vi "SISE-Analyser110.vi"() -> ()   [LabVIEW 2024]
uses:
  <vilib>/Analysis/NI_AALPro.lvlib
panel:
  in  "Ion conc. ch1 (mM) 2":dbl
  in  "Main Tab Control":T1(tab)
  out "Event marks":string
  in  "Raw data file in":path
  out "Trace length":dbl
  out "# of traces":dbl
  out "Trace #":dbl
  in  "Scroll back":bool
  in  "Step back":bool
  in  "Step forward":bool
  in  "Scroll forward":bool
  in  "Module selection view data":enum16{"Load data", "Scroll data"}(ring)
  out "Load data":bool
  in  "Scroll speed":dbl(slide)=10.000000000000002 scale=1.0..100.0
  out "Scroll data":bool
  out "SISE 1 channel":bool
  out "Voltage 2 channel":bool
  out "Voltage 1 channel":bool
  out "SISE 2 channel":bool
  out "Scan distance, µm":dbl
  out "Scan angle, degrees":dbl
  out "Record period (single track), s):":dbl
  out "Position probe":cluster{dbl[], dbl[]}[](graph)
  in  "?":T2(tab)
  out "Vprobe SISE 1":cluster{dbl[], dbl[]}[](graph)
  out "Vprobe SISE 2":cluster{dbl[], dbl[]}[](graph)
  out "Vprobe V 1":cluster{dbl[], dbl[]}[](graph)
  out "Vprobe V 2":cluster{dbl[], dbl[]}[](graph)
  in  "?":enum32{"dV SISE 1", "dV SISE 2"}(tab)
  out "deltaV SISE 1":cluster{dbl[], "Best Linear Fit":dbl[]}[](graph)
  out "deltaV SISE 2":cluster{dbl[], "Best Linear Fit":dbl[]}[](graph)
  in  "Start fit (% of rec. period)":dbl(slide)=50.0 scale=0.0..100.0
  in  "TC 3":T3(tab)
  in  "Range limit\nS1.1 (mV)":dbl(slide)=200.0 min=0.0 max=600.0 scale=0.2..600.0
  in  "Base line\nS1.1 (mV)":dbl(slide) scale=-300.0..300.0
  in  "Range limit\nS1.2 mV":dbl(slide)=30.0 scale=0.03..300.0
  in  "Base line \nS1.2 (mV)":dbl(slide) scale=-15.0..15.0
  out "dV-SISE channel 1":cluster{dbl[], dbl[]}[](graph)
  out "V-SISE channel 1":cluster{dbl[], dbl[]}[](graph)
  out "dV-SISE channel 2":cluster{dbl[], dbl[]}[](graph)
  in  "Base line \nS2.2 (mV)":dbl(slide) scale=-15.0..15.0
  in  "Range limit\nS2.2 (mV)":dbl(slide)=30.0 scale=0.03..300.0
  out "V-SISE channel 2":cluster{dbl[], dbl[]}[](graph)
  in  "Range limit\nS1.1 (mV) 2":dbl(slide)=200.0 min=0.0 max=600.0 scale=0.2..600.0
  in  "Base line\nS1.1 (mV)":dbl(slide) scale=-300.0..300.0
  out "Voltage channel 1":cluster{dbl[], dbl[]}[](graph)
  in  "Base line\nV1 (V)":dbl(slide) scale=-300.0..300.0
  in  "Range limit\nV1 (V)":dbl(slide)=200.0 min=0.0 max=600.0 scale=0.2..600.0
  in  "Base line\nV2 (V)":dbl(slide) scale=-300.0..300.0
  in  "Range limit\nV2 (V)":dbl(slide)=200.0 min=0.0 max=600.0 scale=0.2..600.0
  out "Voltage channel 2":cluster{dbl[], dbl[]}[](graph)
  in  "Zoom from end":dbl(slide)=100.0 scale=0.0..100.0
  in  "Zoom from start":dbl(slide) scale=0.0..100.0
  in  "Calibration-channel SISE1/2":enum32{"SISE channel 1", "SISE channel 2"}(tab)
  out "Update graphs ch1":bool
  in  "Module selection (Calibration window channel 1)":T4(ring)
  out "Anal. method ch1":bool
  out "Calibration ch1":bool
  out "Slope ch1":dbl
  out "Intercept ch1":dbl
  out "?":cluster{dbl[], dbl[]}[](graph)
  out "Point #":dbl[](array[numeric])=[1.0, 2.0, 3.0, 4.0, 5.0]
  in  "Array in":dbl[][](array[numeric])
  out "Geometry ch1":bool caption="Geometry"
  out "Corrected \ndistance ch1":dbl caption="Corrected \ndistance"
  in  "Tab Control Geo 1":enum32{"flat surface", "cylinder", "sphere"}(tab)
  in  "Scan Distance  Flat (µm) 1":dbl
  in  "Scan distance cyl. (µm) 1":dbl caption="Scan distance cyl. (µm)"
  in  "Radius of object cyl. (µm) 1":dbl caption="Radius of object cyl. (µm)"
  in  "Minimum distance to object cyl. (µm) 1":dbl caption="Minimum distance to object cyl. (µm)"
  in  "Minimum distance to object sphere (µm) 1":dbl caption="Minimum distance to object sphere (µm)"
  in  "Radius of object sphere (µm) 1":dbl caption="Radius of object sphere (µm)"
  in  "Scan distance sphere (µm) 1":dbl caption="Scan distance sphere (µm)"
  out "Ion conc. SISE channel 1":cluster{dbl[], dbl[]}[](graph)
  in  "Range limit\nS1.3 (mM)":dbl(slide)=200.0 min=0.0 max=600.0 scale=1e-08..100.0
  in  "Base line\nS1.3 (mM)":dbl(slide) scale=-10.0..10.0
  out "Ion flux SISE channel 1":cluster{dbl[], dbl[]}[](graph)
  in  "Base line \nS1.4":dbl(slide) scale=-15.0..15.0
  in  "Range limit\nS1.4":dbl(slide)=1080.8651170969697 scale=0.03..3000.0
  out "?":string
  in  "Bildlaufleiste":i32(c297)
  in  "Zoom from end (Cal. modul) ch1":dbl(slide)=100.0 caption="Zoom from end" scale=0.0..100.0
  in  "Zoom from start (Cal. modul) ch1":dbl(slide) caption="Zoom from start" scale=0.0..100.0
  in  "Analysis method (Calibration window channel 1)":enum32{"Chem. potential", "Diff. gradient"}(tab)
  in  "Ion conc. ch1 (mM)":dbl
  out "Valence ch1":dbl
  out "Ion mobilty ch1":dbl
  out "Diff. coeff. ch1":dbl
  in  "Ion Species ch1":u16(ring) items=["none", "H+", "K+", "NH4+", "Na+", "Cl-", "NO3-", "Ca2+", "Mg2+"]
  out "Update graphs ch2":bool
  out "Calibration ch2":bool
  out "Slope ch2":dbl
  out "Intercept ch2":dbl
  out "?":cluster{dbl[], dbl[]}[](graph)
  out "Point # 2":dbl[](array[numeric])=[1.0, 2.0, 3.0, 4.0, 5.0]
  in  "Array in 2":dbl[][](array[numeric])
  out "Geometry 2":bool caption="Geometry"
  out "Corrected \ndistance ch2":dbl caption="Corrected\ndistance"
  in  "Tab Control Geo 2":enum32{"flat surface", "cylinder", "sphere"}(tab)
  in  "Scan Distance  Flat (µm) 2":dbl caption="Scan Distance  Flat (µm)"
  in  "Scan distance cyl. (µm) 2":dbl caption="Scan distance cyl. (µm)"
  in  "Radius of object cyl. (µm) 2":dbl caption="Radius of object cyl. (µm)"
  in  "Minimum distance to object cyl. (µm) 2":dbl caption="Minimum distance to object cyl. (µm)"
  in  "Minimum distance to object sphere (µm) 2":dbl caption="Minimum distance to object sphere (µm)"
  in  "Radius of object sphere (µm) 2":dbl caption="Radius of object sphere (µm)"
  in  "Scan distance sphere (µm) 2":dbl caption="Scan distance sphere (µm)"
  in  "Bildlaufleiste 2":i32(c297)
  out "?":string
  out "Ion conc. SISE channel 2":cluster{dbl[], dbl[]}[](graph)
  in  "Range limit\nS2.3 (mM)":dbl(slide)=200.0 min=0.0 max=600.0 scale=1e-08..100.0
  in  "Base line\nS2.3 (mM)":dbl(slide) scale=-10.0..10.0
  out "Ion flux SISE channel 2":cluster{dbl[], dbl[]}[](graph)
  in  "Base line \nS2.4":dbl(slide) scale=-15.0..15.0
  in  "Range limit\nS2.4":dbl(slide)=1021.2709042717592 scale=0.03..3000.0
  in  "Module selection (Calibration window channel 2)":T4(ring)
  in  "Zoom from end (Cal. modul) 2":dbl(slide)=100.0 caption="Zoom from end" scale=0.0..100.0
  in  "Zoom from start (Cal. modul) 2":dbl(slide) caption="Zoom from start" scale=0.0..100.0
  in  "Analysis method (Calibration window channel 2)":enum32{"Chem. potential", "Diff. gradient"}(tab)
  in  "Ion conc. ch2 (mM)":dbl
  out "Valence ch2":dbl
  out "Ion mobilty ch2":dbl
  out "Diff. coeff. ch2":dbl
  in  "Ion Species ch2":u16(ring) items=["none", "H+", "K+", "NH4+", "Na+", "Cl-", "NO3-", "Ca2+", "Mg2+"]
  out "Anal. method ch2":bool
  in  "SISE channel selection (buffer corr.)":T5(tab)
  out "Tab Control":enum32{"Chem. potential", "Diff. gradient"}(tab)
  out "Buffer Mobilty ch1":dbl
  out "Diff. coeff. buffer ch1":dbl
  in  "Module selection ch1 (buffer corr.)":T6(ring)
  out "Buffer species ch1":bool
  out "Buffer conc. ch1":bool
  in  "Select buffer ch1":T7(ring)
  out "pKs ch1":dbl
  in  "Buffer conc. ch1 (mM)":dbl
  out "?":string
  in  "Bildlaufleiste 3":i32(c297)
  out "Ion flux (buffer corr.) SISE channel 1":cluster{dbl[], dbl[]}[](graph)
  in  "Base line \nS2.4 3":dbl(slide) scale=-15.0..15.0
  in  "Range limit\nS2.4 3":dbl(slide)=30.0 scale=0.01..10000.0
  out "Update graphs (buffer corr.) ch1":bool
  in  "Zoom from end (Buffer corr. modul) ch1":dbl(slide)=100.0 caption="Zoom from end" scale=0.0..100.0
  in  "Zoom from start (Buffer corr. modul) ch1":dbl(slide) caption="Zoom from start" scale=0.0..100.0
  in  "Module selection ch2 (buffer corr.)":T6(ring)
  out "Buffer species ch2":bool
  out "Buffer conc. ch2":bool
  in  "Buffer conc. ch2 (mM)":dbl
  in  "Range limit\nS2.4 2":dbl(slide)=30.0 scale=0.01..10000.0
  in  "Base line \nS2.4 2":dbl(slide) scale=-15.0..15.0
  out "Ion flux (buffer corr.) SISE channel 2":cluster{dbl[], dbl[]}[](graph)
  out "Update graphs (buffer corr.) ch2":bool
  out "?":string
  in  "Bildlaufleiste 4":i32(c297)
  in  "Zoom from start (Buffer corr. modul) ch2":dbl(slide) caption="Zoom from start" scale=0.0..100.0
  in  "Zoom from end (Buffer corr. modul) ch2":dbl(slide)=100.0 caption="Zoom from end" scale=0.0..100.0
  in  "Select buffer ch 2":T7(ring)
  out "pKs ch2":dbl
  out "Tab Control 2":enum32{"Chem. potential", "Diff. gradient"}(tab)
  out "Buffer Mobilty ch2":dbl
  out "Diff. coeff. buffer ch2":dbl
  out "Next data file/exit program":bool
  in  "Exit program":bool
  out "Create analysis file":bool
  out "Indicate output":bool[](array[boolean])
  in  "Select output":bool[](array[boolean])=[TRUE, TRUE, TRUE, TRUE, TRUE, TRUE, TRUE, TRUE, TRUE, TRUE, TRUE, TRUE, TRUE, TRUE]
  in  "Analysis output file":path
  out "Raw data file":path
  out "Cluster 3":cluster{string[], bool[]}
  in  "Next data file":bool
  in  "Save data":bool
  out "Save analyses file":bool
  in  "Module selection Save Data":T8(ring)
  # "Event marks"
  # "Point (#)       Conc. (mM )      Vm (mV)"
  # "Event marks"
  # "Point (#)       Conc. (mM )      Vm (mV)"
  # "Event marks"
  # "Event marks"
  # "Output signals available                                                               Select output signals"
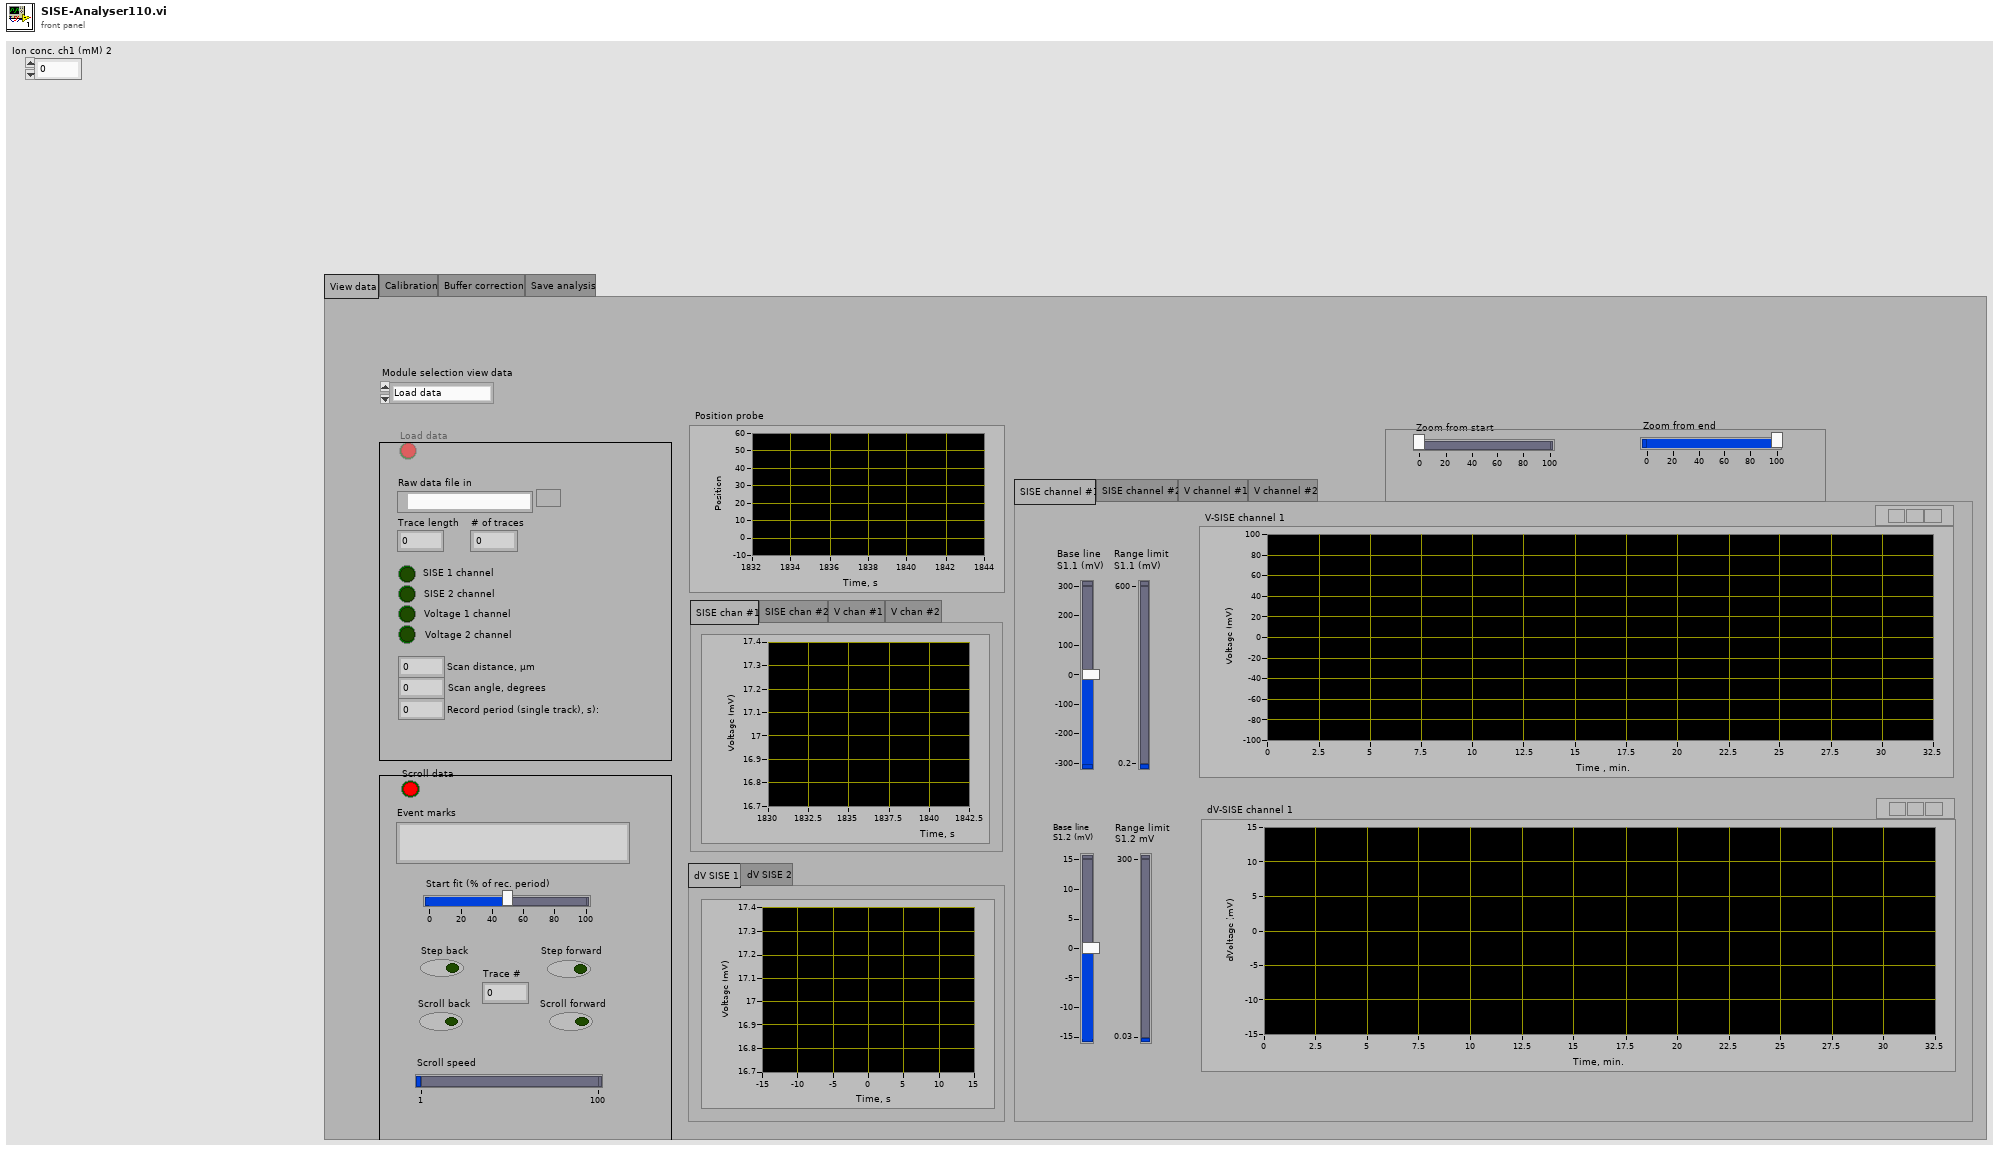
[diagram p1: front panel]
types:
  T1 = enum32{"View data", "Calibration", "Buffer correction", "Save analysis"}
  T2 = enum32{"SISE chan #1", "SISE chan #2", "V chan #1", "V chan #2"}
  T3 = enum32{"SISE channel #1", "SISE channel #2", "V channel #1", "V channel #2"}
  T4 = enum16{"Analysis method", "Calibrate", "Geometry", "Update graphs"}
  T5 = enum32{"SISE channel 1, buffer corr.", "SISE channel 2, buffer corr."}
  T6 = enum16{"Buffer species", "Buffer conc.", "Update graphs"}
  T7 = enum16{"none", "Mes", "Malate (pH 5)", "Citrate (pH 5)", "TRIS", "HEPES"}
  T8 = enum16{"Create analysis file", "Save data", "New/stop analysis"}
  T9 = enum8{"Enabled", "Disabled", "Disabled and Grayed Out"}
  T10 = enum16{"open", "replace", "create", "open or create", "replace or create", "replace or create with confirmation"}
  T11 = enum32{"Chem. potential", "Diff. gradient", "empty loop"}
  T12 = cluster{path, "Referenz (Ausgang)":refnum<file>, bool, i32, string}
  T13 = cluster{path, "Referenz (Ausgang)":refnum<file>, bool, i32, string}[]
  T14 = cluster{"Raw data file in":path, "refnum out":refnum<file>, "status":bool, "code":i32, "source":string}
  T15 = cluster{bool[], dbl[][], dbl[], cluster{string[], bool[]}, dbl[][], cluster{dbl, string}[]}
  T16 = cluster{dbl[], dbl[], "Best Linear Fit":dbl[], dbl[], dbl[]}
  T17 = cluster{"Array (Ausgang)":dbl[], "Array (Ausgang)":dbl[]}
  T18 = cluster{"Array (Ausgang)":dbl[], "Array (Ausgang)":dbl[]}[]
  T19 = cluster{"dup path":path, "refnum":refnum<file>, "status":bool, "code":i32, "source":string}
  T20 = cluster{bool[], dbl[][], dbl[], cluster{dbl, string}[]}
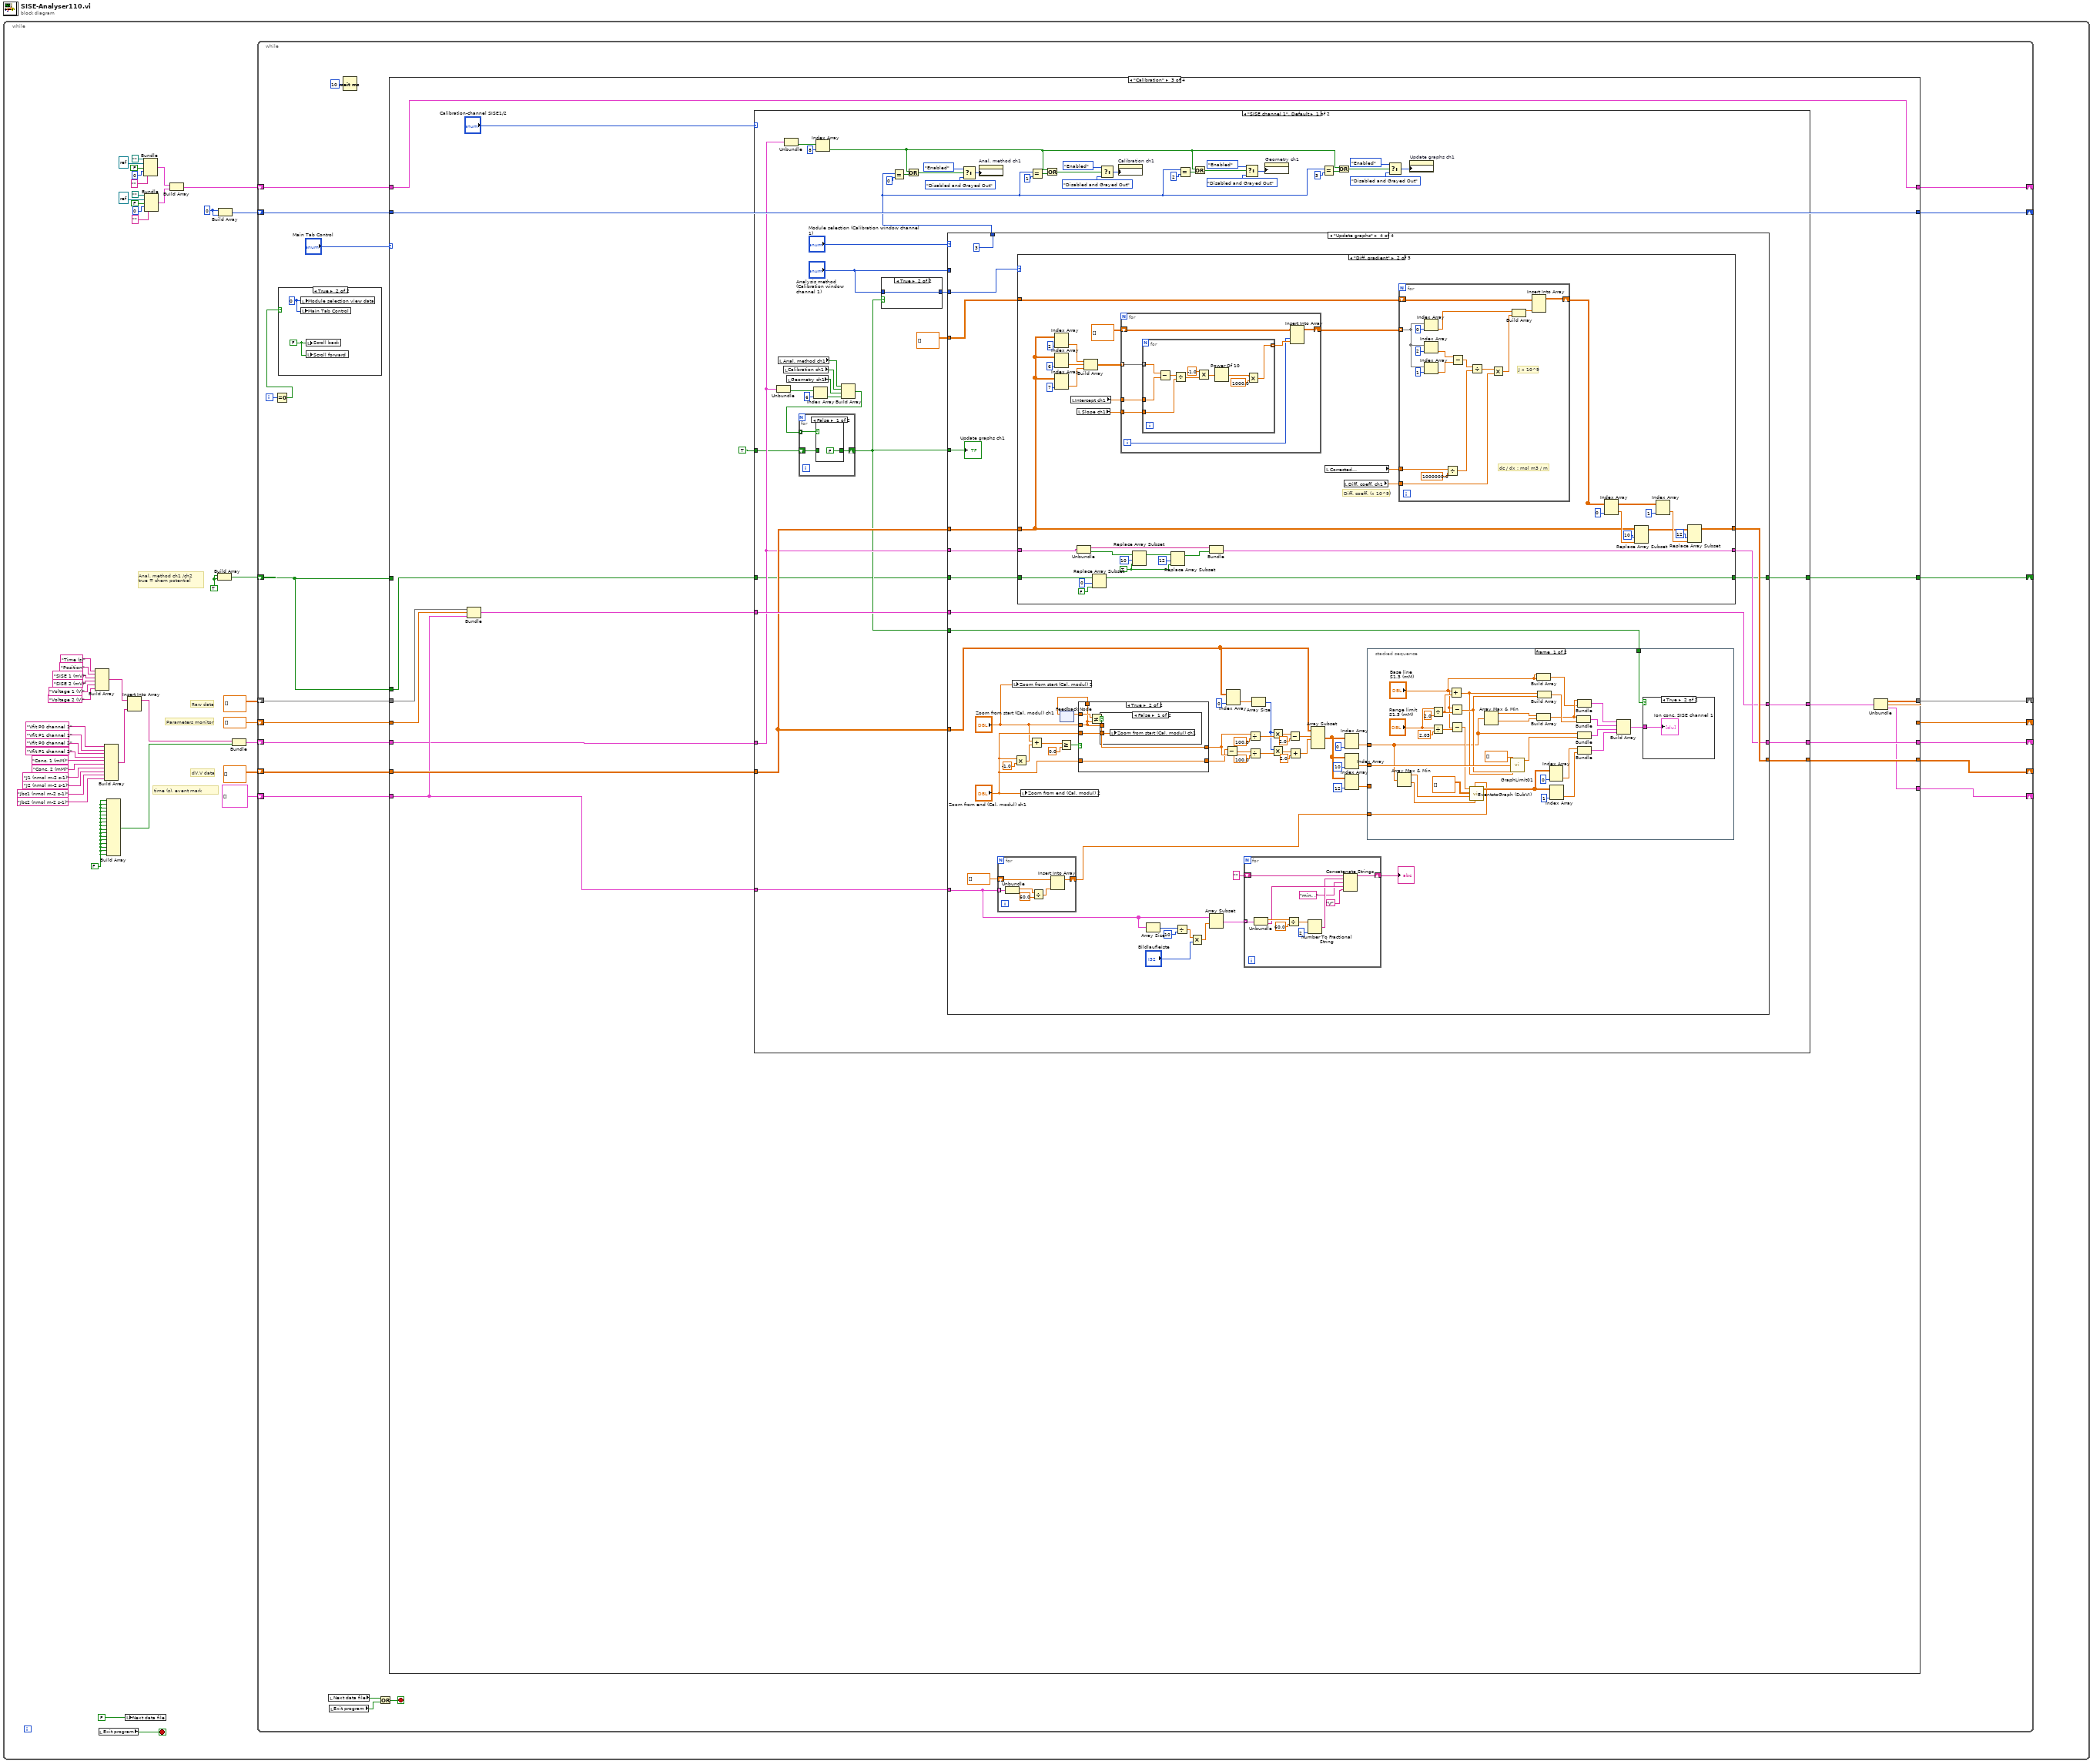
[diagram p0: block diagram]
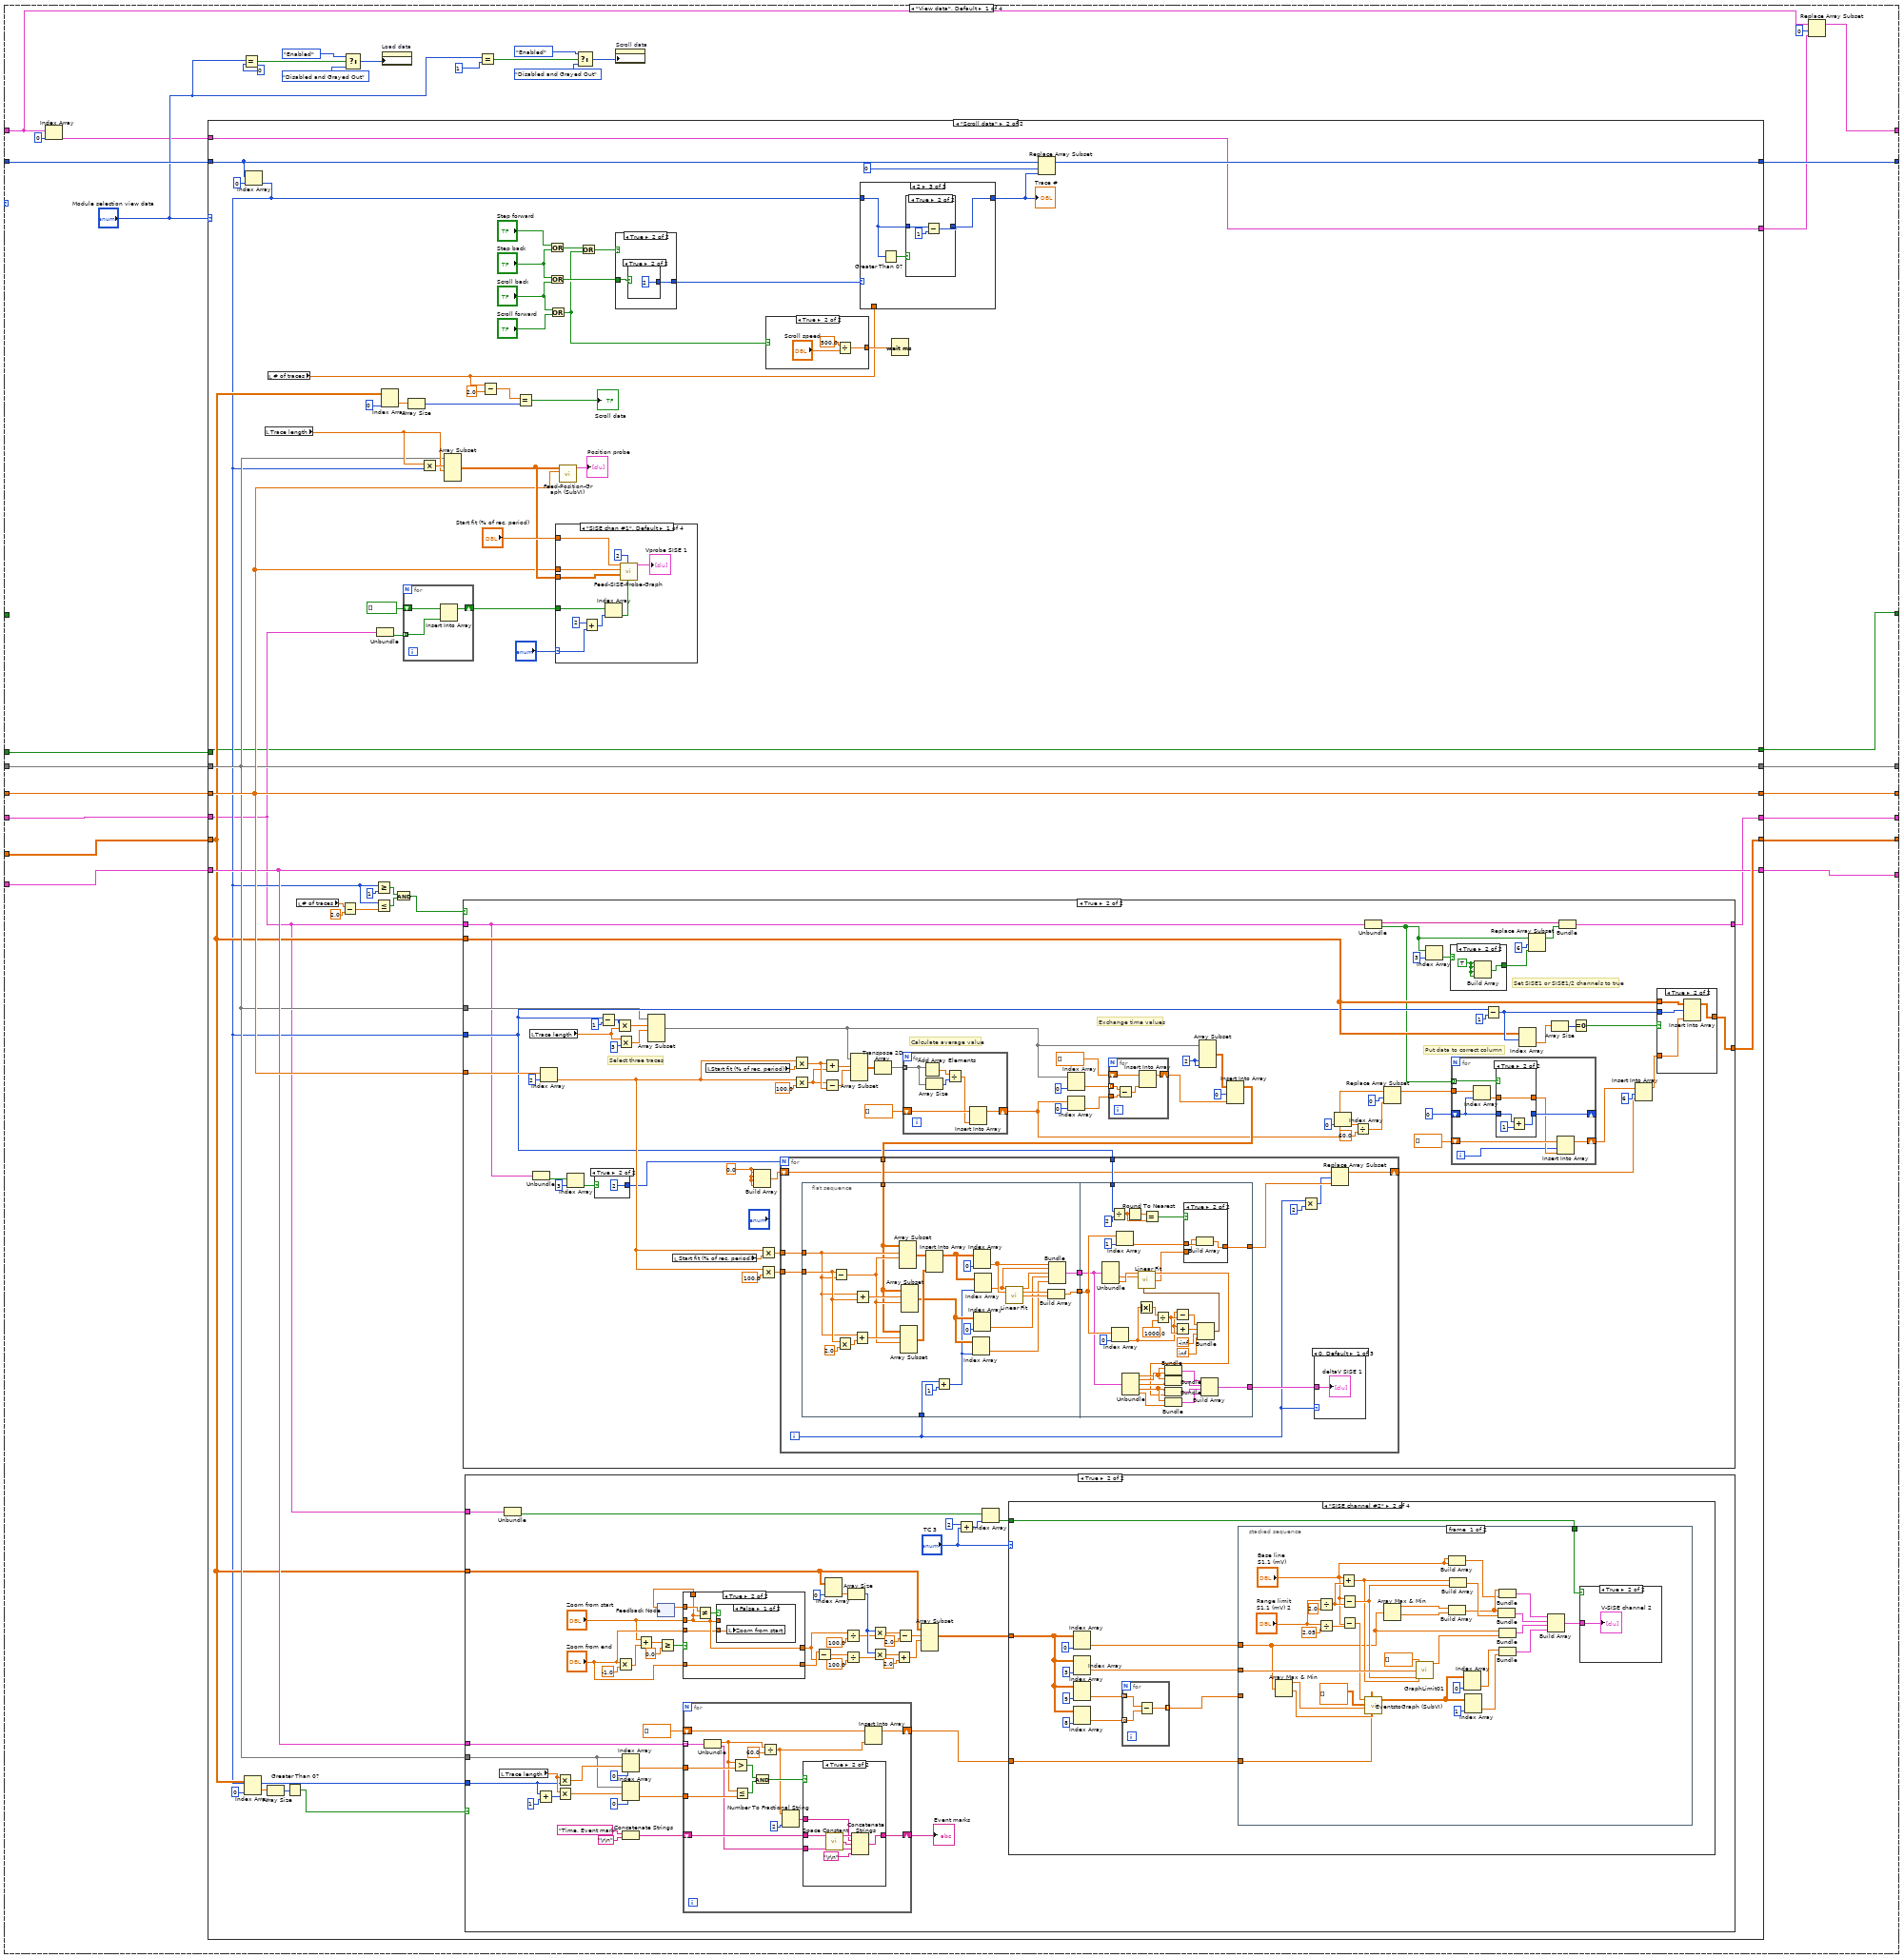
[diagram p3: hidden frame]
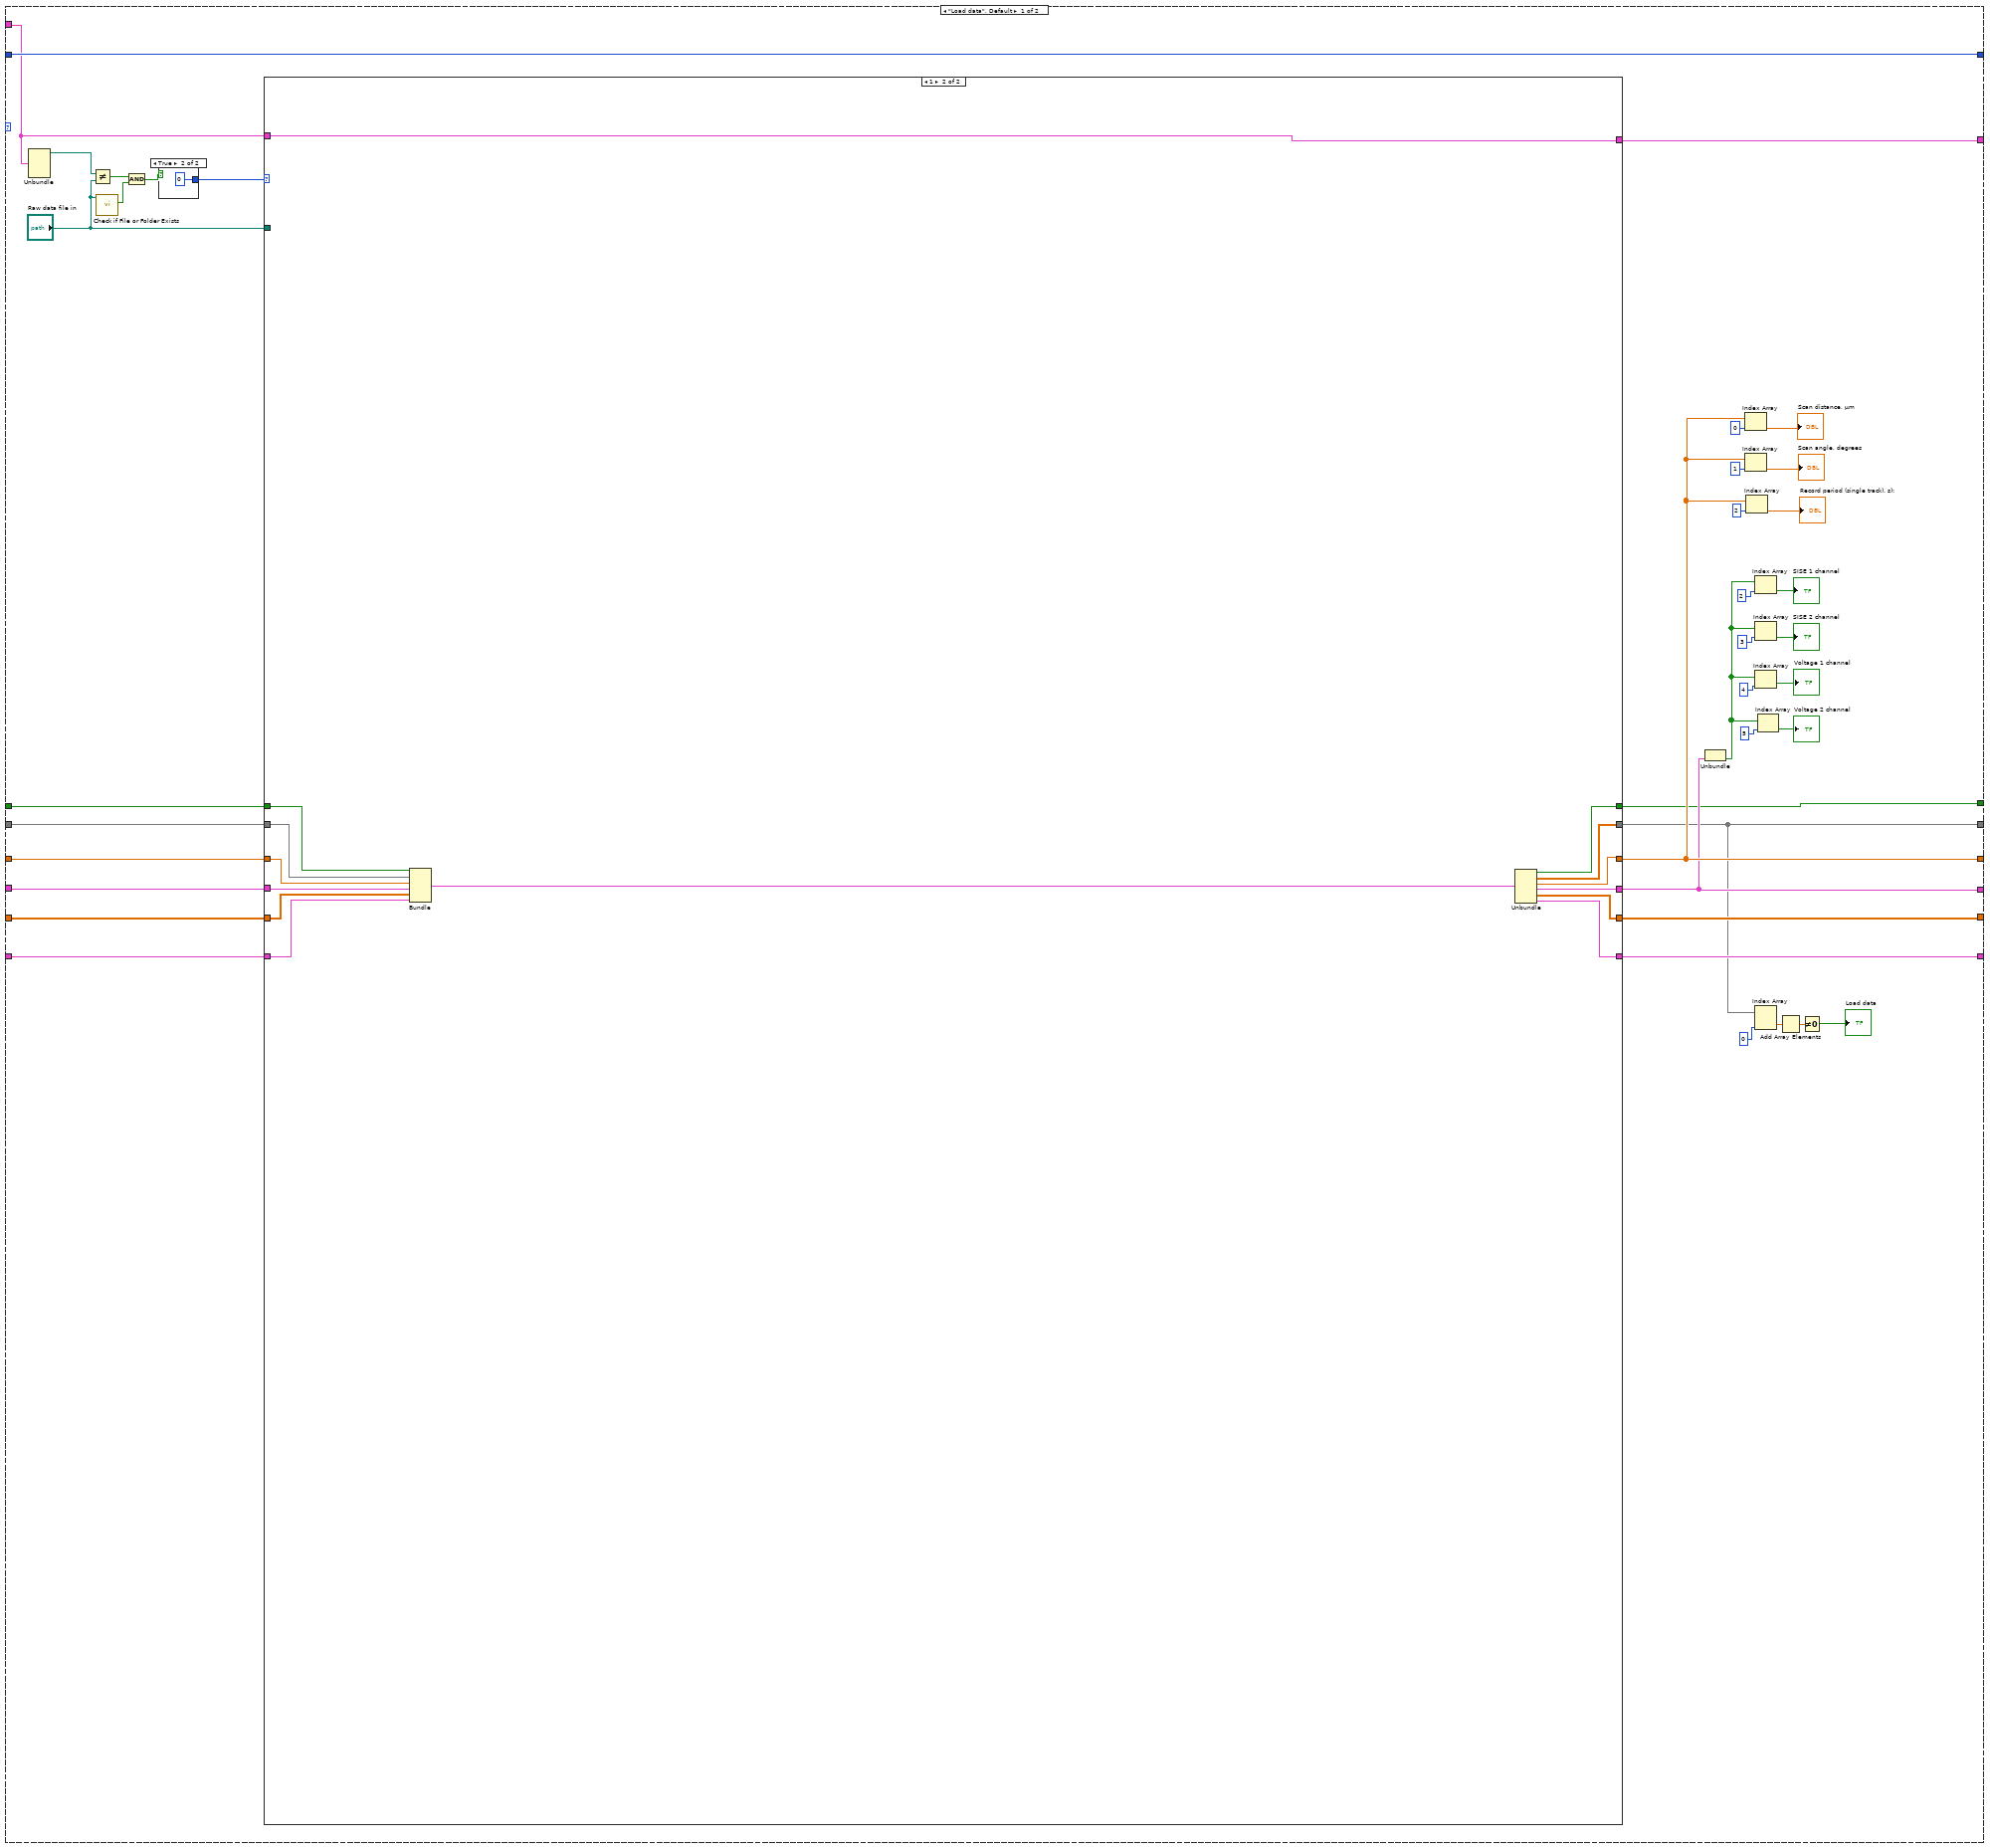
[diagram p4: hidden frame]
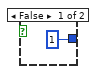
[diagram p5: hidden frame]
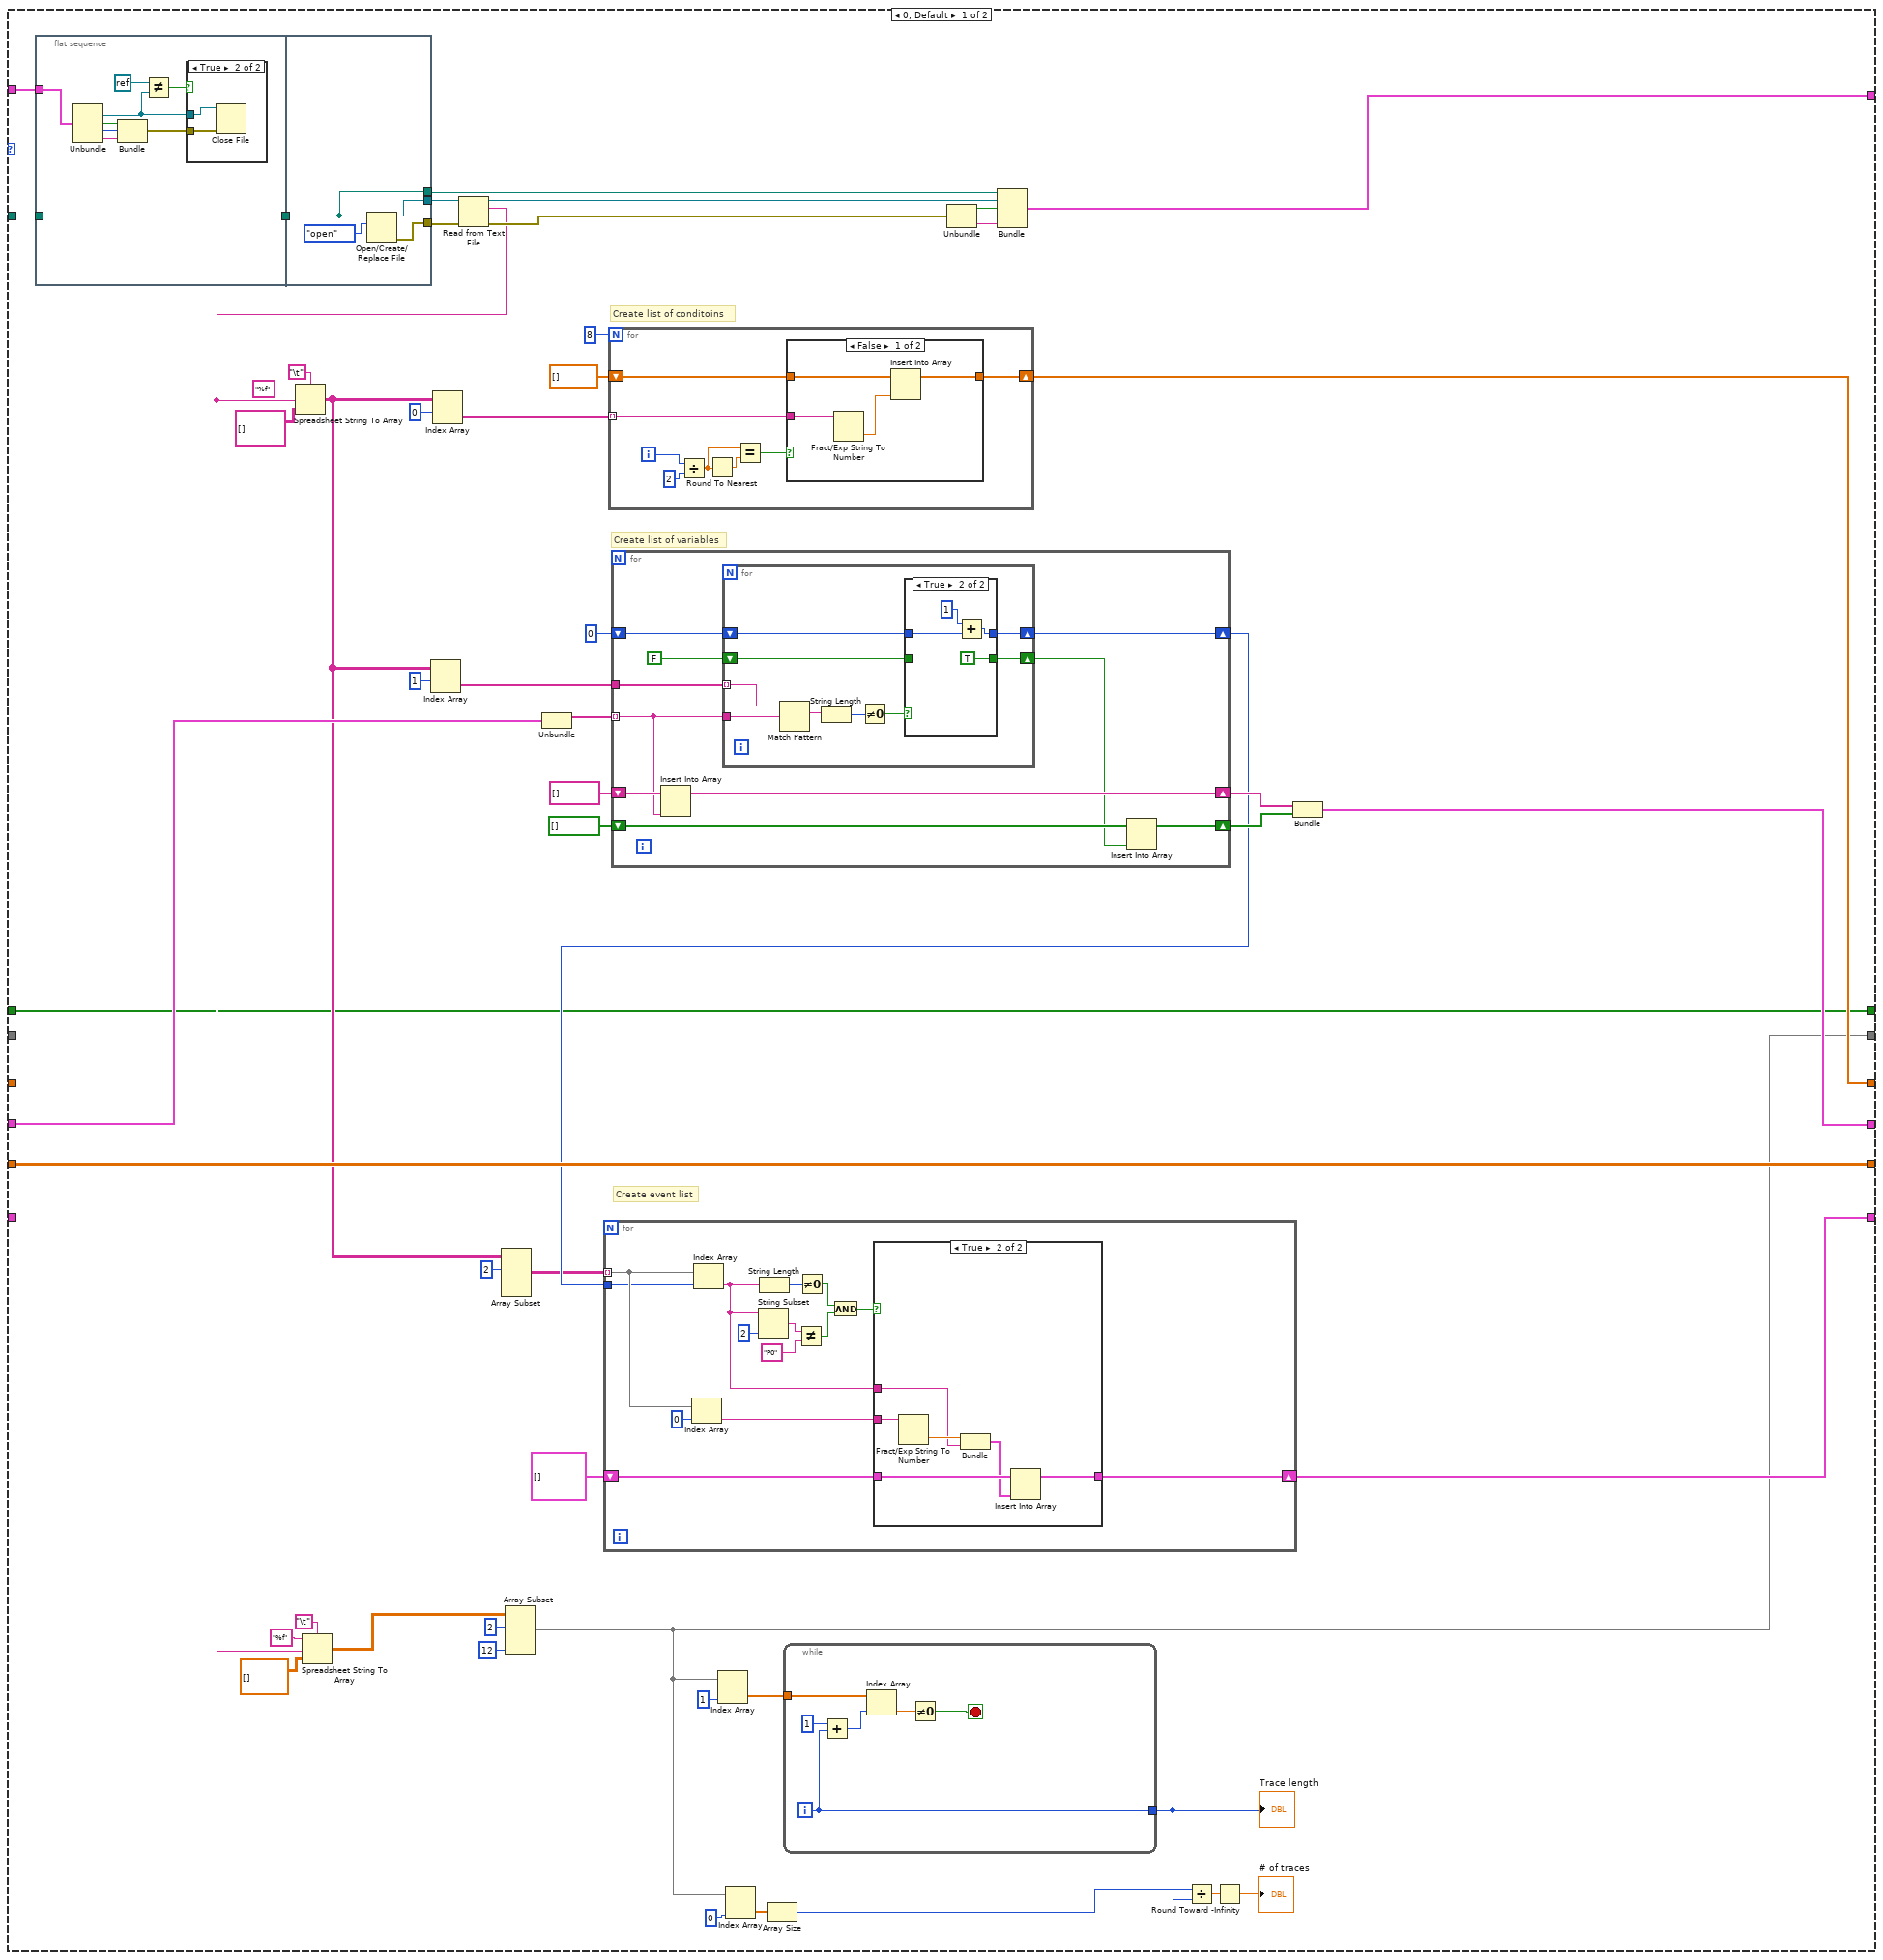
[diagram p6: hidden frame]
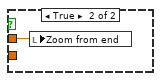
[diagram p13: hidden frame]
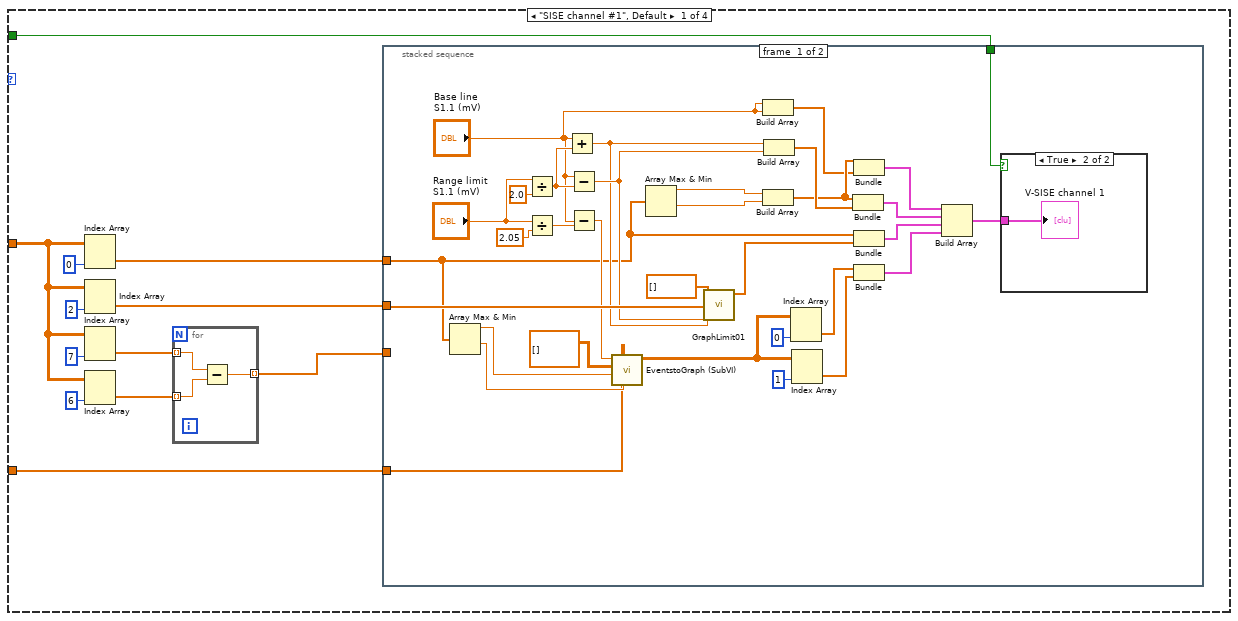
[diagram p14: hidden frame]
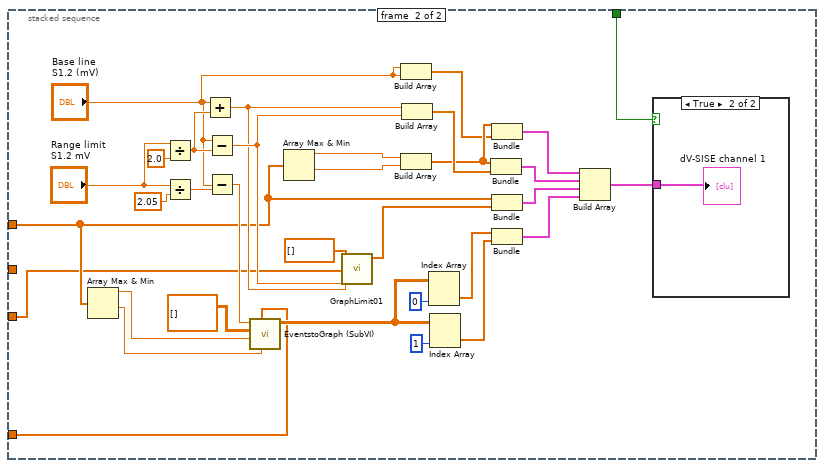
[diagram p16: hidden frame]
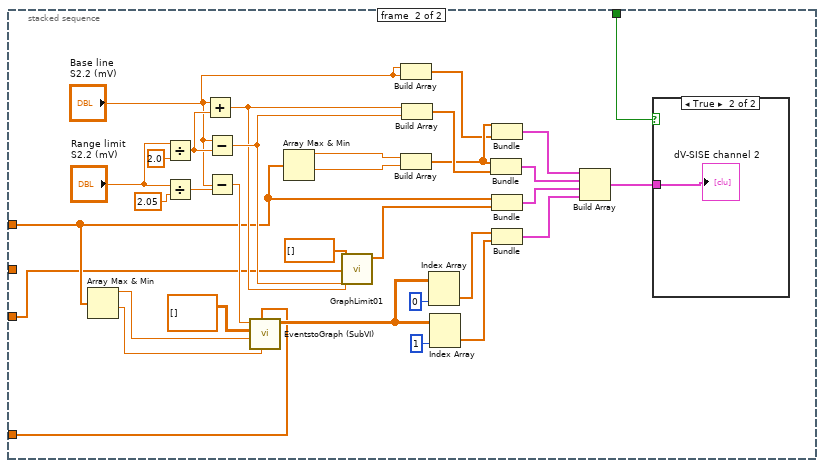
[diagram p19: hidden frame]
diagram:
  n1 = while {
    stop <- w25 stop-if-true
    w2 = TRUE
    w3 = FALSE
    w24 = 0
    # "Anal. method ch1 /ch2\ntrue = chem potential"
    # "time (s), event mark"
    # "Parameters monitor"
    # "dV,V data"
    # "Raw data"
    n2 = Build Array("Time (s)", "Position", "SISE 1 (mV)", "SISE 2 (mV)", "Voltage 1 (V)", "Voltage 2 (V)") -> (w33:string[])
    n3 = local read "Exit program"() -> (w25:bool)
    n4 = Build Array("Vfit P0 channel 1", "Vfit P1 channel 1", "Vfit P0 channel 2", "Vfit P1 channel 2", "Conc. 1 (mM)", "Conc. 2 (mM)", "J1 (nmol m-2 s-1)", "J2 (nmol m-2 s-1)", "Jbc1 (nmol m-2 s-1)", "Jbc2 (nmol m-2 s-1)") -> (w32:string[])
    n5 = Build Array(w3, w3, w3, w3, w3, w3, w3, w3, w3, w3, w3, w3, w3, w3, w3, w3) -> (w26:bool[])
    n6 = local write "Next data file"(FALSE) -> ()
    n7 = Insert Into Array(array=w33, new element=w32) -> (w27:string[])  [unwired: 1 in]
    n8 = Bundle(path "", "Referenz (Ausgang)"=refnum<file> refnum, FALSE, 0, "") -> (w12:T12)  [unwired: 1 in]
    n9 = Bundle(path "", "Referenz (Ausgang)"=refnum<file> refnum, FALSE, 0, "") -> (w11:T12)  [unwired: 1 in]
    n10 = Build Array(w12, w11) -> (w10:T13)
    n11 = Build Array(w2, w2) -> (w1:bool[])
    n12 = Build Array(w24, w24) -> (w23:i32[])
    n13 = Bundle(w27, w26) -> (w41:cluster{string[], bool[]})  [unwired: 1 in]
    n14 = while {
      shift-right: [w49] -> _
      shift-left: dbl[][] [] -> [w46]
      shift-right: [w66] -> _
      shift-left: dbl[][] [] -> [w67]
      shift-right: [w65] -> _
      shift-left: w41 -> [w50]
      shift-right: [w64] -> _
      shift-left: dbl[] [] -> [w63]
      shift-right: [w59] -> _
      shift-left: w23 -> [w54]
      shift-right: [w62] -> _
      shift-left: cluster{dbl, string}[] [] -> [w61]
      shift-right: [w51] -> _
      shift-left: w10 -> [w60]
      shift-right: [w48] -> _
      shift-left: w1 -> [w47]
      i -> [w53]
      stop <- w58 stop-if-true
      n15 = Equal To 0?(x=w53) -> (x = 0?=w52:bool)
      n16 = case shown="True" w52 {
        frame False {
        }
        frame True {
          w69 = FALSE
          w70 = 0
          n17 = local write "Main Tab Control"(w70) -> ()
          n18 = local write "Module selection view data"(w70) -> ()
          n19 = local write "Scroll back"(w69) -> ()
          n20 = local write "Scroll forward"(w69) -> ()
        }
      }
      n21 = local read "Next data file"() -> (w57:bool)
      n22 = local read "Exit program"() -> (w56:bool)
      n23 = Wait (ms)(milliseconds to wait=u32 10) -> ()  [unwired: 1 out]
      n24 = Or(x=w57, y=w56) -> (x .or. y?=w58:bool)
      n25 = case shown="\"Calibration\"" "Main Tab Control" {
        tunnel: w46 -> [w101 w959 w1197 w2103]
        tunnel: [w100 w931 w1203 w2111] -> w49
        tunnel: w67 -> [w84 w962 w1202 w2109]
        tunnel: [w89 w928 w1199 w2098] -> w66
        tunnel: w50 -> [w74 w960 w1193 w2096]
        tunnel: [w73 w930 w1194 w2110] -> w65
        tunnel: w63 -> [w88 w961 w1196 w2108]
        tunnel: [w87 w929 w1198 w2100] -> w64
        tunnel: w54 -> [w83 w951 w1191 w2105]
        tunnel: w61 -> [w75 w958 w1195 w2107]
        tunnel: [w86 w932 w1190 w2101] -> w62
        tunnel: w60 -> [w79 w937 w1192 w2104]
        tunnel: [w77 w935 w1192 w2104] -> w51
        tunnel: [w85 w951 w1191 w2105] -> w59
        tunnel: w47 -> [w72 w927 w1188 w2102]
        tunnel: [w71 w926 w1187 w2099] -> w48
        tunnel: w47 -> [_ _ _ w2095]
        frame "View data", Default {
          n26 = Index Array(array=w79, index=0 ("Index")) -> (element=w80:T12)
          n27 = case shown="\"Scroll data\"" "Module selection view data" {
            tunnel: w101 -> [w115 w302]
            tunnel: [w114 w320] -> w100
            tunnel: w84 -> [w137 w314]
            tunnel: [w113 w314] -> w89
            tunnel: w74 -> [w104 w293]
            tunnel: [w121 w301] -> w73
            tunnel: w88 -> [w132 w321]
            tunnel: [w128 w321] -> w87
            tunnel: w83 -> [w124 w297]
            tunnel: [w124 w298] -> w85
            tunnel: w75 -> [w123 w315]
            tunnel: [w122 w315] -> w86
            tunnel: w80 -> [w109 w294]
            tunnel: [w110 w294] -> w76
            tunnel: w72 -> [w103 w292]
            tunnel: [w102 w292] -> w71
            frame "Load data", Default {
              n28 = Unbundle(w109) -> (w107:path)  [unwired: 4 out]
              n29 = Not Equal?(x=w107, y="Raw data file in") -> (x != y?=w112:bool)
              n30 = call <vilib>:"Check if File or Folder Exists.vi"("path"="Raw data file in") -> ("file or folder exists?"=w111:bool)  [unwired: 8 in, 2 out]
              n31 = And(x=w112, y=w111) -> (x .and. y?=w105:bool)
              n32 = case shown="True" w105 {
                tunnel: [1 0] -> w106
                frame False {
                }
                frame True {
                }
              }
              n33 = case shown="1" w106 {
                tunnel: w137 -> [_ w289]
                tunnel: [w147 w279] -> w113
                tunnel: w104 -> [w170 w291]
                tunnel: [w169 w281] -> w121
                tunnel: w132 -> [_ w290]
                tunnel: [w178 w280] -> w128
                tunnel: w123 -> [_ w287]
                tunnel: [w166 w283] -> w122
                tunnel: w115 -> [w197 w288]
                tunnel: [w197 w282] -> w114
                tunnel: "Raw data file in" -> [w194 _]
                tunnel: [w190 w285] -> w110
                tunnel: w109 -> [w196 w285]
                tunnel: w103 -> [w144 w284]
                tunnel: [w144 w278] -> w102
                frame 0, Default {
                  # "Create list of variables"
                  # "Create list of conditoins"
                  # "Create event list"
                  n34 = flat-sequence {
                    tunnel: w196 -> [w271]
                    tunnel: [w263] -> w195
                    tunnel: w194 -> [w263]
                    tunnel: [w275] -> w187
                    tunnel: [w276] -> w188
                    tunnel: w195 -> [w274]
                    tunnel: [w274] -> w189
                    frame #0 {
                      n35 = Unbundle(w271) -> ("Referenz (Ausgang)"=w264:refnum<file>, w268:bool, w269:i32, w270:string)  [unwired: 1 out]
                      n36 = Bundle(w268, w269, w270) -> (w267:errorcluster)  [unwired: 1 in]
                      n37 = Not Equal?(x=refnum<k0> refnum, y=w264) -> (x != y?=w265:bool)
                      n38 = case shown="True" w265 {
                        tunnel: w267 -> [_ w273]
                        tunnel: w264 -> [_ w272]
                        frame False {
                        }
                        frame True {
                          n39 = Close File(refnum=w272, error in=w273) -> ()  [unwired: 2 out]
                        }
                      }
                    }
                    frame #1 {
                      n40 = Open/Create/Replace File(file path (use dialog)=w274, operation (0:open)=T10."open") -> (refnum out=w276:refnum<file>, error out=w275:errorcluster)  [unwired: 4 in, 1 out]
                    }
                  }
                  n41 = Read from Text File(file (use dialog)=w188, error in=w187) -> (refnum out=w185:refnum<file>, text=w165:string, error out=w186:errorcluster)  [unwired: 2 in, 1 out]
                  n42 = Spreadsheet String To Array(delimiter (Tab)="\t", format string="%f", spreadsheet string=w165, array type (2D Dbl)=string[][] []) -> (array=w167:string[][])
                  n43 = Spreadsheet String To Array(delimiter (Tab)="\t", format string="%f", spreadsheet string=w165, array type (2D Dbl)=dbl[][] []) -> (array=w157:dbl[][])
                  n44 = Index Array(array=w167, index (row)=1 ("Index")) -> (element=w145:string[])  [unwired: 1 in]
                  n45 = Index Array(array=w167, index (row)=0 ("Index")) -> (element=w146:string[])  [unwired: 1 in]
                  n46 = Array Subset(array=w167, index (row)=2 ("Index")) -> (w163:string[][])  [unwired: 3 in]
                  n47 = Array Subset(array=w157, index (row)=2 ("index"), length (col)=12 ("Länge")) -> (w147:dbl[][])  [unwired: 2 in]
                  n48 = Unbundle(w170) -> (w175:string[])  [unwired: 1 out]
                  n49 = for {
                    N: 8 -> [_]
                    tunnel: w146 -> [w252] mode=indexing
                    shift-right: [w250] -> w178
                    shift-left: dbl[] [] -> [w251]
                    i -> [w257]
                    n50 = Divide(x=w257, y=2) -> (x/y=w254:dbl)
                    n51 = Round To Nearest(number=w254) -> (nearest integer value=w255:dbl)
                    n52 = Equal?(x=w254, y=w255) -> (x = y?=w253:bool)
                    n53 = case shown="False" w253 {
                      tunnel: w252 -> [w259 _]
                      tunnel: w251 -> [w261 w262]
                      tunnel: [w260 w262] -> w250
                      frame False {
                        n54 = Fract/Exp String To Number(string=w259) -> (number=w258:dbl)  [unwired: 3 in, 1 out]
                        n55 = Insert Into Array(array=w261, new element=w258) -> (w260:dbl[])  [unwired: 1 in]
                      }
                      frame True {
                      }
                    }
                  }
                  n56 = for {
                    tunnel: w175 -> [w228] mode=indexing
                    tunnel: w145 -> [w234]
                    shift-right: [w227] -> w171
                    shift-left: bool[] [] -> [w226]
                    shift-right: [w231] -> w168
                    shift-left: 0 -> [w232]
                    shift-right: [w230] -> w172
                    shift-left: string[] [] -> [w229]
                    n57 = Insert Into Array(array=w229, new element=w228) -> (w230:string[])  [unwired: 1 in]
                    n58 = for {
                      tunnel: w234 -> [w243] mode=indexing
                      tunnel: w228 -> [w242]
                      shift-right: [w237] -> w225
                      shift-left: FALSE -> [w239]
                      shift-right: [w235] -> w231
                      shift-left: w232 -> [w236]
                      n59 = Match Pattern(string=w243, regular expression=w242) -> (match substring=w241:string)  [unwired: 1 in, 3 out]
                      n60 = String Length(string=w241) -> (length=w240:i32)
                      n61 = Not Equal To 0?(x=w240) -> (x != 0?=w238:bool)
                      n62 = case shown="True" w238 {
                        tunnel: w239 -> [w245 _]
                        tunnel: [w245 TRUE] -> w237
                        tunnel: w236 -> [w244 w246]
                        tunnel: [w244 w248] -> w235
                        frame False {
                        }
                        frame True {
                          n63 = Add(x=1 ("y"), y=w246) -> (x+y=w248:i32)
                        }
                      }
                    }
                    n64 = Insert Into Array(array=w226, new element=w225) -> (w227:bool[])  [unwired: 1 in]
                  }
                  n65 = for {
                    tunnel: w163 -> [w208] mode=indexing
                    tunnel: w168 -> [w204]
                    shift-right: [w205] -> w166
                    shift-left: cluster{dbl, string}[] [] -> [w206]
                    n66 = Index Array(array=w208, index=0 ("Index")) -> (element=w207:string)
                    n67 = Index Array(array=w208, index=w204) -> (element=w210:string)
                    n68 = String Subset(string=w210, length (rest)=2 ("Länge (Rest)")) -> (substring=w215:string)  [unwired: 1 in]
                    n69 = String Length(string=w210) -> (length=w217:i32)
                    n70 = Not Equal?(x=w215, y="P0") -> (x != y?=w211:bool)
                    n71 = Not Equal To 0?(x=w217) -> (x != 0?=w213:bool)
                    n72 = And(x=w213, y=w211) -> (x .and. y?=w212:bool)
                    n73 = case shown="True" w212 {
                      tunnel: w210 -> [_ w222]
                      tunnel: w207 -> [_ w224]
                      tunnel: [w218 w221] -> w205
                      tunnel: w206 -> [w218 w220]
                      frame False {
                      }
                      frame True {
                        n74 = Fract/Exp String To Number(string=w224) -> (number=w223:dbl)  [unwired: 3 in, 1 out]
                        n75 = Bundle(w223, w222) -> (w219:cluster{dbl, string})  [unwired: 1 in]
                        n76 = Insert Into Array(array=w220, new element=w219) -> (w221:cluster{dbl, string}[])  [unwired: 1 in]
                      }
                    }
                  }
                  n77 = Index Array(array=w147, index (col)=1 ("disabled index (col)")) -> (element=w154:dbl[])  [unwired: 1 in]
                  n78 = Index Array(array=w147, index (col)=0 ("disabled index (col)")) -> (element=w152:dbl[])  [unwired: 1 in]
                  n79 = Array Size(array=w152) -> (size(s)=w151:i32)
                  n80 = while {
                    tunnel: w154 -> [w203]
                    tunnel: [w198] -> w149
                    i -> [w198]
                    stop <- w199 stop-if-true
                    n81 = Add(x=1, y=w198) -> (x+y=w202:i32)
                    n82 = Index Array(array=w203, index=w202) -> (element=w200:dbl)
                    n83 = Not Equal To 0?(x=w200) -> (x != 0?=w199:bool)
                  }
                  "Trace length" <- w149
                  n84 = Unbundle(w186) -> ("status"=w191:bool, "code"=w192:i32, "source"=w193:string)
                  n85 = Bundle("Raw data file in"=w189, "refnum out"=w185, "status"=w191, "code"=w192, "source"=w193) -> (w190:T14)  [unwired: 1 in]
                  n86 = Divide(x=w151, y=w149) -> (x/y=w150:dbl)
                  n87 = Round Toward -Infinity(1:w150) -> (0:→"# of traces":dbl)
                  n88 = Bundle(w172, w171) -> (w169:cluster{string[], bool[]})  [unwired: 1 in]
                }
                frame 1 {
                  n89 = Bundle(w284, w289, w290, w291, w288, w287) -> (w286:T15)  [unwired: 1 in]
                  n90 = Unbundle(w286) -> (w278:bool[], w279:dbl[][], w280:dbl[], w281:cluster{string[], bool[]}, w282:dbl[][], w283:cluster{dbl, string}[])
                }
              }
              n91 = Unbundle(w121) -> (w120:bool[])  [unwired: 1 out]
              n92 = Index Array(array=w128, index=0) -> (element=→"Scan distance, µm":dbl)
              n93 = Index Array(array=w128, index=1) -> (element=→"Scan angle, degrees":dbl)
              n94 = Index Array(array=w128, index=2) -> (element=→"Record period (single track), s):":dbl)
              n95 = Index Array(array=w120, index=2) -> (element=→"SISE 1 channel":bool)
              n96 = Index Array(array=w113, index (col)=0 ("disabled index (col)")) -> (element=w140:dbl[])  [unwired: 1 in]
              n97 = Index Array(array=w120, index=3) -> (element=→"SISE 2 channel":bool)
              n98 = Index Array(array=w120, index=4) -> (element=→"Voltage 1 channel":bool)
              n99 = Index Array(array=w120, index=5) -> (element=→"Voltage 2 channel":bool)
              n100 = Add Array Elements(numeric array=w140) -> (sum=w139:dbl)
              n101 = Not Equal To 0?(x=w139) -> (x != 0?=→"Load data":bool)
            }
            frame "Scroll data" {
              n102 = Index Array(array=w302, index (col)=0 ("Deaktivierter Index (Spalte)")) -> (element=w312:dbl[])  [unwired: 1 in]
              n103 = Index Array(array=w297, index=0 ("Index")) -> (element=w299:i32)
              n104 = local read "Trace length"() -> (w329:dbl)
              n105 = Array Size(array=w312) -> (size(s)=w311:i32)
              n106 = local read "# of traces"() -> (w319:dbl)
              n107 = Greater Than 0?(x=w311) -> (x > 0?=w310:bool)
              n108 = local read "# of traces"() -> (w303:dbl)
              n109 = Subtract(x=w303, y=2.0) -> (x-y=w307:dbl)
              n110 = Greater Or Equal?(x=w299, y=1) -> (x >= y?=w306:bool)
              n111 = Less Or Equal?(x=w299, y=w307) -> (x <= y?=w305:bool)
              n112 = Unbundle(w293) -> (w309:bool[])  [unwired: 1 out]
              n113 = Index Array(array=w302, index (col)=0 ("Deaktivierter Index (Spalte)")) -> (element=w334:dbl[])  [unwired: 1 in]
              n114 = And(x=w306, y=w305) -> (x .and. y?=w304:bool)
              n115 = for {
                shift-right: [w864] -> w323
                shift-left: bool[] [] -> [w863]
                tunnel: w309 -> [w862] mode=indexing
                n116 = Insert Into Array(array=w863, new element=w862) -> (w864:bool[])  [unwired: 1 in]
              }
              n117 = Array Size(array=w334) -> (size(s)=w317:i32)
              n118 = Multiply(x=w329, y=w299) -> (x*y=w330:dbl)
              n119 = Array Subset(array=w314, index (row)=w330, length (row)=w329) -> (w325:dbl[][])  [unwired: 2 in]
              n120 = case shown="True" w304 {
                tunnel: w314 -> [_ w689]
                tunnel: w299 -> [_ w690]
                tunnel: w321 -> [_ w728]
                tunnel: w302 -> [w669 w692]
                tunnel: [w669 w702] -> w320
                tunnel: w293 -> [w668 w682]
                tunnel: [w668 w678] -> w301
                frame False {
                }
                frame True {
                  w670 = 0.0 ("Element")
                  w714 = 2 ("Index")
                  # "Put data to correct column"
                  # "Set SISE1 or SISE1/2 channels to true"
                  # "Exchange time values"
                  # "Calculate average value"
                  # "Select three traces"
                  n121 = local read "Trace length"() -> (w699:dbl)
                  n122 = Unbundle(w682) -> (w688:bool[])  [unwired: 1 out]
                  n123 = Index Array(array=w728, index=2 ("Index")) -> (element=w715:dbl)
                  n124 = Index Array(array=w688, index=3 ("Index")) -> (element=w687:bool)
                  n125 = case shown="True" w687 {
                    tunnel: [1 2] -> w697
                    frame False {
                    }
                    frame True {
                    }
                  }
                  n126 = Subtract(x=w690, y=1) -> (x-y=w738:i32)
                  n127 = Multiply(x=w738, y=w699) -> (x*y=w737:dbl)
                  n128 = Multiply(x=w699, y=3) -> (x*y=w735:dbl)
                  n129 = Array Subset(array=w689, index (row)=w737, length (row)=w735) -> (w694:dbl[][])  [unwired: 2 in]
                  n130 = local read "Start fit (% of rec. period)"() -> (w719:dbl)
                  n131 = local read "Start fit (% of rec. period)"() -> (w726:dbl)
                  n132 = Build Array(w670, w670, w670, w670) -> (w691:dbl[])
                  n133 = Multiply(x=w715, y=w719) -> (x*y=w717:dbl)
                  n134 = Multiply(x=w715, y=100.0) -> (x*y=w716:dbl)
                  n135 = Multiply(x=w715, y=w726) -> (x*y=w733:dbl)
                  n136 = Multiply(x=w715, y=100.0) -> (x*y=w732:dbl)
                  n137 = Add(x=w733, y=w732) -> (x+y=w734:dbl)
                  n138 = Subtract(x=w732, y=w733) -> (x-y=w730:dbl)
                  n139 = Array Subset(array=w694, index (row)=w734, length (row)=w730) -> (w729:dbl[][])  [unwired: 2 in]
                  n140 = Transpose 2D Array(2D array=w729) -> (transposed array=w676:dbl[][])
                  n141 = for {
                    tunnel: w676 -> [w859] mode=indexing
                    shift-right: [w858] -> w686
                    shift-left: dbl[] [] -> [w857]
                    n142 = Add Array Elements(numeric array=w859) -> (sum=w860:dbl)
                    n143 = Array Size(array=w859) -> (size(s)=w861:i32)
                    n144 = Divide(x=w860, y=w861) -> (x/y=w856:dbl)
                    n145 = Insert Into Array(array=w857, new element=w856) -> (w858:dbl[])  [unwired: 1 in]
                  }
                  n146 = Index Array(array=w694, index (col)=0 ("Deaktivierter Index (Spalte)")) -> (element=w722:dbl[])  [unwired: 1 in]
                  n147 = Index Array(array=w686, index=0 ("Index (Spalte)")) -> (element=w720:dbl)
                  n148 = for {
                    tunnel: w720 -> [w852]
                    shift-right: [w855] -> w711
                    shift-left: dbl[] [] -> [w854]
                    tunnel: w722 -> [w851] mode=indexing
                    n149 = Subtract(x=w851, y=w852) -> (x-y=w853:dbl)
                    n150 = Insert Into Array(array=w854, new element=w853) -> (w855:dbl[])  [unwired: 1 in]
                  }
                  n151 = Array Subset(array=w694, index (col)=w714, length (col)=w714) -> (w713:dbl[][])  [unwired: 2 in]
                  n152 = Insert Into Array(array=w713, index (col)=0 ("Index"), new element=w711) -> (w710:dbl[][])  [unwired: 1 in]
                  n153 = for {
                    N: w697 -> [_]
                    tunnel: w710 -> [w780]
                    tunnel: w716 -> [w779]
                    tunnel: w717 -> [w778]
                    tunnel: w690 -> [w776]
                    shift-right: [w775] -> w693
                    shift-left: w691 -> [w774]
                    i -> [w772]
                    n154 = flat-sequence {
                      tunnel: w780 -> [w791]
                      tunnel: w778 -> [w792]
                      tunnel: w779 -> [w799]
                      tunnel: [w796] -> w782
                      tunnel: [w793] -> w781
                      tunnel: w772 -> [w786]
                      tunnel: w782 -> [w825]
                      tunnel: w781 -> [w829]
                      tunnel: w776 -> [w826]
                      tunnel: [w814] -> w773
                      tunnel: [w813] -> w777
                      frame #0 {
                        n155 = Subtract(x=w799, y=w792) -> (x-y=w805:dbl)
                        n156 = Multiply(x=w799, y=2.0) -> (x*y=w802:dbl)
                        n157 = Add(x=w792, y=w802) -> (x+y=w810:dbl)
                        n158 = Add(x=w792, y=w799) -> (x+y=w809:dbl)
                        n159 = Array Subset(array=w791, index (row)=w792, length (row)=w805) -> (w807:dbl[][])  [unwired: 2 in]
                        n160 = Array Subset(array=w791, index (row)=w810, length (row)=w805) -> (w808:dbl[][])  [unwired: 2 in]
                        n161 = Array Subset(array=w791, index (row)=w809, length (row)=w805) -> (w800:dbl[][])  [unwired: 2 in]
                        n162 = Insert Into Array(array=w807, new element=w808) -> (w803:dbl[][])  [unwired: 2 in]
                        n163 = Add(x=w786, y=1) -> (x+y=w787:i32)
                        n164 = Index Array(array=w800, index (col)=w787) -> (element=w790:dbl[])  [unwired: 1 in]
                        n165 = Index Array(array=w803, index (col)=0 ("disabled index (col)")) -> (element=w798:dbl[])  [unwired: 1 in]
                        n166 = Index Array(array=w800, index (col)=0 ("disabled index (col)")) -> (element=w789:dbl[])  [unwired: 1 in]
                        n167 = Index Array(array=w803, index (col)=w787) -> (element=w797:dbl[])  [unwired: 1 in]
                        n168 = call <vilib>:"Linear Fit.vi"("Y"=w797, "X"=w798) -> ("Best Linear Fit"=w788:dbl[], "slope"=w795:dbl, "intercept"=w794:dbl)  [unwired: 9 in, 2 out]
                        n169 = Build Array(w795, w794) -> (w793:dbl[])
                        n170 = Bundle(w798, w797, "Best Linear Fit"=w788, w789, w790) -> (w796:T16)  [unwired: 1 in]
                      }
                      frame #1 {
                        n171 = Unbundle(w825) -> (w833:dbl[], w834:dbl[])  [unwired: 3 out]
                        n172 = Divide(x=w826, y=2 ("x")) -> (x/y=w827:dbl)
                        n173 = Index Array(array=w829, index=0 ("Index")) -> (element=w835:dbl)
                        n174 = Index Array(array=w829, index=1 ("Index")) -> (element=w812:dbl)
                        n175 = Unbundle(w825) -> (w822:dbl[], w824:dbl[], "Best Linear Fit"=w821:dbl[], w820:dbl[], w818:dbl[])
                        n176 = Round To Nearest(number=w827) -> (nearest integer value=w828:dbl)
                        n177 = Absolute Value(x=w835) -> (abs(x)=w840:dbl)
                        n178 = Equal?(x=w828, y=w827) -> (x = y?=w831:bool)
                        n179 = Divide(x=w840, y=1000.0) -> (x/y=w842:dbl)
                        n180 = Bundle(w822, w824) -> (w823:cluster{dbl[], dbl[]})  [unwired: 1 in]
                        n181 = Bundle(w822, "Best Linear Fit"=w821) -> (w817:cluster{dbl[], "Best Linear Fit":dbl[]})  [unwired: 1 in]
                        n182 = Bundle(w820, w818) -> (w815:cluster{dbl[], dbl[]})  [unwired: 1 in]
                        n183 = Subtract(x=w835, y=w842) -> (x-y=w839:dbl)
                        n184 = Add(x=w835, y=w842) -> (x+y=w838:dbl)
                        n185 = Bundle(w839, w838, -inf, inf) -> (w837:cluster{dbl, dbl, dbl, dbl})  [unwired: 1 in]
                        n186 = call <vilib>:"Linear Fit.vi"("Y"=w834, "X"=w833, "parameter bounds"=w837) -> ("Best Linear Fit"=w819:dbl[], "intercept"=w811:dbl)  [unwired: 8 in, 3 out]
                        n187 = Bundle(w820, "Best Linear Fit"=w819) -> (w816:cluster{dbl[], "Best Linear Fit":dbl[]})  [unwired: 1 in]
                        n188 = case shown="True" w831 {
                          tunnel: w812 -> [w847 w850]
                          tunnel: [w845 w848] -> w814
                          tunnel: w811 -> [w846 w849]
                          frame False {
                            n189 = Build Array(w847, w846) -> (w845:dbl[])
                          }
                          frame True {
                            n190 = Build Array(w849, w850) -> (w848:dbl[])
                          }
                        }
                        n191 = Build Array(w823, w817, w816, w815) -> (w813:cluster{dbl[], "Best Linear Fit":dbl[]}[])
                      }
                    }
                    n192 = Multiply(x=w772, y=2) -> (x*y=w770:i32)
                    n193 = case shown="0, Default" w772 {
                      tunnel: w777 -> [w783 w784 _]
                      frame 0, Default {
                        "deltaV SISE 1" <- w783
                      }
                      frame 1 {
                        "deltaV SISE 2" <- w784
                      }
                      frame 2 {
                      }
                    }
                    n194 = Replace Array Subset(array=w774, new element=w773, index=w770) -> (w775:dbl[])
                  }
                  n195 = Index Array(array=w686, index=0 ("Index")) -> (element=w706:dbl)
                  n196 = Divide(x=w706, y=60.0) -> (x/y=w695:dbl)
                  n197 = Unbundle(w682) -> (w679:string[], w675:bool[])
                  n198 = Replace Array Subset(array=w686, new element=w695, index=0 ("Index")) -> (w674:dbl[])
                  n199 = Index Array(array=w675, index=3 ("Index")) -> (element=w683:bool)
                  n200 = case shown="True" w683 {
                    tunnel: [w757 w759] -> w680
                    frame False {
                      w756 = FALSE
                      w755 = TRUE
                      n201 = Build Array(w755, w755, w756, w756) -> (w757:bool[])
                    }
                    frame True {
                      w758 = TRUE
                      n202 = Build Array(w758, w758, w758, w758) -> (w759:bool[])
                    }
                  }
                  n203 = for {
                    tunnel: w675 -> [w748] mode=indexing
                    tunnel: w674 -> [w747]
                    shift-right: [w746] -> _
                    shift-left: 0 -> [w745]
                    shift-right: [w743] -> w671
                    shift-left: dbl[] [] -> [w742]
                    i -> [w740]
                    n204 = Index Array(array=w747, index=w745) -> (element=w744:dbl)
                    n205 = case shown="True" w748 {
                      tunnel: w745 -> [w750 w754]
                      tunnel: [w750 w752] -> w746
                      tunnel: w744 -> [_ w751]
                      tunnel: [0.0 w751] -> w741
                      frame False {
                      }
                      frame True {
                        n206 = Add(x=w754, y=1) -> (x+y=w752:i32)
                      }
                    }
                    n207 = Insert Into Array(array=w742, index=w740, new element=w741) -> (w743:dbl[])
                  }
                  n208 = Subtract(x=w690, y=1) -> (x-y=w700:i32)
                  n209 = Index Array(array=w692, index (row)=w700) -> (element=w705:dbl[])  [unwired: 1 in]
                  n210 = Replace Array Subset(array=w675, new element=w680, index=6 ("Index")) -> (w677:bool[])
                  n211 = Array Size(array=w705) -> (size(s)=w704:i32)
                  n212 = Bundle(w679, w677) -> (w678:cluster{string[], bool[]})  [unwired: 1 in]
                  n213 = Equal To 0?(x=w704) -> (x = 0?=w703:bool)
                  n214 = Insert Into Array(array=w671, index=6 ("Index"), new element=w693) -> (w685:dbl[])
                  n215 = case shown="True" w703 {
                    tunnel: w692 -> [w765 w769]
                    tunnel: [w762 w768] -> w702
                    tunnel: w685 -> [w764 w766]
                    tunnel: w700 -> [w763 w767]
                    frame False {
                      n216 = Replace Array Subset(array=w765, new element=w764, index (row)=w763) -> (w762:dbl[][])  [unwired: 1 in]
                    }
                    frame True {
                      n217 = Insert Into Array(array=w769, index (row)=w767, new element=w766) -> (w768:dbl[][])  [unwired: 1 in]
                    }
                  }
                }
              }
              n218 = case shown="True" w310 {
                tunnel: w293 -> [_ w348]
                tunnel: w302 -> [_ w351]
                tunnel: w315 -> [_ w354]
                tunnel: w314 -> [_ w350]
                tunnel: w299 -> [_ w349]
                frame False {
                }
                frame True {
                  n219 = local read "Trace length"() -> (w394:dbl)
                  n220 = Unbundle(w348) -> (w347:bool[])  [unwired: 1 out]
                  n221 = Add(x=w349, y=1) -> (x+y=w391:i32)
                  n222 = Multiply(x=w394, y=w349) -> (x*y=w392:dbl)
                  n223 = Multiply(x=w394, y=w391) -> (x*y=w393:dbl)
                  n224 = Multiply(x="Zoom from end", y=-1.0) -> (x*y=w372:dbl)
                  n225 = Concatenate Strings("Time, Event mark", "\r\n") -> (w389:string)
                  n226 = Index Array(array=w350, index (row)=w392, index (col)=0 ("Deaktivierter Index (Spalte)")) -> (element=w387:dbl)
                  n227 = Index Array(array=w350, index (row)=w393, index (col)=0 ("Deaktivierter Index (Spalte)")) -> (element=w388:dbl)
                  n228 = Add(x="Zoom from start", y=w372) -> (x+y=w365:dbl)
                  n229 = feedback #1() -> (w368:dbl)  [unwired: 1 in]
                  n230 = Greater Or Equal?(x=w365, y=0.0) -> (x >= y?=w366:bool)
                  n231 = case shown="True" w366 {
                    tunnel: "Zoom from start" -> [w397 w400]
                    tunnel: [w396 w400] -> w352
                    tunnel: w368 -> [w396 w402]
                    tunnel: "Zoom from end" -> [_ w399]
                    tunnel: [w397 w400] -> w373
                    tunnel: [w395 w398] -> w374
                    tunnel: "Zoom from end" -> [w395 w398]
                    frame False {
                    }
                    frame True {
                      n232 = Not Equal?(x=w402, y=w400) -> (x != y?=w401:bool)
                      n233 = case shown="False" w401 {
                        tunnel: w400 -> [_ w404]
                        tunnel: w399 -> [w403 _]
                        frame False {
                          n234 = local write "Zoom from start"(w403) -> ()
                        }
                        frame True {
                          n235 = local write "Zoom from end"(w404) -> ()
                        }
                      }
                    }
                  }
                  n236 = feedback-in #1(w352) -> ()
                  n237 = for {
                    tunnel: w354 -> [w658] mode=indexing
                    shift-right: [w660] -> w353
                    shift-left: dbl[] [] -> [w659]
                    tunnel: w387 -> [w657]
                    tunnel: w388 -> [w656]
                    shift-right: [w650] -> w390
                    shift-left: w389 -> [w653]
                    n238 = Unbundle(w658) -> (w645:dbl, w652:string)
                    n239 = Greater?(x=w645, y=w657) -> (0:w654:bool)
                    n240 = Less Or Equal?(x=w645, y=w656) -> (x <= y?=w655:bool)
                    n241 = And(x=w654, y=w655) -> (x .and. y?=w651:bool)
                    n242 = Divide(x=w645, y=60.0) -> (x/y=w646:dbl)
                    n243 = Number To Fractional String(number=w646, precision (6)=i16 2 ("Genauigkeit (6)")) -> (F-format string=w648:string)  [unwired: 2 in]
                    n244 = case shown="True" w651 {
                      tunnel: w653 -> [w661 w664]
                      tunnel: w652 -> [_ w667]
                      tunnel: [w661 w665] -> w650
                      tunnel: w648 -> [_ w662]
                      frame False {
                      }
                      frame True {
                        n245 = call <vilib>:"Space Constant.vi"() -> ("String"=w663:string)
                        n246 = Concatenate Strings(w664, w662, w663, w667, "\r\n") -> (w665:string)
                      }
                    }
                    n247 = Insert Into Array(array=w659, new element=w646) -> (w660:dbl[])  [unwired: 1 in]
                  }
                  "Event marks" <- w390
                  n248 = Subtract(x=w374, y=w373) -> (x-y=w369:dbl)
                  n249 = Index Array(array=w351, index (col)=0 ("Deaktivierter Index (Spalte)")) -> (element=w364:dbl[])  [unwired: 1 in]
                  n250 = Divide(x=w373, y=100.0) -> (x/y=w371:dbl)
                  n251 = Divide(x=w369, y=100.0) -> (x/y=w370:dbl)
                  n252 = Array Size(array=w364) -> (size(s)=w376:i32)
                  n253 = Multiply(x=w376, y=w371) -> (x*y=w379:dbl)
                  n254 = Multiply(x=w376, y=w370) -> (x*y=w377:dbl)
                  n255 = Add(x=w377, y=2.0) -> (x+y=w378:dbl)
                  n256 = Subtract(x=w379, y=2.0) -> (x-y=w380:dbl)
                  n257 = Array Subset(array=w351, index (row)=w380, length (row)=w378) -> (w355:dbl[][])  [unwired: 2 in]
                  n258 = Add(x=2, y="TC 3") -> (x+y=w346:u32)
                  n259 = Index Array(array=w347, index=w346) -> (element=w356:bool)
                  n260 = case shown="\"SISE channel #2\"" "TC 3" {
                    tunnel: w355 -> [w407 w490 w604 w611]
                    tunnel: w353 -> [w406 w489 w572 w614]
                    tunnel: w356 -> [w405 w488 w571 w608]
                    frame "SISE channel #1", Default {
                      n261 = Index Array(array=w407, index (col)=0 ("disabled index (col)")) -> (element=w414:dbl[])  [unwired: 1 in]
                      n262 = Index Array(array=w407, index (col)=2 ("disabled index (col)")) -> (element=w413:dbl[])  [unwired: 1 in]
                      n263 = Index Array(array=w407, index (col)=7 ("disabled index (col)")) -> (element=w410:dbl[])  [unwired: 1 in]
                      n264 = Index Array(array=w407, index (col)=6 ("disabled index (col)")) -> (element=w409:dbl[])  [unwired: 1 in]
                      n265 = for {
                        tunnel: w410 -> [w419] mode=indexing
                        tunnel: w409 -> [w418] mode=indexing
                        tunnel: [w417] -> w408 mode=indexing
                        n266 = Subtract(x=w419, y=w418) -> (x-y=w417:dbl)
                      }
                      n267 = stacked-sequence {
                        tunnel: w414 -> [w421 w460]
                        tunnel: w413 -> [w440 _]
                        tunnel: w406 -> [w422 w454]
                        tunnel: w408 -> [_ w459]
                        tunnel: w405 -> [w420 w455]
                        frame #0 {
                          n268 = Array Max & Min(array=w421) -> (max value=w432:dbl, min value=w431:dbl)  [unwired: 2 out]
                          n269 = Divide(x="Range limit\nS1.1 (mV)", y=2.0) -> (x/y=w450:dbl)
                          n270 = Divide(x="Range limit\nS1.1 (mV)", y=2.05) -> (x/y=w451:dbl)
                          n271 = Add(x="Base line\nS1.1 (mV)", y=w450) -> (x+y=w423:dbl)
                          n272 = Subtract(x="Base line\nS1.1 (mV)", y=w450) -> (x-y=w424:dbl)
                          n273 = Subtract(x="Base line\nS1.1 (mV)", y=w451) -> (x-y=w430:dbl)
                          n274 = call "EventstoGraph (SubVI).vi"("Numerisch 2"=w431, "Array 3"=w422, "Numerisch"=w432, "Array (Eingang)"=dbl[][] [], "Numerisch 3"=w430) -> ("Array (Ausgang)"=w434:dbl[][])  [unwired: 6 in]
                          n275 = Array Max & Min(array=w421) -> (max value=w446:dbl, min value=w447:dbl)  [unwired: 2 out]
                          n276 = call "GraphLimit01.vi"("Numeric 2"=w424, "Numeric"=w423, "Array in"=w440, "Array 3"=dbl[] []) -> ("Array out"=w439:dbl[])  [unwired: 7 in]
                          n277 = Build Array("Base line\nS1.1 (mV)", "Base line\nS1.1 (mV)") -> (w443:dbl[])
                          n278 = Build Array(w446, w447) -> (w444:dbl[])
                          n279 = Build Array(w423, w424) -> (w445:dbl[])
                          n280 = Index Array(array=w434, index (col)=0 ("Index (Zeile)")) -> (element=w435:dbl[])  [unwired: 1 in]
                          n281 = Index Array(array=w434, index (col)=1 ("Index (Zeile)")) -> (element=w433:dbl[])  [unwired: 1 in]
                          n282 = Bundle(w444, w445) -> (w427:cluster{dbl[], dbl[]})  [unwired: 1 in]
                          n283 = Bundle(w444, w443) -> (w428:cluster{dbl[], dbl[]})  [unwired: 1 in]
                          n284 = Bundle(w421, "Array out"=w439) -> (w426:cluster{dbl[], "Array out":dbl[]})  [unwired: 1 in]
                          n285 = Bundle("Array (Ausgang)"=w435, "Array (Ausgang)"=w433) -> (w425:T17)  [unwired: 1 in]
                          n286 = Build Array(w428, w427, w426, w425) -> (w429:T18)
                          n287 = case shown="True" w420 {
                            tunnel: w429 -> [_ w453]
                            frame False {
                            }
                            frame True {
                              "V-SISE channel 1" <- w453
                            }
                          }
                        }
                        frame #1 {
                          n288 = Array Max & Min(array=w460) -> (max value=w469:dbl, min value=w468:dbl)  [unwired: 2 out]
                          n289 = Divide(x="Range limit\nS1.2 mV", y=2.0) -> (x/y=w485:dbl)
                          n290 = Divide(x="Range limit\nS1.2 mV", y=2.05) -> (x/y=w486:dbl)
                          n291 = Add(x="Base line \nS1.2 (mV)", y=w485) -> (x+y=w461:dbl)
                          n292 = Subtract(x="Base line \nS1.2 (mV)", y=w485) -> (x-y=w462:dbl)
                          n293 = Subtract(x="Base line \nS1.2 (mV)", y=w486) -> (x-y=w467:dbl)
                          n294 = call "EventstoGraph (SubVI).vi"("Numerisch 2"=w468, "Array 3"=w454, "Numerisch"=w469, "Array (Eingang)"=dbl[][] [], "Numerisch 3"=w467) -> ("Array (Ausgang)"=w471:dbl[][])  [unwired: 6 in]
                          n295 = Array Max & Min(array=w460) -> (max value=w481:dbl, min value=w482:dbl)  [unwired: 2 out]
                          n296 = call "GraphLimit01.vi"("Numeric 2"=w462, "Numeric"=w461, "Array in"=w459, "Array 3"=dbl[] []) -> ("Array out"=w476:dbl[])  [unwired: 7 in]
                          n297 = Build Array("Base line \nS1.2 (mV)", "Base line \nS1.2 (mV)") -> (w478:dbl[])
                          n298 = Build Array(w481, w482) -> (w479:dbl[])
                          n299 = Build Array(w461, w462) -> (w480:dbl[])
                          n300 = Index Array(array=w471, index (col)=0 ("Index (Zeile)")) -> (element=w472:dbl[])  [unwired: 1 in]
                          n301 = Index Array(array=w471, index (col)=1 ("Index (Zeile)")) -> (element=w470:dbl[])  [unwired: 1 in]
                          n302 = Bundle(w479, w480) -> (w465:cluster{dbl[], dbl[]})  [unwired: 1 in]
                          n303 = Bundle(w479, w478) -> (w466:cluster{dbl[], dbl[]})  [unwired: 1 in]
                          n304 = Bundle(w460, "Array out"=w476) -> (w464:cluster{dbl[], "Array out":dbl[]})  [unwired: 1 in]
                          n305 = Bundle("Array (Ausgang)"=w472, "Array (Ausgang)"=w470) -> (w463:T17)  [unwired: 1 in]
                          n306 = Build Array(w466, w465, w464, w463) -> (w456:T18)
                          n307 = case shown="True" w455 {
                            tunnel: w456 -> [_ w487]
                            frame False {
                            }
                            frame True {
                              "dV-SISE channel 1" <- w487
                            }
                          }
                        }
                      }
                    }
                    frame "SISE channel #2" {
                      n308 = Index Array(array=w490, index (col)=0 ("disabled index (col)")) -> (element=w497:dbl[])  [unwired: 1 in]
                      n309 = Index Array(array=w490, index (col)=3 ("disabled index (col)")) -> (element=w496:dbl[])  [unwired: 1 in]
                      n310 = Index Array(array=w490, index (col)=9 ("disabled index (col)")) -> (element=w493:dbl[])  [unwired: 1 in]
                      n311 = Index Array(array=w490, index (col)=8 ("disabled index (col)")) -> (element=w492:dbl[])  [unwired: 1 in]
                      n312 = for {
                        tunnel: w493 -> [w502] mode=indexing
                        tunnel: w492 -> [w501] mode=indexing
                        tunnel: [w500] -> w491 mode=indexing
                        n313 = Subtract(x=w502, y=w501) -> (x-y=w500:dbl)
                      }
                      n314 = stacked-sequence {
                        tunnel: w497 -> [w506 w543]
                        tunnel: w496 -> [w525 _]
                        tunnel: w489 -> [w507 w539]
                        tunnel: w491 -> [_ w542]
                        tunnel: w488 -> [w505 w540]
                        frame #0 {
                          n315 = Array Max & Min(array=w506) -> (max value=w517:dbl, min value=w516:dbl)  [unwired: 2 out]
                          n316 = Divide(x="Range limit\nS1.1 (mV) 2", y=2.0) -> (x/y=w534:dbl)
                          n317 = Divide(x="Range limit\nS1.1 (mV) 2", y=2.05) -> (x/y=w535:dbl)
                          n318 = Add(x="Base line\nS1.1 (mV)", y=w534) -> (x+y=w508:dbl)
                          n319 = Subtract(x="Base line\nS1.1 (mV)", y=w534) -> (x-y=w509:dbl)
                          n320 = Subtract(x="Base line\nS1.1 (mV)", y=w535) -> (x-y=w515:dbl)
                          n321 = call "EventstoGraph (SubVI).vi"("Numerisch 2"=w516, "Array 3"=w507, "Numerisch"=w517, "Array (Eingang)"=dbl[][] [], "Numerisch 3"=w515) -> ("Array (Ausgang)"=w519:dbl[][])  [unwired: 6 in]
                          n322 = Array Max & Min(array=w506) -> (max value=w530:dbl, min value=w531:dbl)  [unwired: 2 out]
                          n323 = call "GraphLimit01.vi"("Numeric 2"=w509, "Numeric"=w508, "Array in"=w525, "Array 3"=dbl[] []) -> ("Array out"=w524:dbl[])  [unwired: 7 in]
                          n324 = Build Array("Base line\nS1.1 (mV)", "Base line\nS1.1 (mV)") -> (w527:dbl[])
                          n325 = Build Array(w530, w531) -> (w528:dbl[])
                          n326 = Build Array(w508, w509) -> (w529:dbl[])
                          n327 = Index Array(array=w519, index (col)=0 ("Index (Zeile)")) -> (element=w520:dbl[])  [unwired: 1 in]
                          n328 = Index Array(array=w519, index (col)=1 ("Index (Zeile)")) -> (element=w518:dbl[])  [unwired: 1 in]
                          n329 = Bundle(w528, w529) -> (w512:cluster{dbl[], dbl[]})  [unwired: 1 in]
                          n330 = Bundle(w528, w527) -> (w513:cluster{dbl[], dbl[]})  [unwired: 1 in]
                          n331 = Bundle(w506, "Array out"=w524) -> (w511:cluster{dbl[], "Array out":dbl[]})  [unwired: 1 in]
                          n332 = Bundle("Array (Ausgang)"=w520, "Array (Ausgang)"=w518) -> (w510:T17)  [unwired: 1 in]
                          n333 = Build Array(w513, w512, w511, w510) -> (w514:T18)
                          n334 = case shown="True" w505 {
                            tunnel: w514 -> [_ w536]
                            frame False {
                            }
                            frame True {
                              "V-SISE channel 2" <- w536
                            }
                          }
                        }
                        frame #1 {
                          n335 = Array Max & Min(array=w543) -> (max value=w552:dbl, min value=w551:dbl)  [unwired: 2 out]
                          n336 = Divide(x="Range limit\nS2.2 (mV)", y=2.0) -> (x/y=w568:dbl)
                          n337 = Divide(x="Range limit\nS2.2 (mV)", y=2.05) -> (x/y=w569:dbl)
                          n338 = Add(x="Base line \nS2.2 (mV)", y=w568) -> (x+y=w544:dbl)
                          n339 = Subtract(x="Base line \nS2.2 (mV)", y=w568) -> (x-y=w545:dbl)
                          n340 = Subtract(x="Base line \nS2.2 (mV)", y=w569) -> (x-y=w550:dbl)
                          n341 = call "EventstoGraph (SubVI).vi"("Numerisch 2"=w551, "Array 3"=w539, "Numerisch"=w552, "Array (Eingang)"=dbl[][] [], "Numerisch 3"=w550) -> ("Array (Ausgang)"=w554:dbl[][])  [unwired: 6 in]
                          n342 = Array Max & Min(array=w543) -> (max value=w564:dbl, min value=w565:dbl)  [unwired: 2 out]
                          n343 = call "GraphLimit01.vi"("Numeric 2"=w545, "Numeric"=w544, "Array in"=w542, "Array 3"=dbl[] []) -> ("Array out"=w559:dbl[])  [unwired: 7 in]
                          n344 = Build Array("Base line \nS2.2 (mV)", "Base line \nS2.2 (mV)") -> (w561:dbl[])
                          n345 = Build Array(w564, w565) -> (w562:dbl[])
                          n346 = Build Array(w544, w545) -> (w563:dbl[])
                          n347 = Index Array(array=w554, index (col)=0 ("Index (Zeile)")) -> (element=w555:dbl[])  [unwired: 1 in]
                          n348 = Index Array(array=w554, index (col)=1 ("Index (Zeile)")) -> (element=w553:dbl[])  [unwired: 1 in]
                          n349 = Bundle(w562, w563) -> (w548:cluster{dbl[], dbl[]})  [unwired: 1 in]
                          n350 = Bundle(w562, w561) -> (w549:cluster{dbl[], dbl[]})  [unwired: 1 in]
                          n351 = Bundle(w543, "Array out"=w559) -> (w547:cluster{dbl[], "Array out":dbl[]})  [unwired: 1 in]
                          n352 = Bundle("Array (Ausgang)"=w555, "Array (Ausgang)"=w553) -> (w546:T17)  [unwired: 1 in]
                          n353 = Build Array(w549, w548, w547, w546) -> (w541:T18)
                          n354 = case shown="True" w540 {
                            tunnel: w541 -> [_ w570]
                            frame False {
                            }
                            frame True {
                              "dV-SISE channel 2" <- w570
                            }
                          }
                        }
                      }
                    }
                    frame "V channel #1" {
                      n355 = Index Array(array=w604, index (col)=0 ("disabled index (col)")) -> (element=w573:dbl[])  [unwired: 1 in]
                      n356 = Index Array(array=w604, index (col)=4 ("disabled index (col)")) -> (element=w574:dbl[])  [unwired: 1 in]
                      n357 = Array Max & Min(array=w573) -> (max value=w584:dbl, min value=w583:dbl)  [unwired: 2 out]
                      n358 = Divide(x="Range limit\nV1 (V)", y=2.0) -> (x/y=w601:dbl)
                      n359 = Divide(x="Range limit\nV1 (V)", y=2.05) -> (x/y=w602:dbl)
                      n360 = Add(x="Base line\nV1 (V)", y=w601) -> (x+y=w575:dbl)
                      n361 = Subtract(x="Base line\nV1 (V)", y=w601) -> (x-y=w576:dbl)
                      n362 = Subtract(x="Base line\nV1 (V)", y=w602) -> (x-y=w582:dbl)
                      n363 = call "EventstoGraph (SubVI).vi"("Numerisch 2"=w583, "Array 3"=w572, "Numerisch"=w584, "Array (Eingang)"=dbl[][] [], "Numerisch 3"=w582) -> ("Array (Ausgang)"=w586:dbl[][])  [unwired: 6 in]
                      n364 = Array Max & Min(array=w573) -> (max value=w597:dbl, min value=w598:dbl)  [unwired: 2 out]
                      n365 = call "GraphLimit01.vi"("Numeric 2"=w576, "Numeric"=w575, "Array in"=w574, "Array 3"=dbl[] []) -> ("Array out"=w591:dbl[])  [unwired: 7 in]
                      n366 = Build Array("Base line\nV1 (V)", "Base line\nV1 (V)") -> (w594:dbl[])
                      n367 = Build Array(w597, w598) -> (w595:dbl[])
                      n368 = Build Array(w575, w576) -> (w596:dbl[])
                      n369 = Index Array(array=w586, index (col)=0 ("Index (Zeile)")) -> (element=w587:dbl[])  [unwired: 1 in]
                      n370 = Index Array(array=w586, index (col)=1 ("Index (Zeile)")) -> (element=w585:dbl[])  [unwired: 1 in]
                      n371 = Bundle(w595, w596) -> (w579:cluster{dbl[], dbl[]})  [unwired: 1 in]
                      n372 = Bundle(w595, w594) -> (w580:cluster{dbl[], dbl[]})  [unwired: 1 in]
                      n373 = Bundle(w573, "Array out"=w591) -> (w578:cluster{dbl[], "Array out":dbl[]})  [unwired: 1 in]
                      n374 = Bundle("Array (Ausgang)"=w587, "Array (Ausgang)"=w585) -> (w577:T17)  [unwired: 1 in]
                      n375 = Build Array(w580, w579, w578, w577) -> (w581:T18)
                      n376 = case shown="True" w571 {
                        tunnel: w581 -> [_ w607]
                        frame False {
                        }
                        frame True {
                          "Voltage channel 1" <- w607
                        }
                      }
                    }
                    frame "V channel #2" {
                      n377 = Index Array(array=w611, index (col)=0 ("disabled index (col)")) -> (element=w609:dbl[])  [unwired: 1 in]
                      n378 = Index Array(array=w611, index (col)=5 ("disabled index (col)")) -> (element=w610:dbl[])  [unwired: 1 in]
                      n379 = Array Max & Min(array=w609) -> (max value=w624:dbl, min value=w623:dbl)  [unwired: 2 out]
                      n380 = Divide(x="Range limit\nV2 (V)", y=2.0) -> (x/y=w641:dbl)
                      n381 = Divide(x="Range limit\nV2 (V)", y=2.05) -> (x/y=w642:dbl)
                      n382 = Add(x="Base line\nV2 (V)", y=w641) -> (x+y=w615:dbl)
                      n383 = Subtract(x="Base line\nV2 (V)", y=w641) -> (x-y=w616:dbl)
                      n384 = Subtract(x="Base line\nV2 (V)", y=w642) -> (x-y=w622:dbl)
                      n385 = call "EventstoGraph (SubVI).vi"("Numerisch 2"=w623, "Array 3"=w614, "Numerisch"=w624, "Array (Eingang)"=dbl[][] [], "Numerisch 3"=w622) -> ("Array (Ausgang)"=w626:dbl[][])  [unwired: 6 in]
                      n386 = Array Max & Min(array=w609) -> (max value=w637:dbl, min value=w638:dbl)  [unwired: 2 out]
                      n387 = call "GraphLimit01.vi"("Numeric 2"=w616, "Numeric"=w615, "Array in"=w610, "Array 3"=dbl[] []) -> ("Array out"=w631:dbl[])  [unwired: 7 in]
                      n388 = Build Array("Base line\nV2 (V)", "Base line\nV2 (V)") -> (w634:dbl[])
                      n389 = Build Array(w637, w638) -> (w635:dbl[])
                      n390 = Build Array(w615, w616) -> (w636:dbl[])
                      n391 = Index Array(array=w626, index (col)=0 ("Index (Zeile)")) -> (element=w627:dbl[])  [unwired: 1 in]
                      n392 = Index Array(array=w626, index (col)=1 ("Index (Zeile)")) -> (element=w625:dbl[])  [unwired: 1 in]
                      n393 = Bundle(w635, w636) -> (w619:cluster{dbl[], dbl[]})  [unwired: 1 in]
                      n394 = Bundle(w635, w634) -> (w620:cluster{dbl[], dbl[]})  [unwired: 1 in]
                      n395 = Bundle(w609, "Array out"=w631) -> (w618:cluster{dbl[], "Array out":dbl[]})  [unwired: 1 in]
                      n396 = Bundle("Array (Ausgang)"=w627, "Array (Ausgang)"=w625) -> (w617:T17)  [unwired: 1 in]
                      n397 = Build Array(w620, w619, w618, w617) -> (w621:T18)
                      n398 = case shown="True" w608 {
                        tunnel: w621 -> [_ w644]
                        frame False {
                        }
                        frame True {
                          "Voltage channel 2" <- w644
                        }
                      }
                    }
                  }
                }
              }
              n399 = Subtract(x=w319, y=2.0) -> (x-y=w316:dbl)
              n400 = Equal?(x=w316, y=w317) -> (x = y?=→"Scroll data":bool)
              n401 = Or(x="Step forward", y="Step back") -> (x .or. y?=w339:bool)
              n402 = Or(x="Step back", y="Scroll back") -> (x .or. y?=w337:bool)
              n403 = Or(x="Scroll back", y="Scroll forward") -> (x .or. y?=w333:bool)
              n404 = case shown="\"SISE chan #1\", Default" "?" {
                selector: "?" -> [w866 w878 w886 w894]
                tunnel: w321 -> [w873 w880 w890 w897]
                tunnel: w325 -> [w874 w881 w889 w898]
                tunnel: w323 -> [w870 w877 w884 w893]
                tunnel: "Start fit (% of rec. period)" -> [w872 w879 w888 w896]
                frame "SISE chan #1", Default {
                  n405 = Add(x=2, y=w866) -> (x+y=w867:u32)
                  n406 = Index Array(array=w870, index=w867) -> (element=w869:bool)
                  n407 = call "Feed-SISE-Probe-Graph.vi"("Boolesch"=w869, "Numerisch"=2, "Array 2"=w874, "Array"=w873, "Start fit (% of rec. period)"=w872) -> ("Array 3"=→"Vprobe SISE 1":cluster{dbl[], dbl[]}[])  [unwired: 6 in]
                }
                frame "SISE chan #2" {
                  n408 = Index Array(array=w877, index=w878) -> (element=w876:bool)
                  n409 = call "Feed-SISE-Probe-Graph.vi"("Boolesch"=w876, "Numerisch"=3, "Array 2"=w881, "Array"=w880, "Start fit (% of rec. period)"=w879) -> ("Array 3"=→"Vprobe SISE 2":cluster{dbl[], dbl[]}[])  [unwired: 6 in]
                }
                frame "V chan #1" {
                  n410 = Index Array(array=w884, index=w886) -> (element=w885:bool)
                  n411 = call "Feed-V-Probe-Graph.vi"("Boolesch"=w885, "Numerisch"=4, "Array 2"=w889, "Array"=w890, "Start fit (% of rec. period)"=w888) -> ("Array 3"=→"Vprobe V 1":cluster{dbl[], dbl[]}[])  [unwired: 6 in]
                }
                frame "V chan #2" {
                  n412 = Index Array(array=w893, index=w894) -> (element=w892:bool)
                  n413 = call "Feed-V-Probe-Graph.vi"("Boolesch"=w892, "Numerisch"=5, "Array 2"=w898, "Array"=w897, "Start fit (% of rec. period)"=w896) -> ("Array 3"=→"Vprobe V 2":cluster{dbl[], dbl[]}[])  [unwired: 6 in]
                }
              }
              n414 = call "Feed-Position-Graph (SubVI).vi"("Array 2"=w321, "Array"=w325) -> ("Array 3"=→"Position probe":cluster{dbl[], dbl[]}[])  [unwired: 9 in]
              n415 = Or(x=w339, y=w333) -> (x .or. y?=w338:bool)
              n416 = case shown="True" w338 {
                tunnel: [0 w923] -> w336
                tunnel: w337 -> [_ w922]
                frame False {
                }
                frame True {
                  n417 = case shown="True" w922 {
                    tunnel: [1 2] -> w923
                    frame False {
                    }
                    frame True {
                    }
                  }
                }
              }
              n418 = case shown="True" w333 {
                tunnel: [200 w900] -> w332
                frame False {
                }
                frame True {
                  n419 = Divide(x=500.0, y="Scroll speed") -> (x/y=w900:dbl)
                }
              }
              n420 = case shown="2" w336 {
                tunnel: w299 -> [w903 w909 w916]
                tunnel: w319 -> [_ w904 _]
                tunnel: [w903 w908 w915] -> w296
                frame 0, Default {
                }
                frame 1 {
                  n421 = Subtract(x=w904, y=1) -> (x-y=w906:dbl)
                  n422 = Less?(x=w909, y=w906) -> (x < y?=w907:bool)
                  n423 = case shown="False" w907 {
                    tunnel: w909 -> [w910 w913]
                    tunnel: [w910 w911] -> w908
                    frame False {
                    }
                    frame True {
                      n424 = Add(x=w913, y=1) -> (x+y=w911:i32)
                    }
                  }
                }
                frame 2 {
                  n425 = Greater Than 0?(x=w916) -> (x > 0?=w914:bool)
                  n426 = case shown="True" w914 {
                    tunnel: w916 -> [w917 w920]
                    tunnel: [w917 w918] -> w915
                    frame False {
                    }
                    frame True {
                      n427 = Subtract(x=w920, y=1) -> (x-y=w918:i32)
                    }
                  }
                }
              }
              "Trace #" <- w296
              n428 = Wait (ms)(milliseconds to wait=w332) -> ()  [unwired: 1 out]
              n429 = Replace Array Subset(array=w297, new element=w296, index=0 ("Index")) -> (w298:i32[])
            }
          }
          n430 = Equal?(x="Module selection view data", y=u16 0) -> (x = y?=w98:bool)
          n431 = Select(t=T9."Enabled" ("Disabled"), s=w98, f=T9."Disabled and Grayed Out") -> (s? t:f=w95:T9)
          n432 = property on="Load data" class="Bool (strict)"("DisabledEnum"=w95) -> ()  [unwired: 2 in, 2 out]
          n433 = Equal?(x="Module selection view data", y=u16 1) -> (x = y?=w93:bool)
          n434 = Select(t=T9."Enabled" ("Disabled"), s=w93, f=T9."Disabled and Grayed Out") -> (s? t:f=w90:T9)
          n435 = property on="Scroll data" class="Bool (strict)"("DisabledEnum"=w90) -> ()  [unwired: 2 in, 2 out]
          n436 = Replace Array Subset(array=w79, new element=w76, index=0 ("Index")) -> (w77:T13)
        }
        frame "Save analysis" {
          n437 = Index Array(array=w937, index=1 ("Index")) -> (element=w938:T12)
          n438 = case shown="\"Save data\"" "Module selection Save Data" {
            tunnel: w938 -> [w984 w1016 w1028]
            tunnel: [w979 w1016 w1028] -> w936
            tunnel: w962 -> [w974 w1019 w1036]
            tunnel: w961 -> [w975 w1020 w1035]
            tunnel: w960 -> [w976 w1021 w1034]
            tunnel: w959 -> [w977 w1018 w1033]
            tunnel: w958 -> [w978 w1017 w1032]
            tunnel: [w973 w1014 w1031] -> w933
            tunnel: [0 2 1] -> w941
            tunnel: w927 -> [w963 w1013 w1027]
            frame "Create analysis file", Default {
              n439 = local read "Raw data file in"() -> (→"Raw data file":path)
              n440 = call <vilib>:"Check if File or Folder Exists.vi"("path"="Analysis output file") -> ("file or folder exists?"=w964:bool, "dup path"=w968:path)  [unwired: 8 in, 1 out]
              n441 = Unbundle(w984) -> (w982:path, "Referenz (Ausgang)"=w970:refnum<file>, w980:bool, w981:i32, w972:string)
              n442 = Bundle(w963, w974, w975, w976, w977, w978) -> (w973:T15)  [unwired: 1 in]
              n443 = Not(x=w964) -> (.not. x?=w965:bool)
              n444 = Bundle(w980, w981, w972) -> (w971:errorcluster)  [unwired: 1 in]
              n445 = Not Equal?(x=w968, y=w982) -> (x != y?=w967:bool)
              n446 = And(x=w965, y=w967) -> (x .and. y?=w966:bool)
              n447 = feedback #2(FALSE) -> (w988:bool)
              n448 = case shown="True" w966 {
                tunnel: w968 -> [_ w999]
                tunnel: [w997 w1002] -> w987
                tunnel: w988 -> [w997 _]
                tunnel: [w990 w1004] -> w979
                tunnel: [w997 w1002] -> w989
                tunnel: w982 -> [w995 _]
                tunnel: w971 -> [w996 w1000]
                tunnel: w970 -> [w991 _]
                frame False {
                  n449 = Unbundle(w996) -> (w992:bool, w993:i32, w994:string)
                  n450 = Bundle(w995, "Referenz (Ausgang)"=w991, w992, w993, w994) -> (w990:T12)  [unwired: 1 in]
                }
                frame True {
                  n451 = Open/Create/Replace File(file path (use dialog)=w999, error in=w1000, operation (0:open)=T10."create") -> (refnum out=w1010:refnum<file>, error out=w1009:errorcluster)  [unwired: 3 in, 1 out]
                  n452 = Set File Position(offset (in bytes) (0)=i64 0, refnum=w1010, from (0:start)=enum16{"start", "end", "current"}."end", error in=w1009) -> (refnum out=w998:refnum<file>, error out=w1003:errorcluster)
                  n453 = Unbundle By Name(w1003) -> ("status"=w1001:bool)
                  n454 = Not(x=w1001) -> (.not. x?=w1002:bool)
                  n455 = Unbundle(w1003) -> ("status"=w1007:bool, "code"=w1006:i32, "source"=w1005:string)
                  n456 = Bundle("dup path"=w999, "refnum"=w998, "status"=w1007, "code"=w1006, "source"=w1005) -> (w1004:T19)  [unwired: 1 in]
                }
              }
              "Create analysis file" <- w987
              n457 = feedback-in #2(w989) -> ()
            }
            frame "New/stop analysis" {
              n458 = Bundle(w1013, w1019, w1020, w1021, w1018, w1017) -> (w1014:T15)  [unwired: 1 in]
              n459 = local read "Save analyses file"() -> (w1015:bool)
              "Next data file/exit program" <- w1015
              n460 = case shown="True" w1015 {
                frame False {
                }
                frame True {
                  n461 = Or(x="Exit program", y="Next data file") -> (x .or. y?=w1025:bool)
                  n462 = case shown="True" w1025 {
                    frame False {
                    }
                    frame True {
                      n463 = local write "Main Tab Control"(0) -> ()
                    }
                  }
                }
              }
            }
            frame "Save data" {
              n464 = Unbundle(w1034) -> (w1040:string[], w1042:bool[])
              n465 = for {
                tunnel: "Select output" -> [w1056] mode=indexing
                tunnel: w1042 -> [w1057] mode=indexing
                shift-right: [w1053] -> w1039
                shift-left: bool[] [] -> [w1054]
                n466 = And(x=w1057, y=w1056) -> (x .and. y?=w1055:bool)
                n467 = case shown="True" w1055 {
                  tunnel: w1054 -> [w1059 w1062]
                  tunnel: [w1058 w1063] -> w1053
                  frame False {
                    n468 = Insert Into Array(array=w1059, new element=FALSE) -> (w1058:bool[])  [unwired: 1 in]
                  }
                  frame True {
                    n469 = Insert Into Array(array=w1062, new element=TRUE) -> (w1063:bool[])  [unwired: 1 in]
                  }
                }
              }
              "Indicate output" <- w1039
              n470 = Bundle(w1027, w1036, w1035, w1034, w1033, w1032) -> (w1031:T15)  [unwired: 1 in]
              n471 = local read "Create analysis file"() -> (w1029:bool)
              n472 = And(x=w1029, y="Save data") -> (x .and. y?=w1038:bool)
              n473 = case shown="True" w1038 {
                tunnel: w1040 -> [_ w1076]
                tunnel: w1039 -> [_ w1069]
                tunnel: w1033 -> [_ w1073]
                tunnel: w1028 -> [_ w1081]
                tunnel: w1027 -> [_ w1064]
                frame False {
                }
                frame True {
                  n474 = Index Array(array=w1073, index (col)=0 ("Index (Zeile)")) -> (element=w1082:dbl[])  [unwired: 1 in]
                  n475 = for {
                    tunnel: w1069 -> [w1086] mode=indexing
                    shift-right: [w1083] -> w1068
                    shift-left: 0 -> [w1084]
                    i -> [w1085]
                    n476 = case shown="True" w1086 {
                      tunnel: w1085 -> [_ w1088]
                      tunnel: w1084 -> [w1087 _]
                      tunnel: [w1087 w1088] -> w1083
                      frame False {
                      }
                      frame True {
                      }
                    }
                  }
                  n477 = Unbundle(w1081) -> ("Referenz (Ausgang)"=w1077:refnum<file>, w1078:bool, w1079:i32, w1080:string)  [unwired: 1 out]
                  n478 = Array Size(array=w1082) -> (size(s)=w1075:i32)
                  n479 = Bundle(w1078, w1079, w1080) -> (w1067:errorcluster)  [unwired: 1 in]
                  n480 = Add(x=w1075, y=2) -> (x+y=w1071:i32)
                  n481 = for {
                    N: w1071 -> [_]
                    tunnel: w1076 -> [w1099]
                    tunnel: w1077 -> [w1102]
                    tunnel: w1069 -> [w1100]
                    tunnel: w1073 -> [w1098]
                    tunnel: w1068 -> [w1094]
                    tunnel: w1067 -> [w1092]
                    tunnel: [w1091] -> w1066
                    tunnel: [w1090] -> w1065
                    tunnel: w1064 -> [w1089]
                    i -> [w1093]
                    n482 = Greater Or Equal?(x=w1093, y=2) -> (x >= y?=w1097:bool)
                    n483 = case shown="True" w1097 {
                      tunnel: [w1103 2] -> w1095
                      tunnel: w1093 -> [w1103 _]
                      frame False {
                      }
                      frame True {
                      }
                    }
                    n484 = case shown="0, Default" w1095 {
                      tunnel: [w1108 w1143 w1164] -> w1101
                      tunnel: w1100 -> [w1112 w1142 w1166]
                      tunnel: w1099 -> [_ w1145 _]
                      tunnel: w1098 -> [_ _ w1169]
                      tunnel: w1094 -> [_ w1141 w1162]
                      tunnel: w1093 -> [_ _ w1161]
                      tunnel: w1089 -> [w1109 _ _]
                      frame 0, Default {
                        n485 = Index Array(array=w1112, index=13) -> (element=w1110:bool)
                        n486 = case shown="False" w1110 {
                          tunnel: w1109 -> [w1117 w1131]
                          tunnel: [w1116 w1125] -> w1106
                          frame False {
                            n487 = Index Array(array=w1117, index=0) -> (element=w1120:bool)
                            n488 = case shown="True" w1120 {
                              tunnel: ["Diff. gradient" "Chem. potential"] -> w1119
                              frame False {
                              }
                              frame True {
                              }
                            }
                            n489 = Concatenate Strings("Anal. method channel 1: ", w1119, "\r\n") -> (w1116:string)
                          }
                          frame True {
                            n490 = Index Array(array=w1131, index=0) -> (element=w1134:bool)
                            n491 = Index Array(array=w1131, index=1) -> (element=w1132:bool)
                            n492 = case shown="True" w1134 {
                              tunnel: ["Diff. gradient" "Chem. potential"] -> w1130
                              frame False {
                              }
                              frame True {
                              }
                            }
                            n493 = case shown="True" w1132 {
                              tunnel: ["Diff. gradient" "Chem. potential"] -> w1127
                              frame False {
                              }
                              frame True {
                              }
                            }
                            n494 = Concatenate Strings("Anal. method channel 1: ", w1130, "\t", "Anal. method channel 2: ", w1127, "\r\n") -> (w1125:string)
                          }
                        }
                        n495 = local read "Raw data file in"() -> (w1113:path)
                        n496 = Path To String(path=w1113) -> (string=w1115:string)
                        n497 = Concatenate Strings("Datafile in: ", w1115, "\t") -> (w1107:string)
                        n498 = Concatenate Strings(w1107, w1106) -> (w1108:string)
                      }
                      frame 1 {
                        n499 = for {
                          tunnel: w1141 -> [w1150]
                          tunnel: w1142 -> [w1153] mode=indexing
                          tunnel: w1145 -> [w1152] mode=indexing
                          shift-right: [w1148] -> w1143
                          shift-left: "" -> [w1147]
                          i -> [w1151]
                          n500 = Equal?(x=w1150, y=w1151) -> (x = y?=w1149:bool)
                          n501 = case shown="False" w1153 {
                            tunnel: w1152 -> [_ w1158]
                            tunnel: w1149 -> [_ w1157]
                            tunnel: ["" w1155] -> w1146
                            frame False {
                            }
                            frame True {
                              n502 = case shown="True" w1157 {
                                tunnel: ["\t" "\r\n"] -> w1156
                                frame False {
                                }
                                frame True {
                                }
                              }
                              n503 = Concatenate Strings(w1158, w1156) -> (w1155:string)
                            }
                          }
                          n504 = Concatenate Strings(w1147, w1146) -> (w1148:string)
                        }
                      }
                      frame 2 {
                        n505 = Subtract(x=w1161, y=2 ("x")) -> (x-y=w1167:i32)
                        n506 = Index Array(array=w1169, index (row)=w1167) -> (element=w1165:dbl[])  [unwired: 1 in]
                        n507 = for {
                          tunnel: w1166 -> [w1177] mode=indexing
                          tunnel: w1165 -> [w1176] mode=indexing
                          shift-right: [w1172] -> w1164
                          shift-left: "" -> [w1171]
                          tunnel: w1162 -> [w1174]
                          i -> [w1173]
                          n508 = Equal?(x=w1174, y=w1173) -> (x = y?=w1175:bool)
                          n509 = case shown="False" w1177 {
                            tunnel: w1176 -> [_ w1183]
                            tunnel: ["" w1184] -> w1170
                            tunnel: w1175 -> [_ w1180]
                            frame False {
                            }
                            frame True {
                              n510 = Number To Exponential String(number=w1183, precision (6)=i16 6 ("Genauigkeit (6)")) -> (E-format string=w1181:string)  [unwired: 2 in]
                              n511 = case shown="False" w1180 {
                                tunnel: ["\t" "\r\n"] -> w1179
                                frame False {
                                }
                                frame True {
                                }
                              }
                              n512 = Concatenate Strings(w1181, w1179) -> (w1184:string)
                            }
                          }
                          n513 = Concatenate Strings(w1171, w1170) -> (w1172:string)
                        }
                      }
                    }
                    n514 = Write to Text File(file (use dialog)=w1102, text=w1101, error in=w1092) -> (refnum out=w1091:refnum<file>, error out=w1090:errorcluster)  [unwired: 1 in, 1 out]
                  }
                  n515 = Close File(refnum=w1066, error in=w1065) -> ()  [unwired: 2 out]
                }
              }
              n516 = case shown="True" w1029 {
                tunnel: w1028 -> [_ w1049]
                frame False {
                }
                frame True {
                  n517 = Unbundle(w1049) -> (w1044:path, w1046:bool, w1047:i32, w1048:string)  [unwired: 1 out]
                  n518 = Bundle(w1046, w1047, w1048) -> (w1045:errorcluster)  [unwired: 1 in]
                  n519 = Read from Text File(file (use dialog)=w1044, error in=w1045) -> (text=w1052:string)  [unwired: 2 in, 3 out]
                  n520 = String Length(string=w1052) -> (length=w1051:i32)
                  n521 = Not Equal To 0?(x=w1051) -> (x != 0?=→"Save analyses file":bool)
                }
              }
              "Cluster 3" <- w1034
            }
          }
          n522 = Equal?(x=w941, y=u16 0) -> (x = y?=w955:bool)
          n523 = Select(t=T9."Enabled" ("Disabled"), s=w955, f=T9."Disabled and Grayed Out") -> (s? t:f=w952:T9)
          n524 = property on="Create analysis file" class="Bool (strict)"("DisabledEnum"=w952) -> ()  [unwired: 2 in, 2 out]
          n525 = Equal?(x=w941, y=u16 1) -> (x = y?=w949:bool)
          n526 = Select(t=T9."Enabled" ("Disabled"), s=w949, f=T9."Disabled and Grayed Out") -> (s? t:f=w946:T9)
          n527 = property on="Save analyses file" class="Bool (strict)"("DisabledEnum"=w946) -> ()  [unwired: 2 in, 2 out]
          n528 = Equal?(x=w941, y=u16 2) -> (x = y?=w944:bool)
          n529 = Select(t=T9."Enabled" ("Disabled"), s=w944, f=T9."Disabled and Grayed Out") -> (s? t:f=w940:T9)
          n530 = property on="Next data file/exit program" class="Bool (strict)"("DisabledEnum"=w940) -> ()  [unwired: 2 in, 2 out]
          n531 = Replace Array Subset(array=w937, new element=w936, index=1 ("Index")) -> (w935:T13)
          n532 = Unbundle(w933) -> (w926:bool[], w928:dbl[][], w929:dbl[], w930:cluster{string[], bool[]}, w931:dbl[][], w932:cluster{dbl, string}[])
        }
        frame "Calibration" {
          n533 = Bundle(w1202, w1196, w1195) -> (w1201:cluster{dbl[][], dbl[], cluster{dbl, string}[]})  [unwired: 1 in]
          n534 = case shown="\"SISE channel 1\", Default" "Calibration-channel SISE1/2" {
            tunnel: w1197 -> [w1219 w1677]
            tunnel: [w1234 w1678] -> w1203
            tunnel: w1201 -> [w1236 w1682]
            tunnel: [w1233 w1681] -> w1200
            tunnel: w1195 -> [w1235 w1680]
            tunnel: [w1220 w1665] -> w1194
            tunnel: w1193 -> [w1218 w1656]
            tunnel: TRUE -> [w1210 w1660]
            tunnel: w1188 -> [w1205 w1651]
            tunnel: [w1206 w1650] -> w1187
            frame "SISE channel 1", Default {
              n535 = Unbundle(w1218) -> (w1216:bool[])  [unwired: 1 out]
              n536 = local read "Anal. method ch1"() -> (w1212:bool)
              n537 = local read "Calibration ch1"() -> (w1213:bool)
              n538 = Unbundle(w1218) -> (w1231:bool[])  [unwired: 1 out]
              n539 = local read "Geometry ch1"() -> (w1214:bool)
              n540 = Index Array(array=w1216, index=6) -> (element=w1215:bool)
              n541 = Index Array(array=w1231, index=8 ("Index")) -> (element=w1221:bool)
              n542 = Build Array(w1212, w1213, w1214, w1215) -> (w1211:bool[])
              n543 = for {
                tunnel: w1211 -> [w1259] mode=indexing
                shift-right: [w1257] -> w1207
                shift-left: w1210 -> [w1258]
                n544 = case shown="False" w1259 {
                  tunnel: w1258 -> [_ w1261]
                  tunnel: [FALSE w1261] -> w1257
                  frame False {
                  }
                  frame True {
                  }
                }
              }
              n545 = case shown="True" w1207 {
                tunnel: [T11."empty loop" ("Analysis method (Calibration window channel 1)") w1256] -> w1209
                tunnel: "Analysis method (Calibration window channel 1)" -> [_ w1256]
                frame False {
                }
                frame True {
                }
              }
              n546 = case shown="\"Update graphs\"" "Module selection (Calibration window channel 1)" {
                tunnel: dbl[][] [] -> [_ _ _ w1407]
                tunnel: w1207 -> [_ _ _ w1387]
                tunnel: [0 1 2 3] -> w1239
                tunnel: w1219 -> [_ _ _ w1388]
                tunnel: [w1270 w1315 w1325 w1386] -> w1234
                tunnel: [w1271 w1316 w1326 w1383] -> w1233
                tunnel: w1236 -> [w1271 w1316 w1326 w1383]
                tunnel: w1235 -> [_ _ _ w1389]
                tunnel: w1219 -> [w1270 w1315 w1325 w1367]
                tunnel: w1218 -> [w1269 w1314 w1324 w1385]
                tunnel: [w1269 w1314 w1324 w1384] -> w1220
                tunnel: "Analysis method (Calibration window channel 1)" -> [w1268 _ _ _]
                tunnel: w1209 -> [_ _ _ w1355]
                tunnel: w1207 -> [_ _ _ w1354]
                tunnel: [w1262 w1310 w1322 w1352] -> w1206
                tunnel: w1205 -> [w1262 w1310 w1322 w1353]
                frame "Analysis method", Default {
                  n547 = case shown="\"Diff. gradient\"" w1268 {
                    tunnel: "Ion Species ch1" -> [w1275 w1280]
                    tunnel: [w1274 w1281] -> w1266
                    frame "Chem. potential", Default {
                      n548 = Not Equal?(x=w1275, y=u16 0) -> (x != y?=w1277:bool)
                      n549 = Not Equal?(x="Ion conc. ch1 (mM)", y=u16 0) -> (x != y?=w1279:bool)
                      n550 = And(x=w1277, y=w1279) -> (x .and. y?=w1274:bool)
                    }
                    frame "Diff. gradient" {
                      n551 = Not Equal?(x=w1280, y=u16 0) -> (x != y?=w1281:bool)
                    }
                  }
                  "Anal. method ch1" <- w1266
                  n552 = case shown="8" "Ion Species ch1" {
                    tunnel: [0.0 36.4 7.6 7.6 5.2 7.9 7.4 3.1 2.7] -> w1263
                    tunnel: [0.0 1.0 1.0 1.0 1.0 1.0 1.0 2.0 2.0] -> w1264
                    tunnel: [0.0 9.3 2.0 2.0 1.3 2.0 1.9 0.8 0.7] -> w1265
                    frame 0, Default {
                    }
                    frame 1 {
                      # "H+"
                    }
                    frame 2 {
                      # "K+"
                    }
                    frame 3 {
                      # "NH4+"
                    }
                    frame 4 {
                      # "Na+"
                    }
                    frame 5 {
                      # "Cl-"
                    }
                    frame 6 {
                      # "NO3-"
                    }
                    frame 7 {
                      # "Ca2+"
                    }
                    frame 8 {
                      # "Mg2+"
                    }
                  }
                  "Ion mobilty ch1" <- w1263
                  "Valence ch1" <- w1264
                  "Diff. coeff. ch1" <- w1265
                }
                frame "Calibrate" {
                  n553 = call "Calibration-Fit-(SubVI).vi"("Array in"="Array in") -> ("intercept"=→"Intercept ch1":dbl, "slope"=w1313:dbl, "Array out"=→"?":cluster{dbl[], "Best Linear Fit":dbl[]}[], "Array 3"=→"Point #":dbl[])  [unwired: 7 in]
                  "Slope ch1" <- w1313
                  n554 = Not A Number/Path/Refnum?(number/path/refnum=w1313) -> (NaN/Path/Refnum?=w1312:bool)
                  n555 = Not(x=w1312) -> (.not. x?=→"Calibration ch1":bool)
                }
                frame "Geometry" {
                  n556 = local write "Tab Control Geo 2"("Tab Control Geo 1") -> ()
                  n557 = case shown="\"sphere\"" "Tab Control Geo 1" {
                    tunnel: ["Scan Distance  Flat (µm) 1" w1335 w1350] -> w1329
                    frame "flat surface", Default {
                      n558 = local write "Scan Distance  Flat (µm) 2"("Scan Distance  Flat (µm) 1") -> ()
                    }
                    frame "cylinder" {
                      n559 = local write "Scan distance cyl. (µm) 2"("Scan distance cyl. (µm) 1") -> ()
                      n560 = local write "Radius of object cyl. (µm) 2"("Radius of object cyl. (µm) 1") -> ()
                      n561 = local write "Minimum distance to object cyl. (µm) 2"("Minimum distance to object cyl. (µm) 1") -> ()
                      n562 = Add(x="Minimum distance to object cyl. (µm) 1", y="Radius of object cyl. (µm) 1") -> (x+y=w1338:dbl)
                      n563 = Add(x=w1338, y="Scan distance cyl. (µm) 1") -> (x+y=w1339:dbl)
                      n564 = Divide(x=w1339, y=w1338) -> (x/y=w1337:dbl)
                      n565 = Natural Logarithm(1:w1337) -> (0:w1336:dbl)
                      n566 = Multiply(x=w1336, y="Radius of object cyl. (µm) 1") -> (x*y=w1335:dbl)
                    }
                    frame "sphere" {
                      n567 = local write "Scan distance sphere (µm) 2"("Scan distance sphere (µm) 1") -> ()
                      n568 = local write "Radius of object sphere (µm) 2"("Radius of object sphere (µm) 1") -> ()
                      n569 = local write "Minimum distance to object sphere (µm) 2"("Minimum distance to object sphere (µm) 1") -> ()
                      n570 = Add(x="Minimum distance to object sphere (µm) 1", y="Radius of object sphere (µm) 1") -> (x+y=w1345:dbl)
                      n571 = Add(x=w1345, y="Scan distance sphere (µm) 1") -> (x+y=w1346:dbl)
                      n572 = Divide(x=1.0, y=w1345) -> (x/y=w1348:dbl)
                      n573 = Square(x="Radius of object sphere (µm) 1") -> (x^2=w1349:dbl)
                      n574 = Divide(x=1.0, y=w1346) -> (x/y=w1344:dbl)
                      n575 = Subtract(x=w1348, y=w1344) -> (x-y=w1343:dbl)
                      n576 = Multiply(x=w1343, y=w1349) -> (x*y=w1350:dbl)
                    }
                  }
                  "Corrected \ndistance ch1" <- w1329
                  n577 = Not Equal?(x=w1329, y=0.0) -> (x != y?=→"Geometry ch1":bool)
                }
                frame "Update graphs" {
                  n578 = for {
                    tunnel: w1389 -> [w1500] mode=indexing
                    shift-right: [w1502] -> w1404
                    shift-left: dbl[] [] -> [w1501]
                    n579 = Unbundle(w1500) -> (w1497:dbl)  [unwired: 1 out]
                    n580 = Divide(x=w1497, y=60.0) -> (x/y=w1498:dbl)
                    n581 = Insert Into Array(array=w1501, new element=w1498) -> (w1502:dbl[])  [unwired: 1 in]
                  }
                  n582 = local write "Zoom from start (Cal. modul) 2"("Zoom from start (Cal. modul) ch1") -> ()
                  n583 = Multiply(x="Zoom from end (Cal. modul) ch1", y=-1.0) -> (x*y=w1363:dbl)
                  n584 = case shown="\"Diff. gradient\"" w1355 {
                    tunnel: w1407 -> [w1539 w1612 _]
                    tunnel: w1388 -> [w1510 w1599 w1648]
                    tunnel: [w1527 w1604 w1648] -> w1386
                    tunnel: w1385 -> [w1517 w1581 w1649]
                    tunnel: [w1515 w1580 w1649] -> w1384
                    tunnel: w1353 -> [w1506 w1577 w1647]
                    tunnel: [w1503 w1576 w1647] -> w1352
                    frame "Chem. potential", Default {
                      w1516 = TRUE
                      w1534 = 1000000000.0  # Scaling, nmol m-2 s-1
                      w1536 = -58.0  # Nernst slope
                      n585 = Index Array(array=w1510, index (col)=2 ("Deaktivierter Index (Spalte)")) -> (element=w1509:dbl[])  [unwired: 1 in]
                      n586 = Index Array(array=w1510, index (col)=7 ("Deaktivierter Index (Spalte)")) -> (element=w1508:dbl[])  [unwired: 1 in]
                      n587 = Index Array(array=w1510, index (col)=6 ("Deaktivierter Index (Spalte)")) -> (element=w1507:dbl[])  [unwired: 1 in]
                      n588 = for {
                        tunnel: w1508 -> [w1544] mode=indexing
                        tunnel: [w1543] -> w1514 mode=indexing
                        tunnel: w1507 -> [w1542] mode=indexing
                        n589 = Subtract(x=w1544, y=w1542) -> (x-y=w1543:dbl)
                      }
                      n590 = Replace Array Subset(array=w1506, new element=TRUE ("new element/subarray"), index=0) -> (w1503:bool[])
                      n591 = local read "Corrected \ndistance ch1"() -> (w1535:dbl)
                      n592 = local read "Ion conc. ch1 (mM)"() -> (w1533:dbl)
                      n593 = local read "Ion mobilty ch1"() -> (w1538:dbl)
                      n594 = Unbundle(w1517) -> (w1518:string[], w1523:bool[])
                      n595 = local read "Intercept ch1"() -> (w1541:dbl)
                      n596 = local read "Valence ch1"() -> (w1537:dbl)
                      n597 = local read "Slope ch1"() -> (w1540:dbl)
                      n598 = for {
                        tunnel: w1509 -> [w1549] mode=indexing
                        tunnel: w1541 -> [w1566]
                        tunnel: w1540 -> [w1546]
                        shift-right: [w1570] -> w1526
                        shift-left: w1539 -> [w1571]
                        tunnel: w1538 -> [w1565]
                        tunnel: w1537 -> [w1555]
                        tunnel: w1536 -> [w1562]
                        tunnel: w1535 -> [w1559]
                        tunnel: w1534 -> [w1552]
                        tunnel: w1533 -> [w1550]
                        tunnel: w1514 -> [w1548] mode=indexing
                        # "dV / dx : mV / mm"
                        n599 = Divide(x=w1562, y=w1555) -> (x/y=w1561:dbl)
                        n600 = Divide(x=w1559, y=1000.0) -> (x/y=w1557:dbl)
                        n601 = Multiply(x=w1565, y=1e-08) -> (x*y=w1551:dbl)
                        n602 = Subtract(x=w1549, y=w1566) -> (x-y=w1574:dbl)
                        n603 = Divide(x=w1574, y=w1546) -> (x/y=w1573:dbl)
                        n604 = Divide(x=w1548, y=w1557) -> (x/y=w1554:dbl)
                        n605 = Multiply(x=w1550, y=w1551) -> (x*y=w1545:dbl)
                        n606 = Divide(x=w1561, y=w1546) -> (x/y=w1560:dbl)
                        n607 = Multiply(x=-1.0, y=w1573) -> (x*y=w1572:dbl)
                        n608 = Multiply(x=w1545, y=w1560) -> (x*y=w1556:dbl)
                        n609 = Power Of 10(x=w1572) -> (10^x=w1567:dbl)
                        n610 = Multiply(x=w1556, y=w1554) -> (x*y=w1553:dbl)
                        n611 = Multiply(x=w1553, y=w1552) -> (x*y=w1547:dbl)
                        n612 = Multiply(x=w1567, y=1000.0) -> (x*y=w1563:dbl)
                        n613 = Build Array(w1563, w1547) -> (w1569:dbl[])
                        n614 = Insert Into Array(array=w1571, new element=w1569) -> (w1570:dbl[][])  [unwired: 2 in]
                      }
                      n615 = Replace Array Subset(array=w1523, new element=w1516, index=10 ("Index")) -> (w1520:bool[])
                      n616 = Replace Array Subset(array=w1520, new element=w1516, index=12 ("Index")) -> (w1519:bool[])
                      n617 = Bundle(w1518, w1519) -> (w1515:cluster{string[], bool[]})  [unwired: 1 in]
                      n618 = Index Array(array=w1526, index (col)=0 ("Deaktivierter Index (Spalte)")) -> (element=w1532:dbl[])  [unwired: 1 in]
                      n619 = Replace Array Subset(array=w1510, new element=w1532, index (col)=10 ("Deaktivierter Index (Spalte)")) -> (w1528:dbl[][])  [unwired: 1 in]
                      n620 = Index Array(array=w1526, index (col)=1 ("Deaktivierter Index (Spalte)")) -> (element=w1531:dbl[])  [unwired: 1 in]
                      n621 = Replace Array Subset(array=w1528, new element=w1531, index (col)=12 ("Deaktivierter Index (Spalte)")) -> (w1527:dbl[][])  [unwired: 1 in]
                    }
                    frame "Diff. gradient" {
                      w1584 = TRUE
                      # "Diff. coeff. (x 10^9)"
                      n622 = Index Array(array=w1599, index (col)=2 ("Deaktivierter Index (Spalte)")) -> (element=w1598:dbl[])  [unwired: 1 in]
                      n623 = Index Array(array=w1599, index (col)=6 ("Deaktivierter Index (Spalte)")) -> (element=w1597:dbl[])  [unwired: 1 in]
                      n624 = Index Array(array=w1599, index (col)=7 ("Deaktivierter Index (Spalte)")) -> (element=w1596:dbl[])  [unwired: 1 in]
                      n625 = local read "Intercept ch1"() -> (w1594:dbl)
                      n626 = Unbundle(w1581) -> (w1582:string[], w1588:bool[])
                      n627 = local read "Slope ch1"() -> (w1593:dbl)
                      n628 = Build Array(w1598, w1597, w1596) -> (w1595:dbl[][])
                      n629 = Replace Array Subset(array=w1577, new element=FALSE ("new element/subarray"), index=0) -> (w1576:bool[])
                      n630 = for {
                        tunnel: w1595 -> [w1619] mode=indexing
                        tunnel: w1594 -> [w1618]
                        tunnel: w1593 -> [w1617]
                        shift-right: [w1615] -> w1589
                        shift-left: dbl[][] [] -> [w1616]
                        i -> [w1613]
                        n631 = for {
                          tunnel: w1619 -> [w1623] mode=indexing
                          tunnel: [w1621] -> w1614 mode=indexing
                          tunnel: w1618 -> [w1624]
                          tunnel: w1617 -> [w1622]
                          n632 = Subtract(x=w1623, y=w1624) -> (x-y=w1627:dbl)
                          n633 = Divide(x=w1627, y=w1622) -> (x/y=w1628:dbl)
                          n634 = Multiply(x=-1.0, y=w1628) -> (x*y=w1629:dbl)
                          n635 = Power Of 10(x=w1629) -> (10^x=w1620:dbl)
                          n636 = Multiply(x=w1620, y=1000.0) -> (x*y=w1621:dbl)
                        }
                        n637 = Insert Into Array(array=w1616, index (col)=w1613, new element=w1614) -> (w1615:dbl[][])  [unwired: 1 in]
                      }
                      n638 = Replace Array Subset(array=w1588, new element=w1584, index=10 ("Index")) -> (w1585:bool[])
                      n639 = Replace Array Subset(array=w1585, new element=w1584, index=12 ("Index")) -> (w1583:bool[])
                      n640 = Bundle(w1582, w1583) -> (w1580:cluster{string[], bool[]})  [unwired: 1 in]
                      n641 = local read "Corrected \ndistance ch1"() -> (w1591:dbl)
                      n642 = local read "Diff. coeff. ch1"() -> (w1592:dbl)
                      n643 = for {
                        shift-right: [w1646] -> w1603
                        shift-left: w1612 -> [w1645]
                        tunnel: w1592 -> [w1634]
                        tunnel: w1591 -> [w1638]
                        tunnel: w1589 -> [w1630] mode=indexing
                        # "J x 10^9"
                        # "dc / dx : mol m3 / m"
                        n644 = Index Array(array=w1630, index=0 ("Deaktivierter Index (Spalte)")) -> (element=w1632:dbl)
                        n645 = Index Array(array=w1630, index=2 ("Deaktivierter Index (Spalte)")) -> (element=w1641:dbl)
                        n646 = Index Array(array=w1630, index=1 ("Deaktivierter Index (Spalte)")) -> (element=w1640:dbl)
                        n647 = Divide(x=w1638, y=1000000.0) -> (x/y=w1636:dbl)
                        n648 = Subtract(x=w1641, y=w1640) -> (x-y=w1639:dbl)
                        n649 = Divide(x=w1639, y=w1636) -> (x/y=w1635:dbl)
                        n650 = Multiply(x=w1635, y=w1634) -> (x*y=w1631:dbl)
                        n651 = Build Array(w1632, w1631) -> (w1633:dbl[])
                        n652 = Insert Into Array(array=w1645, new element=w1633) -> (w1646:dbl[][])  [unwired: 2 in]
                      }
                      n653 = Index Array(array=w1603, index (col)=0 ("Deaktivierter Index (Spalte)")) -> (element=w1611:dbl[])  [unwired: 1 in]
                      n654 = Replace Array Subset(array=w1599, new element=w1611, index (col)=10 ("Deaktivierter Index (Spalte)")) -> (w1607:dbl[][])  [unwired: 1 in]
                      n655 = Index Array(array=w1603, index (col)=1 ("Deaktivierter Index (Spalte)")) -> (element=w1610:dbl[])  [unwired: 1 in]
                      n656 = Replace Array Subset(array=w1607, new element=w1610, index (col)=12 ("Deaktivierter Index (Spalte)")) -> (w1604:dbl[][])  [unwired: 1 in]
                    }
                    frame "empty loop" {
                    }
                  }
                  n657 = local write "Zoom from end (Cal. modul) 2"("Zoom from end (Cal. modul) ch1") -> ()
                  n658 = Add(x="Zoom from start (Cal. modul) ch1", y=w1363) -> (x+y=w1366:dbl)
                  n659 = Greater Or Equal?(x=w1366, y=0.0) -> (x >= y?=w1365:bool)
                  n660 = feedback #3() -> (w1364:dbl)  [unwired: 1 in]
                  n661 = case shown="True" w1365 {
                    tunnel: "Zoom from start (Cal. modul) ch1" -> [w1410 w1413]
                    tunnel: [w1409 w1413] -> w1358
                    tunnel: w1364 -> [w1409 w1415]
                    tunnel: "Zoom from end (Cal. modul) ch1" -> [_ w1412]
                    tunnel: [w1410 w1413] -> w1360
                    tunnel: [w1408 w1411] -> w1359
                    tunnel: "Zoom from end (Cal. modul) ch1" -> [w1408 w1411]
                    frame False {
                    }
                    frame True {
                      n662 = Not Equal?(x=w1415, y=w1413) -> (x != y?=w1414:bool)
                      n663 = case shown="False" w1414 {
                        tunnel: w1413 -> [_ w1417]
                        tunnel: w1412 -> [w1416 _]
                        frame False {
                          n664 = local write "Zoom from start (Cal. modul) ch1"(w1416) -> ()
                        }
                        frame True {
                          n665 = local write "Zoom from end (Cal. modul) ch1"(w1417) -> ()
                        }
                      }
                    }
                  }
                  n666 = feedback-in #3(w1358) -> ()
                  n667 = Array Size(array=w1389) -> (size(s)=w1393:i32)
                  n668 = Divide(x=w1393, y=10) -> (x/y=w1394:dbl)
                  n669 = Multiply(x=w1394, y="Bildlaufleiste") -> (x*y=w1396:dbl)
                  n670 = Array Subset(array=w1389, index=w1396) -> (w1397:cluster{dbl, string}[])  [unwired: 1 in]
                  n671 = Subtract(x=w1359, y=w1360) -> (x-y=w1381:dbl)
                  n672 = Index Array(array=w1367, index (col)=0 ("Deaktivierter Index (Spalte)")) -> (element=w1382:dbl[])  [unwired: 1 in]
                  n673 = for {
                    shift-right: [w1427] -> w1392
                    shift-left: "" -> [w1428]
                    tunnel: w1397 -> [w1426] mode=indexing
                    n674 = Unbundle(w1426) -> (w1424:dbl, w1421:string)
                    n675 = Divide(x=w1424, y=60.0) -> (x/y=w1422:dbl)
                    n676 = Number To Fractional String(number=w1422, precision (6)=i16 2 ("Genauigkeit (6)")) -> (F-format string=w1420:string)  [unwired: 2 in]
                    n677 = Concatenate Strings(w1428, w1420, "min. ,", w1421, "\r") -> (w1427:string)
                  }
                  "?" <- w1392
                  n678 = Divide(x=w1360, y=100.0) -> (x/y=w1379:dbl)
                  n679 = Divide(x=w1381, y=100.0) -> (x/y=w1380:dbl)
                  n680 = Array Size(array=w1382) -> (size(s)=w1378:i32)
                  n681 = Multiply(x=w1378, y=w1379) -> (x*y=w1375:dbl)
                  n682 = Multiply(x=w1378, y=w1380) -> (x*y=w1377:dbl)
                  n683 = Subtract(x=w1375, y=2.0) -> (x-y=w1374:dbl)
                  n684 = Add(x=w1377, y=2.0) -> (x+y=w1376:dbl)
                  n685 = Array Subset(array=w1367, index (row)=w1374, length (row)=w1376) -> (w1368:dbl[][])  [unwired: 2 in]
                  n686 = Index Array(array=w1368, index (col)=0 ("disabled index (col)")) -> (element=w1401:dbl[])  [unwired: 1 in]
                  n687 = Index Array(array=w1368, index (col)=10 ("disabled index (col)")) -> (element=w1400:dbl[])  [unwired: 1 in]
                  n688 = Index Array(array=w1368, index (col)=12 ("disabled index (col)")) -> (element=w1398:dbl[])  [unwired: 1 in]
                  n689 = stacked-sequence {
                    tunnel: w1401 -> [w1430 w1469]
                    tunnel: w1400 -> [w1449 _]
                    tunnel: w1404 -> [w1431 w1463]
                    tunnel: w1398 -> [_ w1468]
                    tunnel: w1387 -> [w1429 w1464]
                    frame #0 {
                      n690 = Array Max & Min(array=w1430) -> (max value=w1441:dbl, min value=w1440:dbl)  [unwired: 2 out]
                      n691 = Divide(x="Range limit\nS1.3 (mM)", y=2.0) -> (x/y=w1459:dbl)
                      n692 = Divide(x="Range limit\nS1.3 (mM)", y=2.05) -> (x/y=w1460:dbl)
                      n693 = Add(x="Base line\nS1.3 (mM)", y=w1459) -> (x+y=w1432:dbl)
                      n694 = Subtract(x="Base line\nS1.3 (mM)", y=w1459) -> (x-y=w1433:dbl)
                      n695 = Subtract(x="Base line\nS1.3 (mM)", y=w1460) -> (x-y=w1439:dbl)
                      n696 = call "EventstoGraph (SubVI).vi"("Numerisch 2"=w1440, "Array 3"=w1431, "Numerisch"=w1441, "Array (Eingang)"=dbl[][] [], "Numerisch 3"=w1439) -> ("Array (Ausgang)"=w1443:dbl[][])  [unwired: 6 in]
                      n697 = Array Max & Min(array=w1430) -> (max value=w1455:dbl, min value=w1456:dbl)  [unwired: 2 out]
                      n698 = call "GraphLimit01.vi"("Numeric 2"=w1433, "Numeric"=w1432, "Array in"=w1449, "Array 3"=dbl[] []) -> ("Array out"=w1448:dbl[])  [unwired: 7 in]
                      n699 = Build Array("Base line\nS1.3 (mM)", "Base line\nS1.3 (mM)") -> (w1452:dbl[])
                      n700 = Build Array(w1455, w1456) -> (w1453:dbl[])
                      n701 = Build Array(w1432, w1433) -> (w1454:dbl[])
                      n702 = Index Array(array=w1443, index (col)=0 ("Index (Zeile)")) -> (element=w1444:dbl[])  [unwired: 1 in]
                      n703 = Index Array(array=w1443, index (col)=1 ("Index (Zeile)")) -> (element=w1442:dbl[])  [unwired: 1 in]
                      n704 = Bundle(w1453, w1454) -> (w1436:cluster{dbl[], dbl[]})  [unwired: 1 in]
                      n705 = Bundle(w1453, w1452) -> (w1437:cluster{dbl[], dbl[]})  [unwired: 1 in]
                      n706 = Bundle(w1430, "Array out"=w1448) -> (w1435:cluster{dbl[], "Array out":dbl[]})  [unwired: 1 in]
                      n707 = Bundle("Array (Ausgang)"=w1444, "Array (Ausgang)"=w1442) -> (w1434:T17)  [unwired: 1 in]
                      n708 = Build Array(w1437, w1436, w1435, w1434) -> (w1438:T18)
                      n709 = case shown="True" w1429 {
                        tunnel: w1438 -> [_ w1462]
                        frame False {
                        }
                        frame True {
                          "Ion conc. SISE channel 1" <- w1462
                        }
                      }
                    }
                    frame #1 {
                      n710 = Array Max & Min(array=w1469) -> (max value=w1478:dbl, min value=w1477:dbl)  [unwired: 2 out]
                      n711 = Divide(x="Range limit\nS1.4", y=2.0) -> (x/y=w1494:dbl)
                      n712 = Divide(x="Range limit\nS1.4", y=2.05) -> (x/y=w1495:dbl)
                      n713 = Add(x="Base line \nS1.4", y=w1494) -> (x+y=w1470:dbl)
                      n714 = Subtract(x="Base line \nS1.4", y=w1494) -> (x-y=w1471:dbl)
                      n715 = Subtract(x="Base line \nS1.4", y=w1495) -> (x-y=w1476:dbl)
                      n716 = call "EventstoGraph (SubVI).vi"("Numerisch 2"=w1477, "Array 3"=w1463, "Numerisch"=w1478, "Array (Eingang)"=dbl[][] [], "Numerisch 3"=w1476) -> ("Array (Ausgang)"=w1480:dbl[][])  [unwired: 6 in]
                      n717 = Array Max & Min(array=w1469) -> (max value=w1490:dbl, min value=w1491:dbl)  [unwired: 2 out]
                      n718 = call "GraphLimit01.vi"("Numeric 2"=w1471, "Numeric"=w1470, "Array in"=w1468, "Array 3"=dbl[] []) -> ("Array out"=w1485:dbl[])  [unwired: 7 in]
                      n719 = Build Array("Base line \nS1.4", "Base line \nS1.4") -> (w1487:dbl[])
                      n720 = Build Array(w1490, w1491) -> (w1488:dbl[])
                      n721 = Build Array(w1470, w1471) -> (w1489:dbl[])
                      n722 = Index Array(array=w1480, index (col)=0 ("Index (Zeile)")) -> (element=w1481:dbl[])  [unwired: 1 in]
                      n723 = Index Array(array=w1480, index (col)=1 ("Index (Zeile)")) -> (element=w1479:dbl[])  [unwired: 1 in]
                      n724 = Bundle(w1488, w1489) -> (w1474:cluster{dbl[], dbl[]})  [unwired: 1 in]
                      n725 = Bundle(w1488, w1487) -> (w1475:cluster{dbl[], dbl[]})  [unwired: 1 in]
                      n726 = Bundle(w1469, "Array out"=w1485) -> (w1473:cluster{dbl[], "Array out":dbl[]})  [unwired: 1 in]
                      n727 = Bundle("Array (Ausgang)"=w1481, "Array (Ausgang)"=w1479) -> (w1472:T17)  [unwired: 1 in]
                      n728 = Build Array(w1475, w1474, w1473, w1472) -> (w1465:T18)
                      n729 = case shown="True" w1464 {
                        tunnel: w1465 -> [_ w1496]
                        frame False {
                        }
                        frame True {
                          "Ion flux SISE channel 1" <- w1496
                        }
                      }
                    }
                  }
                  "Update graphs ch1" <- w1354
                }
              }
              n730 = Equal?(x=w1239, y=u16 0) -> (x = y?=w1229:bool)
              n731 = Or(x=w1221, y=w1229) -> (x .or. y?=w1228:bool)
              n732 = Select(t=T9."Enabled" ("Disabled"), s=w1228, f=T9."Disabled and Grayed Out") -> (s? t:f=w1254:T9)
              n733 = property on="Anal. method ch1" class="Bool (strict)"("DisabledEnum"=w1254) -> ()  [unwired: 2 in, 2 out]
              n734 = Equal?(x=w1239, y=u16 1) -> (x = y?=w1226:bool)
              n735 = Or(x=w1221, y=w1226) -> (x .or. y?=w1227:bool)
              n736 = Select(t=T9."Enabled" ("Disabled"), s=w1227, f=T9."Disabled and Grayed Out") -> (s? t:f=w1250:T9)
              n737 = property on="Calibration ch1" class="Bool (strict)"("DisabledEnum"=w1250) -> ()  [unwired: 2 in, 2 out]
              n738 = Equal?(x=w1239, y=u16 2) -> (x = y?=w1224:bool)
              n739 = Or(x=w1221, y=w1224) -> (x .or. y?=w1225:bool)
              n740 = Select(t=T9."Enabled" ("Disabled"), s=w1225, f=T9."Disabled and Grayed Out") -> (s? t:f=w1244:T9)
              n741 = property on="Geometry ch1" class="Bool (strict)"("DisabledEnum"=w1244) -> ()  [unwired: 2 in, 2 out]
              n742 = Equal?(x=w1239, y=u16 3) -> (x = y?=w1222:bool)
              n743 = Or(x=w1221, y=w1222) -> (x .or. y?=w1223:bool)
              n744 = Select(t=T9."Enabled" ("Disabled"), s=w1223, f=T9."Disabled and Grayed Out") -> (s? t:f=w1238:T9)
              n745 = property on="Update graphs ch1" class="Bool (strict)"("DisabledEnum"=w1238) -> ()  [unwired: 2 in, 2 out]
            }
            frame "SISE channel 2" {
              n746 = local read "Anal. method ch2"() -> (w1661:bool)
              n747 = Unbundle(w1656) -> (w1676:bool[])  [unwired: 1 out]
              n748 = Unbundle(w1656) -> (w1655:bool[])  [unwired: 1 out]
              n749 = local read "Calibration ch2"() -> (w1662:bool)
              n750 = local read "Geometry 2"() -> (w1663:bool)
              n751 = Index Array(array=w1655, index=8) -> (element=w1654:bool)
              n752 = Index Array(array=w1676, index=7 ("Index")) -> (element=w1666:bool)
              n753 = Build Array(w1661, w1662, w1663, w1654) -> (w1659:bool[])
              n754 = for {
                tunnel: w1659 -> [w1704] mode=indexing
                shift-right: [w1702] -> w1652
                shift-left: w1660 -> [w1703]
                n755 = case shown="True" w1704 {
                  tunnel: w1703 -> [_ w1706]
                  tunnel: [FALSE w1706] -> w1702
                  frame False {
                  }
                  frame True {
                  }
                }
              }
              n756 = case shown="False" w1652 {
                tunnel: "Analysis method (Calibration window channel 2)" -> [_ w1701]
                tunnel: [T11."empty loop" ("Analysis method (Calibration window channel 2)") w1701] -> w1658
                frame False {
                }
                frame True {
                }
              }
              n757 = case shown="\"Update graphs\"" "Module selection (Calibration window channel 2)" {
                tunnel: dbl[][] [] -> [_ _ _ w1801]
                tunnel: w1652 -> [_ _ _ w1835]
                tunnel: [0 1 2 3] -> w1684
                tunnel: w1677 -> [_ _ _ w1805]
                tunnel: [w1716 w1761 w1771 w1851] -> w1681
                tunnel: w1682 -> [w1716 w1761 w1771 w1851]
                tunnel: w1680 -> [_ _ _ w1834]
                tunnel: [w1715 w1760 w1770 w1802] -> w1678
                tunnel: w1677 -> [w1715 w1760 w1770 w1809]
                tunnel: w1656 -> [w1714 w1759 w1769 w1804]
                tunnel: [w1714 w1759 w1769 w1803] -> w1665
                tunnel: w1658 -> [_ _ _ w1800]
                tunnel: "Analysis method (Calibration window channel 2)" -> [w1708 _ _ _]
                tunnel: w1652 -> [_ _ _ w1799]
                tunnel: w1651 -> [w1707 w1755 w1767 w1798]
                tunnel: [w1707 w1755 w1767 w1797] -> w1650
                frame "Analysis method", Default {
                  n758 = case shown="\"Diff. gradient\"" w1708 {
                    tunnel: "Ion Species ch2" -> [w1720 w1725]
                    tunnel: [w1719 w1726] -> w1709
                    frame "Chem. potential", Default {
                      n759 = Not Equal?(x=w1720, y=u16 0) -> (x != y?=w1722:bool)
                      n760 = Not Equal?(x="Ion conc. ch2 (mM)", y=u16 0) -> (x != y?=w1724:bool)
                      n761 = And(x=w1722, y=w1724) -> (x .and. y?=w1719:bool)
                    }
                    frame "Diff. gradient" {
                      n762 = Not Equal?(x=w1725, y=u16 0) -> (x != y?=w1726:bool)
                    }
                  }
                  "Anal. method ch2" <- w1709
                  n763 = case shown="7" "Ion Species ch2" {
                    tunnel: [0.0 36.4 7.6 7.6 5.2 7.9 7.4 3.1 2.7] -> w1710
                    tunnel: [0.0 1.0 1.0 1.0 1.0 1.0 1.0 2.0 2.0] -> w1711
                    tunnel: [0.0 9.3 2.0 2.0 1.3 2.0 1.9 0.4 0.4] -> w1712
                    frame 0, Default {
                    }
                    frame 1 {
                      # "H+"
                    }
                    frame 2 {
                      # "K+"
                    }
                    frame 3 {
                      # "NH4+"
                    }
                    frame 4 {
                      # "Na+"
                    }
                    frame 5 {
                      # "Cl-"
                    }
                    frame 6 {
                      # "NO3-"
                    }
                    frame 7 {
                      # "Ca2+"
                    }
                    frame 8 {
                      # "Mg2+"
                    }
                  }
                  "Diff. coeff. ch2" <- w1712
                  "Ion mobilty ch2" <- w1710
                  "Valence ch2" <- w1711
                }
                frame "Calibrate" {
                  n764 = call "Calibration-Fit-(SubVI).vi"("Array in"="Array in 2") -> ("intercept"=→"Intercept ch2":dbl, "slope"=w1758:dbl, "Array out"=→"?":cluster{dbl[], "Best Linear Fit":dbl[]}[], "Array 3"=→"Point # 2":dbl[])  [unwired: 7 in]
                  "Slope ch2" <- w1758
                  n765 = Not A Number/Path/Refnum?(number/path/refnum=w1758) -> (NaN/Path/Refnum?=w1757:bool)
                  n766 = Not(x=w1757) -> (.not. x?=→"Calibration ch2":bool)
                }
                frame "Geometry" {
                  n767 = local write "Tab Control Geo 1"("Tab Control Geo 2") -> ()
                  n768 = case shown="\"flat surface\", Default" "Tab Control Geo 2" {
                    tunnel: ["Scan Distance  Flat (µm) 2" w1780 w1795] -> w1774
                    frame "flat surface", Default {
                      n769 = local write "Scan Distance  Flat (µm) 1"("Scan Distance  Flat (µm) 2") -> ()
                    }
                    frame "cylinder" {
                      n770 = Add(x="Minimum distance to object cyl. (µm) 2", y="Radius of object cyl. (µm) 2") -> (x+y=w1783:dbl)
                      n771 = local write "Scan distance cyl. (µm) 1"("Scan distance cyl. (µm) 2") -> ()
                      n772 = local write "Radius of object cyl. (µm) 1"("Radius of object cyl. (µm) 2") -> ()
                      n773 = local write "Minimum distance to object cyl. (µm) 1"("Minimum distance to object cyl. (µm) 2") -> ()
                      n774 = Add(x=w1783, y="Scan distance cyl. (µm) 2") -> (x+y=w1784:dbl)
                      n775 = Divide(x=w1784, y=w1783) -> (x/y=w1782:dbl)
                      n776 = Natural Logarithm(1:w1782) -> (0:w1781:dbl)
                      n777 = Multiply(x=w1781, y="Radius of object cyl. (µm) 2") -> (x*y=w1780:dbl)
                    }
                    frame "sphere" {
                      n778 = local write "Scan distance sphere (µm) 1"("Scan distance sphere (µm) 2") -> ()
                      n779 = local write "Radius of object sphere (µm) 1"("Radius of object sphere (µm) 2") -> ()
                      n780 = local write "Minimum distance to object sphere (µm) 1"("Minimum distance to object sphere (µm) 2") -> ()
                      n781 = Add(x="Minimum distance to object sphere (µm) 2", y="Radius of object sphere (µm) 2") -> (x+y=w1790:dbl)
                      n782 = Add(x=w1790, y="Scan distance sphere (µm) 2") -> (x+y=w1791:dbl)
                      n783 = Divide(x=1.0, y=w1790) -> (x/y=w1793:dbl)
                      n784 = Square(x="Radius of object sphere (µm) 2") -> (x^2=w1794:dbl)
                      n785 = Divide(x=1.0, y=w1791) -> (x/y=w1789:dbl)
                      n786 = Subtract(x=w1793, y=w1789) -> (x-y=w1788:dbl)
                      n787 = Multiply(x=w1788, y=w1794) -> (x*y=w1795:dbl)
                    }
                  }
                  "Corrected \ndistance ch2" <- w1774
                  n788 = Not Equal?(x=w1774, y=0.0) -> (x != y?=→"Geometry 2":bool)
                }
                frame "Update graphs" {
                  n789 = for {
                    tunnel: w1834 -> [w2092] mode=indexing
                    shift-right: [w2094] -> w1833
                    shift-left: dbl[] [] -> [w2093]
                    n790 = Unbundle(w2092) -> (w2089:dbl)  [unwired: 1 out]
                    n791 = Divide(x=w2089, y=60.0) -> (x/y=w2090:dbl)
                    n792 = Insert Into Array(array=w2093, new element=w2090) -> (w2094:dbl[])  [unwired: 1 in]
                  }
                  n793 = case shown="\"Chem. potential\", Default" w1800 {
                    tunnel: w1801 -> [w1889 w1962 _]
                    tunnel: w1805 -> [w1861 w1949 w1999]
                    tunnel: [w1877 w1954 w1999] -> w1802
                    tunnel: [w1866 w1931 w1998] -> w1803
                    tunnel: w1804 -> [w1857 w1930 w1998]
                    tunnel: w1798 -> [w1856 w1927 w1997]
                    tunnel: [w1853 w1926 w1997] -> w1797
                    frame "Chem. potential", Default {
                      w1867 = TRUE
                      w1884 = 1000000000.0  # Scaling, nmol m-2 s-1
                      w1886 = -58.0  # Nernst slope
                      n794 = Index Array(array=w1861, index (col)=3 ("Deaktivierter Index (Spalte)")) -> (element=w1860:dbl[])  [unwired: 1 in]
                      n795 = Index Array(array=w1861, index (col)=9 ("Deaktivierter Index (Spalte)")) -> (element=w1859:dbl[])  [unwired: 1 in]
                      n796 = Index Array(array=w1861, index (col)=8 ("Deaktivierter Index (Spalte)")) -> (element=w1858:dbl[])  [unwired: 1 in]
                      n797 = for {
                        tunnel: w1859 -> [w1894] mode=indexing
                        tunnel: [w1893] -> w1865 mode=indexing
                        tunnel: w1858 -> [w1892] mode=indexing
                        n798 = Subtract(x=w1894, y=w1892) -> (x-y=w1893:dbl)
                      }
                      n799 = Replace Array Subset(array=w1856, new element=TRUE ("new element/subarray"), index=1) -> (w1853:bool[])
                      n800 = local read "Corrected \ndistance ch2"() -> (w1885:dbl)
                      n801 = local read "Ion conc. ch2 (mM)"() -> (w1883:dbl)
                      n802 = local read "Ion mobilty ch2"() -> (w1888:dbl)
                      n803 = Unbundle(w1857) -> (w1868:string[], w1873:bool[])
                      n804 = local read "Intercept ch2"() -> (w1891:dbl)
                      n805 = local read "Valence ch2"() -> (w1887:dbl)
                      n806 = local read "Slope ch2"() -> (w1890:dbl)
                      n807 = for {
                        tunnel: w1860 -> [w1899] mode=indexing
                        tunnel: w1891 -> [w1916]
                        tunnel: w1890 -> [w1896]
                        shift-right: [w1920] -> w1876
                        shift-left: w1889 -> [w1921]
                        tunnel: w1888 -> [w1915]
                        tunnel: w1887 -> [w1905]
                        tunnel: w1886 -> [w1912]
                        tunnel: w1885 -> [w1909]
                        tunnel: w1884 -> [w1902]
                        tunnel: w1883 -> [w1900]
                        tunnel: w1865 -> [w1898] mode=indexing
                        # "dV / dx : mV / mm"
                        n808 = Divide(x=w1912, y=w1905) -> (x/y=w1911:dbl)
                        n809 = Divide(x=w1909, y=1000.0) -> (x/y=w1907:dbl)
                        n810 = Multiply(x=w1915, y=1e-08) -> (x*y=w1901:dbl)
                        n811 = Subtract(x=w1899, y=w1916) -> (x-y=w1924:dbl)
                        n812 = Divide(x=w1924, y=w1896) -> (x/y=w1923:dbl)
                        n813 = Divide(x=w1898, y=w1907) -> (x/y=w1904:dbl)
                        n814 = Multiply(x=w1900, y=w1901) -> (x*y=w1895:dbl)
                        n815 = Divide(x=w1911, y=w1896) -> (x/y=w1910:dbl)
                        n816 = Multiply(x=-1.0, y=w1923) -> (x*y=w1922:dbl)
                        n817 = Multiply(x=w1895, y=w1910) -> (x*y=w1906:dbl)
                        n818 = Power Of 10(x=w1922) -> (10^x=w1917:dbl)
                        n819 = Multiply(x=w1906, y=w1904) -> (x*y=w1903:dbl)
                        n820 = Multiply(x=w1903, y=w1902) -> (x*y=w1897:dbl)
                        n821 = Multiply(x=w1917, y=1000.0) -> (x*y=w1913:dbl)
                        n822 = Build Array(w1913, w1897) -> (w1919:dbl[])
                        n823 = Insert Into Array(array=w1921, new element=w1919) -> (w1920:dbl[][])  [unwired: 2 in]
                      }
                      n824 = Replace Array Subset(array=w1873, new element=w1867, index=11 ("Index")) -> (w1870:bool[])
                      n825 = Replace Array Subset(array=w1870, new element=w1867, index=13 ("Index")) -> (w1869:bool[])
                      n826 = Bundle(w1868, w1869) -> (w1866:cluster{string[], bool[]})  [unwired: 1 in]
                      n827 = Index Array(array=w1876, index (col)=0 ("Deaktivierter Index (Spalte)")) -> (element=w1882:dbl[])  [unwired: 1 in]
                      n828 = Replace Array Subset(array=w1861, new element=w1882, index (col)=11 ("Deaktivierter Index (Spalte)")) -> (w1878:dbl[][])  [unwired: 1 in]
                      n829 = Index Array(array=w1876, index (col)=1 ("Deaktivierter Index (Spalte)")) -> (element=w1881:dbl[])  [unwired: 1 in]
                      n830 = Replace Array Subset(array=w1878, new element=w1881, index (col)=13 ("Deaktivierter Index (Spalte)")) -> (w1877:dbl[][])  [unwired: 1 in]
                    }
                    frame "Diff. gradient" {
                      w1934 = TRUE
                      # "Diff. coell. (x 10^9)"
                      n831 = Index Array(array=w1949, index (col)=3 ("Deaktivierter Index (Spalte)")) -> (element=w1948:dbl[])  [unwired: 1 in]
                      n832 = Index Array(array=w1949, index (col)=8 ("Deaktivierter Index (Spalte)")) -> (element=w1947:dbl[])  [unwired: 1 in]
                      n833 = Index Array(array=w1949, index (col)=9 ("Deaktivierter Index (Spalte)")) -> (element=w1946:dbl[])  [unwired: 1 in]
                      n834 = local read "Intercept ch2"() -> (w1944:dbl)
                      n835 = Replace Array Subset(array=w1927, new element=FALSE ("new element/subarray"), index=1) -> (w1926:bool[])
                      n836 = Unbundle(w1930) -> (w1932:string[], w1938:bool[])
                      n837 = local read "Slope ch2"() -> (w1943:dbl)
                      n838 = Build Array(w1948, w1947, w1946) -> (w1945:dbl[][])
                      n839 = for {
                        tunnel: w1945 -> [w1969] mode=indexing
                        tunnel: w1944 -> [w1968]
                        tunnel: w1943 -> [w1967]
                        shift-right: [w1965] -> w1939
                        shift-left: dbl[][] [] -> [w1966]
                        i -> [w1963]
                        n840 = for {
                          tunnel: w1969 -> [w1972] mode=indexing
                          tunnel: [w1970] -> w1964 mode=indexing
                          tunnel: w1968 -> [w1973]
                          tunnel: w1967 -> [w1971]
                          n841 = Subtract(x=w1972, y=w1973) -> (x-y=w1976:dbl)
                          n842 = Divide(x=w1976, y=w1971) -> (x/y=w1977:dbl)
                          n843 = Multiply(x=-1.0, y=w1977) -> (x*y=w1978:dbl)
                          n844 = Power Of 10(x=w1978) -> (10^x=w1979:dbl)
                          n845 = Multiply(x=w1979, y=1000.0) -> (x*y=w1970:dbl)
                        }
                        n846 = Insert Into Array(array=w1966, index (col)=w1963, new element=w1964) -> (w1965:dbl[][])  [unwired: 1 in]
                      }
                      n847 = Replace Array Subset(array=w1938, new element=w1934, index=11 ("Index")) -> (w1935:bool[])
                      n848 = Replace Array Subset(array=w1935, new element=w1934, index=13 ("Index")) -> (w1933:bool[])
                      n849 = Bundle(w1932, w1933) -> (w1931:cluster{string[], bool[]})  [unwired: 1 in]
                      n850 = local read "Corrected \ndistance ch2"() -> (w1941:dbl)
                      n851 = local read "Diff. coeff. ch2"() -> (w1942:dbl)
                      n852 = for {
                        shift-right: [w1996] -> w1953
                        shift-left: w1962 -> [w1995]
                        tunnel: w1942 -> [w1984]
                        tunnel: w1941 -> [w1988]
                        tunnel: w1939 -> [w1980] mode=indexing
                        # "J x 10^9"
                        # "dc / dx : mol m3 / m"
                        n853 = Index Array(array=w1980, index=0 ("Deaktivierter Index (Spalte)")) -> (element=w1982:dbl)
                        n854 = Index Array(array=w1980, index=2 ("Deaktivierter Index (Spalte)")) -> (element=w1991:dbl)
                        n855 = Index Array(array=w1980, index=1 ("Deaktivierter Index (Spalte)")) -> (element=w1990:dbl)
                        n856 = Divide(x=w1988, y=1000000.0) -> (x/y=w1986:dbl)
                        n857 = Subtract(x=w1991, y=w1990) -> (x-y=w1989:dbl)
                        n858 = Divide(x=w1989, y=w1986) -> (x/y=w1985:dbl)
                        n859 = Multiply(x=w1985, y=w1984) -> (x*y=w1981:dbl)
                        n860 = Build Array(w1982, w1981) -> (w1983:dbl[])
                        n861 = Insert Into Array(array=w1995, new element=w1983) -> (w1996:dbl[][])  [unwired: 2 in]
                      }
                      n862 = Index Array(array=w1953, index (col)=0 ("Deaktivierter Index (Spalte)")) -> (element=w1961:dbl[])  [unwired: 1 in]
                      n863 = Replace Array Subset(array=w1949, new element=w1961, index (col)=11 ("Deaktivierter Index (Spalte)")) -> (w1957:dbl[][])  [unwired: 1 in]
                      n864 = Index Array(array=w1953, index (col)=1 ("Deaktivierter Index (Spalte)")) -> (element=w1960:dbl[])  [unwired: 1 in]
                      n865 = Replace Array Subset(array=w1957, new element=w1960, index (col)=13 ("Deaktivierter Index (Spalte)")) -> (w1954:dbl[][])  [unwired: 1 in]
                    }
                    frame "empty loop" {
                    }
                  }
                  n866 = local write "Zoom from start (Cal. modul) ch1"("Zoom from start (Cal. modul) 2") -> ()
                  n867 = Multiply(x="Zoom from end (Cal. modul) 2", y=-1.0) -> (x*y=w1815:dbl)
                  n868 = local write "Zoom from end (Cal. modul) ch1"("Zoom from end (Cal. modul) 2") -> ()
                  n869 = Add(x="Zoom from start (Cal. modul) 2", y=w1815) -> (x+y=w1818:dbl)
                  n870 = feedback #4() -> (w1816:dbl)  [unwired: 1 in]
                  n871 = Greater Or Equal?(x=w1818, y=0.0) -> (x >= y?=w1817:bool)
                  n872 = case shown="True" w1817 {
                    tunnel: "Zoom from start (Cal. modul) 2" -> [w2002 w2005]
                    tunnel: [w2001 w2005] -> w1810
                    tunnel: w1816 -> [w2001 w2007]
                    tunnel: "Zoom from end (Cal. modul) 2" -> [_ w2004]
                    tunnel: [w2002 w2005] -> w1812
                    tunnel: [w2000 w2003] -> w1811
                    tunnel: "Zoom from end (Cal. modul) 2" -> [w2000 w2003]
                    frame False {
                    }
                    frame True {
                      n873 = Not Equal?(x=w2007, y=w2005) -> (x != y?=w2006:bool)
                      n874 = case shown="True" w2006 {
                        tunnel: w2005 -> [_ w2009]
                        tunnel: w2004 -> [w2008 _]
                        frame False {
                          n875 = local write "Zoom from start (Cal. modul) 2"(w2008) -> ()
                        }
                        frame True {
                          n876 = local write "Zoom from end (Cal. modul) 2"(w2009) -> ()
                        }
                      }
                    }
                  }
                  n877 = feedback-in #4(w1810) -> ()
                  n878 = Array Size(array=w1834) -> (size(s)=w1839:i32)
                  n879 = Divide(x=w1839, y=10) -> (x/y=w1840:dbl)
                  n880 = Multiply(x=w1840, y="Bildlaufleiste 2") -> (x*y=w1842:dbl)
                  n881 = Array Subset(array=w1834, index=w1842) -> (w1843:cluster{dbl, string}[])  [unwired: 1 in]
                  n882 = Subtract(x=w1811, y=w1812) -> (x-y=w1831:dbl)
                  n883 = Index Array(array=w1809, index (col)=0 ("Deaktivierter Index (Spalte)")) -> (element=w1832:dbl[])  [unwired: 1 in]
                  n884 = for {
                    shift-right: [w2019] -> w1838
                    shift-left: "" -> [w2020]
                    tunnel: w1843 -> [w2018] mode=indexing
                    n885 = Unbundle(w2018) -> (w2016:dbl, w2013:string)
                    n886 = Divide(x=w2016, y=60.0) -> (x/y=w2014:dbl)
                    n887 = Number To Fractional String(number=w2014, precision (6)=i16 2 ("Genauigkeit (6)")) -> (F-format string=w2012:string)  [unwired: 2 in]
                    n888 = Concatenate Strings(w2020, w2012, "min. ,", w2013, "\r") -> (w2019:string)
                  }
                  "?" <- w1838
                  n889 = Divide(x=w1812, y=100.0) -> (x/y=w1829:dbl)
                  n890 = Divide(x=w1831, y=100.0) -> (x/y=w1830:dbl)
                  n891 = Array Size(array=w1832) -> (size(s)=w1828:i32)
                  n892 = Multiply(x=w1828, y=w1829) -> (x*y=w1825:dbl)
                  n893 = Multiply(x=w1828, y=w1830) -> (x*y=w1827:dbl)
                  n894 = Subtract(x=w1825, y=2.0) -> (x-y=w1824:dbl)
                  n895 = Add(x=w1827, y=2.0) -> (x+y=w1826:dbl)
                  n896 = Array Subset(array=w1809, index (row)=w1824, length (row)=w1826) -> (w1808:dbl[][])  [unwired: 2 in]
                  n897 = Index Array(array=w1808, index (col)=0 ("disabled index (col)")) -> (element=w1847:dbl[])  [unwired: 1 in]
                  n898 = Index Array(array=w1808, index (col)=11 ("disabled index (col)")) -> (element=w1846:dbl[])  [unwired: 1 in]
                  n899 = Index Array(array=w1808, index (col)=13 ("disabled index (col)")) -> (element=w1844:dbl[])  [unwired: 1 in]
                  n900 = stacked-sequence {
                    tunnel: w1847 -> [w2022 w2061]
                    tunnel: w1846 -> [w2041 _]
                    tunnel: w1833 -> [w2023 w2055]
                    tunnel: w1844 -> [_ w2060]
                    tunnel: w1835 -> [w2021 w2056]
                    frame #0 {
                      n901 = Array Max & Min(array=w2022) -> (max value=w2033:dbl, min value=w2032:dbl)  [unwired: 2 out]
                      n902 = Divide(x="Range limit\nS2.3 (mM)", y=2.0) -> (x/y=w2051:dbl)
                      n903 = Divide(x="Range limit\nS2.3 (mM)", y=2.05) -> (x/y=w2052:dbl)
                      n904 = Add(x="Base line\nS2.3 (mM)", y=w2051) -> (x+y=w2024:dbl)
                      n905 = Subtract(x="Base line\nS2.3 (mM)", y=w2051) -> (x-y=w2025:dbl)
                      n906 = Subtract(x="Base line\nS2.3 (mM)", y=w2052) -> (x-y=w2031:dbl)
                      n907 = call "EventstoGraph (SubVI).vi"("Numerisch 2"=w2032, "Array 3"=w2023, "Numerisch"=w2033, "Array (Eingang)"=dbl[][] [], "Numerisch 3"=w2031) -> ("Array (Ausgang)"=w2035:dbl[][])  [unwired: 6 in]
                      n908 = Array Max & Min(array=w2022) -> (max value=w2047:dbl, min value=w2048:dbl)  [unwired: 2 out]
                      n909 = call "GraphLimit01.vi"("Numeric 2"=w2025, "Numeric"=w2024, "Array in"=w2041, "Array 3"=dbl[] []) -> ("Array out"=w2040:dbl[])  [unwired: 7 in]
                      n910 = Build Array("Base line\nS2.3 (mM)", "Base line\nS2.3 (mM)") -> (w2044:dbl[])
                      n911 = Build Array(w2047, w2048) -> (w2045:dbl[])
                      n912 = Build Array(w2024, w2025) -> (w2046:dbl[])
                      n913 = Index Array(array=w2035, index (col)=0 ("Index (Zeile)")) -> (element=w2036:dbl[])  [unwired: 1 in]
                      n914 = Index Array(array=w2035, index (col)=1 ("Index (Zeile)")) -> (element=w2034:dbl[])  [unwired: 1 in]
                      n915 = Bundle(w2045, w2046) -> (w2028:cluster{dbl[], dbl[]})  [unwired: 1 in]
                      n916 = Bundle(w2045, w2044) -> (w2029:cluster{dbl[], dbl[]})  [unwired: 1 in]
                      n917 = Bundle(w2022, "Array out"=w2040) -> (w2027:cluster{dbl[], "Array out":dbl[]})  [unwired: 1 in]
                      n918 = Bundle("Array (Ausgang)"=w2036, "Array (Ausgang)"=w2034) -> (w2026:T17)  [unwired: 1 in]
                      n919 = Build Array(w2029, w2028, w2027, w2026) -> (w2030:T18)
                      n920 = case shown="True" w2021 {
                        tunnel: w2030 -> [_ w2054]
                        frame False {
                        }
                        frame True {
                          "Ion conc. SISE channel 2" <- w2054
                        }
                      }
                    }
                    frame #1 {
                      n921 = Array Max & Min(array=w2061) -> (max value=w2070:dbl, min value=w2069:dbl)  [unwired: 2 out]
                      n922 = Divide(x="Range limit\nS2.4", y=2.0) -> (x/y=w2086:dbl)
                      n923 = Divide(x="Range limit\nS2.4", y=2.05) -> (x/y=w2087:dbl)
                      n924 = Add(x="Base line \nS2.4", y=w2086) -> (x+y=w2062:dbl)
                      n925 = Subtract(x="Base line \nS2.4", y=w2086) -> (x-y=w2063:dbl)
                      n926 = Subtract(x="Base line \nS2.4", y=w2087) -> (x-y=w2068:dbl)
                      n927 = call "EventstoGraph (SubVI).vi"("Numerisch 2"=w2069, "Array 3"=w2055, "Numerisch"=w2070, "Array (Eingang)"=dbl[][] [], "Numerisch 3"=w2068) -> ("Array (Ausgang)"=w2072:dbl[][])  [unwired: 6 in]
                      n928 = Array Max & Min(array=w2061) -> (max value=w2082:dbl, min value=w2083:dbl)  [unwired: 2 out]
                      n929 = call "GraphLimit01.vi"("Numeric 2"=w2063, "Numeric"=w2062, "Array in"=w2060, "Array 3"=dbl[] []) -> ("Array out"=w2077:dbl[])  [unwired: 7 in]
                      n930 = Build Array("Base line \nS2.4", "Base line \nS2.4") -> (w2079:dbl[])
                      n931 = Build Array(w2082, w2083) -> (w2080:dbl[])
                      n932 = Build Array(w2062, w2063) -> (w2081:dbl[])
                      n933 = Index Array(array=w2072, index (col)=0 ("Index (Zeile)")) -> (element=w2073:dbl[])  [unwired: 1 in]
                      n934 = Index Array(array=w2072, index (col)=1 ("Index (Zeile)")) -> (element=w2071:dbl[])  [unwired: 1 in]
                      n935 = Bundle(w2080, w2081) -> (w2066:cluster{dbl[], dbl[]})  [unwired: 1 in]
                      n936 = Bundle(w2080, w2079) -> (w2067:cluster{dbl[], dbl[]})  [unwired: 1 in]
                      n937 = Bundle(w2061, "Array out"=w2077) -> (w2065:cluster{dbl[], "Array out":dbl[]})  [unwired: 1 in]
                      n938 = Bundle("Array (Ausgang)"=w2073, "Array (Ausgang)"=w2071) -> (w2064:T17)  [unwired: 1 in]
                      n939 = Build Array(w2067, w2066, w2065, w2064) -> (w2057:T18)
                      n940 = case shown="True" w2056 {
                        tunnel: w2057 -> [_ w2088]
                        frame False {
                        }
                        frame True {
                          "Ion flux SISE channel 2" <- w2088
                        }
                      }
                    }
                  }
                  "Update graphs ch2" <- w1799
                }
              }
              n941 = Equal?(x=w1684, y=u16 0) -> (x = y?=w1674:bool)
              n942 = Or(x=w1666, y=w1674) -> (x .or. y?=w1673:bool)
              n943 = Select(t=T9."Enabled" ("Disabled"), s=w1673, f=T9."Disabled and Grayed Out") -> (s? t:f=w1699:T9)
              n944 = property on="Anal. method ch2" class="Bool (strict)"("DisabledEnum"=w1699) -> ()  [unwired: 2 in, 2 out]
              n945 = Equal?(x=w1684, y=u16 1) -> (x = y?=w1671:bool)
              n946 = Or(x=w1666, y=w1671) -> (x .or. y?=w1672:bool)
              n947 = Select(t=T9."Enabled" ("Disabled"), s=w1672, f=T9."Disabled and Grayed Out") -> (s? t:f=w1695:T9)
              n948 = property on="Calibration ch2" class="Bool (strict)"("DisabledEnum"=w1695) -> ()  [unwired: 2 in, 2 out]
              n949 = Equal?(x=w1684, y=u16 2) -> (x = y?=w1669:bool)
              n950 = Or(x=w1666, y=w1669) -> (x .or. y?=w1670:bool)
              n951 = Select(t=T9."Enabled" ("Disabled"), s=w1670, f=T9."Disabled and Grayed Out") -> (s? t:f=w1689:T9)
              n952 = property on="Geometry 2" class="Bool (strict)"("DisabledEnum"=w1689) -> ()  [unwired: 2 in, 2 out]
              n953 = Equal?(x=w1684, y=u16 3) -> (x = y?=w1667:bool)
              n954 = Or(x=w1666, y=w1667) -> (x .or. y?=w1668:bool)
              n955 = Select(t=T9."Enabled" ("Disabled"), s=w1668, f=T9."Disabled and Grayed Out") -> (s? t:f=w1679:T9)
              n956 = property on="Update graphs ch2" class="Bool (strict)"("DisabledEnum"=w1679) -> ()  [unwired: 2 in, 2 out]
            }
          }
          n957 = Unbundle(w1200) -> (w1199:dbl[][], w1198:dbl[], w1190:cluster{dbl, string}[])
        }
        frame "Buffer correction" {
          n958 = Bundle(w2102, w2109, w2108, w2107) -> (w2106:T20)  [unwired: 1 in]
          n959 = case shown="\"SISE channel 2, buffer corr.\"" "SISE channel selection (buffer corr.)" {
            tunnel: w2103 -> [w2129 w2450]
            tunnel: w2096 -> [w2133 w2454]
            tunnel: [w2132 w2453] -> w2111
            tunnel: w2107 -> [w2130 w2452]
            tunnel: [w2131 w2451] -> w2110
            tunnel: w2103 -> [w2127 w2448]
            tunnel: TRUE -> [w2119 w2442]
            tunnel: w2096 -> [w2115 w2440]
            tunnel: w2095 -> [w2118 w2439]
            frame "SISE channel 2, buffer corr." {
              n960 = local read "Analysis method (Calibration window channel 2)"() -> (→"Tab Control 2":enum32{"Chem. potential", "Diff. gradient"})
              n961 = local read "Buffer species ch2"() -> (w2125:bool)
              n962 = local read "Buffer conc. ch2"() -> (w2124:bool)
              n963 = Unbundle(w2115) -> (w2122:bool[])  [unwired: 1 out]
              n964 = Index Array(array=w2118, index=1) -> (element=w2116:bool)
              n965 = Index Array(array=w2122, index=12) -> (element=w2123:bool)
              n966 = Build Array(w2125, w2124, w2123) -> (w2114:bool[])
              n967 = for {
                shift-right: [w2165] -> w2113
                shift-left: w2119 -> [w2166]
                tunnel: w2114 -> [w2164] mode=indexing
                n968 = case shown="True" w2164 {
                  tunnel: w2166 -> [_ w2168]
                  tunnel: [FALSE w2168] -> w2165
                  frame False {
                  }
                  frame True {
                  }
                }
              }
              "Update graphs (buffer corr.) ch2" <- w2113
              n969 = Unbundle(w2133) -> (w2143:bool[])  [unwired: 1 out]
              n970 = case shown="True" w2113 {
                tunnel: [0 w2161] -> w2117
                tunnel: w2116 -> [_ w2160]
                frame False {
                }
                frame True {
                  n971 = case shown="False" w2160 {
                    tunnel: [2 1] -> w2161
                    frame False {
                    }
                    frame True {
                    }
                  }
                }
              }
              n972 = Index Array(array=w2143, index=9 ("Index")) -> (element=w2141:bool)
              n973 = Index Array(array=w2143, index=11 ("Index")) -> (element=w2142:bool)
              n974 = And(x=w2141, y=w2142) -> (x .and. y?=w2134:bool)
              n975 = case shown="\"Update graphs\"" "Module selection ch2 (buffer corr.)" {
                tunnel: [0 1 2] -> w2146
                tunnel: w2129 -> [w2177 w2204 w2218]
                tunnel: [w2177 w2204 w2209] -> w2132
                tunnel: w2115 -> [w2176 w2203 w2217]
                tunnel: [w2176 w2203 w2210] -> w2131
                tunnel: w2130 -> [_ _ w2219]
                tunnel: w2113 -> [_ _ w2220]
                tunnel: w2127 -> [_ _ w2223]
                tunnel: w2117 -> [_ _ w2208]
                frame "Buffer species", Default {
                  n976 = case shown="\"none\", Default" "Select buffer ch 2" {
                    tunnel: ["" "Mes" "Malate (pH 5)" "Citrate (pH 5)" "TRIS" "HEPES"] -> w2173
                    tunnel: [0.0 6.2 5.1 4.8 8.2 7.5] -> w2172
                    tunnel: [0.0 2.9 3.2 2.5 3.2 2.4] -> w2171
                    tunnel: [0.0 0.7 0.8 0.6 0.8 0.6] -> w2170
                    frame "none", Default {
                    }
                    frame "Mes" {
                    }
                    frame "Malate (pH 5)" {
                    }
                    frame "Citrate (pH 5)" {
                    }
                    frame "TRIS" {
                    }
                    frame "HEPES" {
                    }
                  }
                  "pKs ch2" <- w2172
                  "Buffer Mobilty ch2" <- w2171
                  "Diff. coeff. buffer ch2" <- w2170
                  n977 = Not Equal?(x="", y=w2173) -> (x != y?=→"Buffer species ch2":bool)
                }
                frame "Buffer conc." {
                  n978 = Not Equal To 0?(x="Buffer conc. ch2 (mM)") -> (x != 0?=→"Buffer conc. ch2":bool)
                }
                frame "Update graphs" {
                  n979 = local read "Buffer conc. ch2 (mM)"() -> (w2213:dbl)
                  n980 = local read "Ion conc. ch2 (mM)"() -> (w2215:dbl)
                  n981 = local read "Buffer Mobilty ch2"() -> (w2212:dbl)
                  n982 = local read "Ion mobilty ch2"() -> (w2211:dbl)
                  n983 = local read "pKs ch2"() -> (w2214:dbl)
                  n984 = local write "Zoom from start (Buffer corr. modul) ch1"("Zoom from start (Buffer corr. modul) ch2") -> ()
                  n985 = local write "Zoom from end (Buffer corr. modul) ch1"("Zoom from end (Buffer corr. modul) ch2") -> ()
                  n986 = for {
                    tunnel: w2219 -> [w2397] mode=indexing
                    shift-right: [w2399] -> w2256
                    shift-left: dbl[] [] -> [w2398]
                    n987 = Unbundle(w2397) -> (w2394:dbl)  [unwired: 1 out]
                    n988 = Divide(x=w2394, y=60.0) -> (x/y=w2395:dbl)
                    n989 = Insert Into Array(array=w2398, new element=w2395) -> (w2399:dbl[])  [unwired: 1 in]
                  }
                  n990 = case shown="1" w2208 {
                    tunnel: w2212 -> [_ w2283 _]
                    tunnel: w2211 -> [_ w2284 _]
                    tunnel: w2214 -> [_ w2281 w2324]
                    tunnel: w2213 -> [_ w2280 w2325]
                    tunnel: w2215 -> [_ w2273 _]
                    tunnel: w2218 -> [w2264 w2268 w2312]
                    tunnel: [w2263 w2274 w2316] -> w2210
                    tunnel: [w2264 w2272 w2311] -> w2209
                    tunnel: dbl[] [] -> [_ w2266 w2322]
                    tunnel: w2217 -> [w2263 w2265 w2309]
                    frame 0, Default {
                    }
                    frame 1 {
                      n991 = Index Array(array=w2268, index (col)=13 ("Deaktivierter Index (Spalte)")) -> (element=w2267:dbl[])  [unwired: 1 in]
                      n992 = Divide(x=w2283, y=w2284) -> (x/y=w2282:dbl)
                      n993 = for {
                        tunnel: w2282 -> [w2293]
                        tunnel: w2281 -> [w2303]
                        tunnel: w2280 -> [w2297]
                        shift-right: [w2288] -> w2271
                        shift-left: w2266 -> [w2289]
                        tunnel: w2267 -> [w2287] mode=indexing
                        tunnel: w2273 -> [w2286]
                        n994 = Multiply(x=w2286, y=0.001) -> (x*y=w2307:dbl)
                        n995 = Multiply(x=w2297, y=0.001) -> (x*y=w2294:dbl)
                        n996 = Logarithm Base 10(1:w2307) -> (0:w2306:dbl)
                        n997 = Multiply(x=w2306, y=-1.0) -> (x*y=w2304:dbl)
                        n998 = Power Of 10(x=w2304) -> (10^x=w2301:dbl)
                        n999 = Power Of 10(x=w2303) -> (10^x=w2298:dbl)
                        n1000 = Add(x=w2301, y=w2298) -> (x+y=w2302:dbl)
                        n1001 = Divide(x=w2301, y=w2302) -> (x/y=w2300:dbl)
                        n1002 = Square(x=w2300) -> (x^2=w2299:dbl)
                        n1003 = Multiply(x=w2299, y=w2298) -> (x*y=w2295:dbl)
                        n1004 = Multiply(x=w2295, y=w2294) -> (x*y=w2292:dbl)
                        n1005 = Multiply(x=w2292, y=w2293) -> (x*y=w2291:dbl)
                        n1006 = Multiply(x=w2291, y=w2287) -> (x*y=w2290:dbl)
                        n1007 = Add(x=w2290, y=w2287) -> (x+y=w2285:dbl)
                        n1008 = Insert Into Array(array=w2289, new element=w2285) -> (w2288:dbl[])  [unwired: 1 in]
                      }
                      n1009 = Unbundle(w2265) -> (w2275:string[], w2278:bool[])
                      n1010 = Replace Array Subset(array=w2278, new element=TRUE, index=15 ("Index")) -> (w2279:bool[])
                      n1011 = Bundle(w2275, w2279) -> (w2274:cluster{string[], bool[]})  [unwired: 1 in]
                      n1012 = Replace Array Subset(array=w2268, new element=w2271, index (col)=15 ("Deaktivierter Index (Spalte)")) -> (w2272:dbl[][])  [unwired: 1 in]
                    }
                    frame 2 {
                      # "Diff. coeff. (x 10^9)"
                      n1013 = Index Array(array=w2312, index (col)=8 ("Deaktivierter Index (Spalte)")) -> (element=w2329:dbl[])  [unwired: 1 in]
                      n1014 = Index Array(array=w2312, index (col)=9 ("Deaktivierter Index (Spalte)")) -> (element=w2330:dbl[])  [unwired: 1 in]
                      n1015 = Build Array(w2329, w2330) -> (w2331:dbl[][])
                      n1016 = local read "Intercept ch2"() -> (w2332:dbl)
                      n1017 = local read "Slope ch2"() -> (w2333:dbl)
                      n1018 = for {
                        tunnel: w2331 -> [w2344] mode=indexing
                        tunnel: w2332 -> [w2343]
                        tunnel: w2333 -> [w2342]
                        shift-right: [w2340] -> w2323
                        shift-left: dbl[][] [] -> [w2341]
                        tunnel: w2325 -> [w2338]
                        tunnel: w2324 -> [w2337]
                        i -> [w2336]
                        n1019 = for {
                          tunnel: w2344 -> [w2354] mode=indexing
                          tunnel: [w2346] -> w2339 mode=indexing
                          tunnel: w2343 -> [w2355]
                          tunnel: w2342 -> [w2353]
                          tunnel: w2338 -> [w2352]
                          tunnel: w2337 -> [w2351]
                          # "[HA] = C(buffer) x 10^pK /(10^pH + 10^pK)"
                          # "pIon"
                          n1020 = Subtract(x=w2354, y=w2355) -> (x-y=w2356:dbl)
                          n1021 = Power Of 10(x=w2351) -> (10^x=w2347:dbl)
                          n1022 = Divide(x=w2356, y=w2353) -> (x/y=w2345:dbl)
                          n1023 = Multiply(x=w2347, y=w2352) -> (x*y=w2350:dbl)
                          n1024 = Power Of 10(x=w2345) -> (10^x=w2348:dbl)
                          n1025 = Add(x=w2347, y=w2348) -> (x+y=w2349:dbl)
                          n1026 = Divide(x=w2350, y=w2349) -> (x/y=w2346:dbl)
                        }
                        n1027 = Insert Into Array(array=w2341, index (col)=w2336, new element=w2339) -> (w2340:dbl[][])  [unwired: 1 in]
                      }
                      n1028 = Unbundle(w2309) -> (w2321:string[], w2320:bool[])
                      n1029 = Replace Array Subset(array=w2320, new element=TRUE, index=15 ("Index")) -> (w2319:bool[])
                      n1030 = Bundle(w2321, w2319) -> (w2316:cluster{string[], bool[]})  [unwired: 1 in]
                      n1031 = local read "Corrected \ndistance ch2"() -> (w2335:dbl)
                      n1032 = local read "Diff. coeff. buffer ch2"() -> (w2334:dbl)
                      n1033 = Index Array(array=w2312, index (col)=13 ("disabled index (col)")) -> (element=w2314:dbl[])  [unwired: 1 in]
                      n1034 = for {
                        shift-right: [w2372] -> w2310
                        shift-left: w2322 -> [w2371]
                        tunnel: w2334 -> [w2362]
                        tunnel: w2335 -> [w2365]
                        tunnel: w2323 -> [w2361] mode=indexing
                        tunnel: w2314 -> [w2357] mode=indexing
                        # "J(Ion) x 10^9"
                        # "J(buffer) x 10^9"
                        # "dc / dx : mol m3 / m"
                        n1035 = Index Array(array=w2361, index=1 ("Deaktivierter Index (Spalte)")) -> (element=w2368:dbl)
                        n1036 = Index Array(array=w2361, index=0 ("Deaktivierter Index (Spalte)")) -> (element=w2367:dbl)
                        n1037 = Divide(x=w2365, y=1000000.0) -> (x/y=w2363:dbl)
                        n1038 = Subtract(x=w2368, y=w2367) -> (x-y=w2366:dbl)
                        n1039 = Divide(x=w2366, y=w2363) -> (x/y=w2358:dbl)
                        n1040 = Multiply(x=w2358, y=w2362) -> (x*y=w2360:dbl)
                        n1041 = Add(x=w2360, y=w2357) -> (x+y=w2359:dbl)
                        n1042 = Insert Into Array(array=w2371, new element=w2359) -> (w2372:dbl[])  [unwired: 1 in]
                      }
                      n1043 = Replace Array Subset(array=w2312, new element=w2310, index (col)=15 ("Deaktivierter Index (Spalte)")) -> (w2311:dbl[][])  [unwired: 1 in]
                    }
                  }
                  n1044 = Multiply(x="Zoom from end (Buffer corr. modul) ch2", y=-1.0) -> (x*y=w2240:dbl)
                  n1045 = Add(x="Zoom from start (Buffer corr. modul) ch2", y=w2240) -> (x+y=w2234:dbl)
                  n1046 = feedback #5() -> (w2236:dbl)  [unwired: 1 in]
                  n1047 = Greater Or Equal?(x=w2234, y=0.0) -> (x >= y?=w2235:bool)
                  n1048 = case shown="True" w2235 {
                    tunnel: "Zoom from start (Buffer corr. modul) ch2" -> [w2375 w2378]
                    tunnel: [w2374 w2378] -> w2225
                    tunnel: w2236 -> [w2374 w2380]
                    tunnel: "Zoom from end (Buffer corr. modul) ch2" -> [_ w2377]
                    tunnel: [w2375 w2378] -> w2241
                    tunnel: [w2373 w2376] -> w2242
                    tunnel: "Zoom from end (Buffer corr. modul) ch2" -> [w2373 w2376]
                    frame False {
                    }
                    frame True {
                      n1049 = Not Equal?(x=w2380, y=w2378) -> (x != y?=w2379:bool)
                      n1050 = case shown="False" w2379 {
                        tunnel: w2378 -> [_ w2382]
                        tunnel: w2377 -> [w2381 _]
                        frame False {
                          n1051 = local write "Zoom from start (Buffer corr. modul) ch2"(w2381) -> ()
                        }
                        frame True {
                          n1052 = local write "Zoom from end (Buffer corr. modul) ch2"(w2382) -> ()
                        }
                      }
                    }
                  }
                  n1053 = feedback-in #5(w2225) -> ()
                  n1054 = Array Size(array=w2219) -> (size(s)=w2251:i32)
                  n1055 = Divide(x=w2251, y=10) -> (x/y=w2252:dbl)
                  n1056 = Multiply(x=w2252, y="Bildlaufleiste 4") -> (x*y=w2254:dbl)
                  n1057 = Array Subset(array=w2219, index=w2254) -> (w2255:cluster{dbl, string}[])  [unwired: 1 in]
                  n1058 = Subtract(x=w2242, y=w2241) -> (x-y=w2237:dbl)
                  n1059 = for {
                    shift-right: [w2392] -> w2250
                    shift-left: "" -> [w2393]
                    tunnel: w2255 -> [w2391] mode=indexing
                    n1060 = Unbundle(w2391) -> (w2389:dbl, w2386:string)
                    n1061 = Divide(x=w2389, y=60.0) -> (x/y=w2387:dbl)
                    n1062 = Number To Fractional String(number=w2387, precision (6)=i16 2 ("Genauigkeit (6)")) -> (F-format string=w2385:string)  [unwired: 2 in]
                    n1063 = Concatenate Strings(w2393, w2385, "min. ,", w2386, "\r") -> (w2392:string)
                  }
                  "?" <- w2250
                  n1064 = Index Array(array=w2223, index (col)=0 ("Deaktivierter Index (Spalte)")) -> (element=w2233:dbl[])  [unwired: 1 in]
                  n1065 = Divide(x=w2241, y=100.0) -> (x/y=w2239:dbl)
                  n1066 = Divide(x=w2237, y=100.0) -> (x/y=w2238:dbl)
                  n1067 = Array Size(array=w2233) -> (size(s)=w2243:i32)
                  n1068 = Multiply(x=w2243, y=w2239) -> (x*y=w2246:dbl)
                  n1069 = Multiply(x=w2243, y=w2238) -> (x*y=w2244:dbl)
                  n1070 = Add(x=w2244, y=2.0) -> (x+y=w2245:dbl)
                  n1071 = Subtract(x=w2246, y=2.0) -> (x-y=w2247:dbl)
                  n1072 = Array Subset(array=w2223, index (row)=w2247, length (row)=w2245) -> (w2224:dbl[][])  [unwired: 2 in]
                  n1073 = Index Array(array=w2224, index (col)=0 ("disabled index (col)")) -> (element=w2260:dbl[])  [unwired: 1 in]
                  n1074 = Index Array(array=w2224, index (col)=15 ("disabled index (col)")) -> (element=w2258:dbl[])  [unwired: 1 in]
                  n1075 = stacked-sequence {
                    tunnel: w2260 -> [w2406]
                    tunnel: w2256 -> [w2400]
                    tunnel: w2258 -> [w2405]
                    tunnel: w2220 -> [w2401]
                    frame #0 {
                      n1076 = Array Max & Min(array=w2406) -> (max value=w2415:dbl, min value=w2414:dbl)  [unwired: 2 out]
                      n1077 = Divide(x="Range limit\nS2.4 2", y=2.0) -> (x/y=w2431:dbl)
                      n1078 = Divide(x="Range limit\nS2.4 2", y=2.05) -> (x/y=w2432:dbl)
                      n1079 = Add(x="Base line \nS2.4 2", y=w2431) -> (x+y=w2407:dbl)
                      n1080 = Subtract(x="Base line \nS2.4 2", y=w2431) -> (x-y=w2408:dbl)
                      n1081 = Subtract(x="Base line \nS2.4 2", y=w2432) -> (x-y=w2413:dbl)
                      n1082 = call "EventstoGraph (SubVI).vi"("Numerisch 2"=w2414, "Array 3"=w2400, "Numerisch"=w2415, "Array (Eingang)"=dbl[][] [], "Numerisch 3"=w2413) -> ("Array (Ausgang)"=w2417:dbl[][])  [unwired: 6 in]
                      n1083 = Array Max & Min(array=w2406) -> (max value=w2427:dbl, min value=w2428:dbl)  [unwired: 2 out]
                      n1084 = call "GraphLimit01.vi"("Numeric 2"=w2408, "Numeric"=w2407, "Array in"=w2405, "Array 3"=dbl[] []) -> ("Array out"=w2422:dbl[])  [unwired: 7 in]
                      n1085 = Build Array("Base line \nS2.4 2", "Base line \nS2.4 2") -> (w2424:dbl[])
                      n1086 = Build Array(w2427, w2428) -> (w2425:dbl[])
                      n1087 = Build Array(w2407, w2408) -> (w2426:dbl[])
                      n1088 = Index Array(array=w2417, index (col)=0 ("Index (Zeile)")) -> (element=w2418:dbl[])  [unwired: 1 in]
                      n1089 = Index Array(array=w2417, index (col)=1 ("Index (Zeile)")) -> (element=w2416:dbl[])  [unwired: 1 in]
                      n1090 = Bundle(w2425, w2426) -> (w2411:cluster{dbl[], dbl[]})  [unwired: 1 in]
                      n1091 = Bundle(w2425, w2424) -> (w2412:cluster{dbl[], dbl[]})  [unwired: 1 in]
                      n1092 = Bundle(w2406, "Array out"=w2422) -> (w2410:cluster{dbl[], "Array out":dbl[]})  [unwired: 1 in]
                      n1093 = Bundle("Array (Ausgang)"=w2418, "Array (Ausgang)"=w2416) -> (w2409:T17)  [unwired: 1 in]
                      n1094 = Build Array(w2412, w2411, w2410, w2409) -> (w2402:T18)
                      n1095 = case shown="True" w2401 {
                        tunnel: w2402 -> [_ w2433]
                        frame False {
                        }
                        frame True {
                          "Ion flux (buffer corr.) SISE channel 2" <- w2433
                        }
                      }
                    }
                  }
                }
              }
              n1096 = Equal?(x=w2146, y=u16 0) -> (x = y?=w2140:bool)
              n1097 = Or(x=w2134, y=w2140) -> (x .or. y?=w2139:bool)
              n1098 = Select(t=T9."Enabled" ("Disabled"), s=w2139, f=T9."Disabled and Grayed Out") -> (s? t:f=w2155:T9)
              n1099 = property on="Buffer species ch2" class="Bool (strict)"("DisabledEnum"=w2155) -> ()  [unwired: 2 in, 2 out]
              n1100 = Equal?(x=w2146, y=u16 1) -> (x = y?=w2137:bool)
              n1101 = Or(x=w2134, y=w2137) -> (x .or. y?=w2138:bool)
              n1102 = Select(t=T9."Enabled" ("Disabled"), s=w2138, f=T9."Disabled and Grayed Out") -> (s? t:f=w2151:T9)
              n1103 = property on="Buffer conc. ch2" class="Bool (strict)"("DisabledEnum"=w2151) -> ()  [unwired: 2 in, 2 out]
              n1104 = Equal?(x=w2146, y=u16 2) -> (x = y?=w2135:bool)
              n1105 = Or(x=w2134, y=w2135) -> (x .or. y?=w2136:bool)
              n1106 = Select(t=T9."Enabled" ("Disabled"), s=w2136, f=T9."Disabled and Grayed Out") -> (s? t:f=w2128:T9)
              n1107 = property on="Update graphs (buffer corr.) ch2" class="Bool (strict)"("DisabledEnum"=w2128) -> ()  [unwired: 2 in, 2 out]
            }
            frame "SISE channel 1, buffer corr." {
              n1108 = local read "Analysis method (Calibration window channel 1)"() -> (→"Tab Control":enum32{"Chem. potential", "Diff. gradient"})
              n1109 = local read "Buffer species ch1"() -> (w2443:bool)
              n1110 = local read "Buffer conc. ch1"() -> (w2444:bool)
              n1111 = Unbundle(w2440) -> (w2447:bool[])  [unwired: 1 out]
              n1112 = Index Array(array=w2439, index=0) -> (element=w2434:bool)
              n1113 = Index Array(array=w2447, index=12) -> (element=w2445:bool)
              n1114 = Build Array(w2443, w2444, w2445) -> (w2441:bool[])
              n1115 = for {
                shift-right: [w2486] -> w2436
                shift-left: w2442 -> [w2487]
                tunnel: w2441 -> [w2485] mode=indexing
                n1116 = case shown="True" w2485 {
                  tunnel: w2487 -> [_ w2489]
                  tunnel: [FALSE w2489] -> w2486
                  frame False {
                  }
                  frame True {
                  }
                }
              }
              "Update graphs (buffer corr.) ch1" <- w2436
              n1117 = Unbundle(w2454) -> (w2464:bool[])  [unwired: 1 out]
              n1118 = case shown="True" w2436 {
                tunnel: [0 w2482] -> w2435
                tunnel: w2434 -> [_ w2481]
                frame False {
                }
                frame True {
                  n1119 = case shown="False" w2481 {
                    tunnel: [2 1] -> w2482
                    frame False {
                    }
                    frame True {
                    }
                  }
                }
              }
              n1120 = Index Array(array=w2464, index=8 ("Index")) -> (element=w2462:bool)
              n1121 = Index Array(array=w2464, index=10 ("Index")) -> (element=w2463:bool)
              n1122 = And(x=w2462, y=w2463) -> (x .and. y?=w2455:bool)
              n1123 = case shown="\"Update graphs\"" "Module selection ch1 (buffer corr.)" {
                tunnel: [0 1 2] -> w2467
                tunnel: w2450 -> [w2496 w2525 w2563]
                tunnel: [w2496 w2525 w2561] -> w2453
                tunnel: w2452 -> [_ _ w2564]
                tunnel: [w2495 w2524 w2562] -> w2451
                tunnel: w2448 -> [_ _ w2536]
                tunnel: w2436 -> [_ _ w2532]
                tunnel: w2440 -> [w2495 w2524 w2531]
                tunnel: w2435 -> [_ _ w2530]
                frame "Buffer species", Default {
                  n1124 = case shown="\"none\", Default" "Select buffer ch1" {
                    tunnel: ["" "Mes" "Malate (pH 5)" "Citrate (pH 5)" "TRIS" "HEPES"] -> w2490
                    tunnel: [0.0 6.2 5.1 4.8 8.2 7.5] -> w2493
                    tunnel: [0.0 2.9 3.2 2.5 3.2 2.4] -> w2492
                    tunnel: [0.0 0.7 0.8 0.6 0.8 0.6] -> w2491
                    frame "none", Default {
                    }
                    frame "Mes" {
                    }
                    frame "Malate (pH 5)" {
                    }
                    frame "Citrate (pH 5)" {
                    }
                    frame "TRIS" {
                    }
                    frame "HEPES" {
                    }
                  }
                  "pKs ch1" <- w2493
                  "Buffer Mobilty ch1" <- w2492
                  "Diff. coeff. buffer ch1" <- w2491
                  n1125 = Not Equal?(x="", y=w2490) -> (x != y?=→"Buffer species ch1":bool)
                }
                frame "Buffer conc." {
                  n1126 = Not Equal To 0?(x="Buffer conc. ch1 (mM)") -> (x != 0?=→"Buffer conc. ch1":bool)
                }
                frame "Update graphs" {
                  n1127 = local read "Ion conc. ch1 (mM)"() -> (w2533:dbl)
                  n1128 = local read "pKs ch1"() -> (w2582:dbl)
                  n1129 = local read "Buffer conc. ch1 (mM)"() -> (w2581:dbl)
                  n1130 = local read "Buffer Mobilty ch1"() -> (w2579:dbl)
                  n1131 = local read "Ion mobilty ch1"() -> (w2580:dbl)
                  n1132 = local write "Zoom from start (Buffer corr. modul) ch2"("Zoom from start (Buffer corr. modul) ch1") -> ()
                  n1133 = local write "Zoom from end (Buffer corr. modul) ch2"("Zoom from end (Buffer corr. modul) ch1") -> ()
                  n1134 = for {
                    tunnel: w2564 -> [w2608] mode=indexing
                    shift-right: [w2610] -> w2565
                    shift-left: dbl[] [] -> [w2609]
                    n1135 = Unbundle(w2608) -> (w2605:dbl)  [unwired: 1 out]
                    n1136 = Divide(x=w2605, y=60.0) -> (x/y=w2606:dbl)
                    n1137 = Insert Into Array(array=w2609, new element=w2606) -> (w2610:dbl[])  [unwired: 1 in]
                  }
                  n1138 = case shown="1" w2530 {
                    tunnel: w2579 -> [_ w2665 _]
                    tunnel: w2580 -> [_ w2666 _]
                    tunnel: w2582 -> [_ w2663 w2706]
                    tunnel: w2581 -> [_ w2662 w2707]
                    tunnel: w2533 -> [_ w2654 _]
                    tunnel: w2531 -> [w2646 w2657 w2698]
                    tunnel: w2563 -> [w2645 w2649 w2693]
                    tunnel: [w2646 w2655 w2697] -> w2562
                    tunnel: [w2645 w2653 w2692] -> w2561
                    tunnel: dbl[] [] -> [_ w2647 w2704]
                    frame 0, Default {
                    }
                    frame 1 {
                      n1139 = Index Array(array=w2649, index (col)=12 ("Deaktivierter Index (Spalte)")) -> (element=w2648:dbl[])  [unwired: 1 in]
                      n1140 = Divide(x=w2665, y=w2666) -> (x/y=w2664:dbl)
                      n1141 = for {
                        tunnel: w2664 -> [w2675]
                        tunnel: w2663 -> [w2685]
                        tunnel: w2662 -> [w2679]
                        shift-right: [w2670] -> w2652
                        shift-left: w2647 -> [w2671]
                        tunnel: w2648 -> [w2669] mode=indexing
                        tunnel: w2654 -> [w2668]
                        n1142 = Multiply(x=w2668, y=0.001) -> (x*y=w2689:dbl)
                        n1143 = Multiply(x=w2679, y=0.001) -> (x*y=w2676:dbl)
                        n1144 = Logarithm Base 10(1:w2689) -> (0:w2688:dbl)
                        n1145 = Multiply(x=w2688, y=-1.0) -> (x*y=w2686:dbl)
                        n1146 = Power Of 10(x=w2686) -> (10^x=w2683:dbl)
                        n1147 = Power Of 10(x=w2685) -> (10^x=w2680:dbl)
                        n1148 = Add(x=w2683, y=w2680) -> (x+y=w2684:dbl)
                        n1149 = Divide(x=w2683, y=w2684) -> (x/y=w2682:dbl)
                        n1150 = Square(x=w2682) -> (x^2=w2681:dbl)
                        n1151 = Multiply(x=w2681, y=w2680) -> (x*y=w2677:dbl)
                        n1152 = Multiply(x=w2677, y=w2676) -> (x*y=w2674:dbl)
                        n1153 = Multiply(x=w2674, y=w2675) -> (x*y=w2673:dbl)
                        n1154 = Multiply(x=w2673, y=w2669) -> (x*y=w2672:dbl)
                        n1155 = Add(x=w2672, y=w2669) -> (x+y=w2667:dbl)
                        n1156 = Insert Into Array(array=w2671, new element=w2667) -> (w2670:dbl[])  [unwired: 1 in]
                      }
                      n1157 = Unbundle(w2657) -> (w2656:string[], w2660:bool[])
                      n1158 = Replace Array Subset(array=w2660, new element=TRUE, index=14 ("Index")) -> (w2661:bool[])
                      n1159 = Bundle(w2656, w2661) -> (w2655:cluster{string[], bool[]})  [unwired: 1 in]
                      n1160 = Replace Array Subset(array=w2649, new element=w2652, index (col)=14 ("Deaktivierter Index (Spalte)")) -> (w2653:dbl[][])  [unwired: 1 in]
                    }
                    frame 2 {
                      # "Diff. coeff. (x 10^9)"
                      n1161 = Index Array(array=w2693, index (col)=6 ("Deaktivierter Index (Spalte)")) -> (element=w2711:dbl[])  [unwired: 1 in]
                      n1162 = Index Array(array=w2693, index (col)=7 ("Deaktivierter Index (Spalte)")) -> (element=w2712:dbl[])  [unwired: 1 in]
                      n1163 = Build Array(w2711, w2712) -> (w2713:dbl[][])
                      n1164 = local read "Intercept ch1"() -> (w2714:dbl)
                      n1165 = local read "Slope ch1"() -> (w2715:dbl)
                      n1166 = for {
                        tunnel: w2713 -> [w2726] mode=indexing
                        tunnel: w2714 -> [w2725]
                        tunnel: w2715 -> [w2724]
                        shift-right: [w2722] -> w2705
                        shift-left: dbl[][] [] -> [w2723]
                        tunnel: w2707 -> [w2720]
                        tunnel: w2706 -> [w2719]
                        i -> [w2718]
                        n1167 = for {
                          tunnel: w2726 -> [w2736] mode=indexing
                          tunnel: [w2728] -> w2721 mode=indexing
                          tunnel: w2725 -> [w2737]
                          tunnel: w2724 -> [w2735]
                          tunnel: w2720 -> [w2734]
                          tunnel: w2719 -> [w2733]
                          # "[HA] = C(buffer) x 10^pK /(10^pH + 10^pK)"
                          # "pIon"
                          n1168 = Subtract(x=w2736, y=w2737) -> (x-y=w2738:dbl)
                          n1169 = Power Of 10(x=w2733) -> (10^x=w2729:dbl)
                          n1170 = Divide(x=w2738, y=w2735) -> (x/y=w2727:dbl)
                          n1171 = Multiply(x=w2729, y=w2734) -> (x*y=w2732:dbl)
                          n1172 = Power Of 10(x=w2727) -> (10^x=w2730:dbl)
                          n1173 = Add(x=w2729, y=w2730) -> (x+y=w2731:dbl)
                          n1174 = Divide(x=w2732, y=w2731) -> (x/y=w2728:dbl)
                        }
                        n1175 = Insert Into Array(array=w2723, index (col)=w2718, new element=w2721) -> (w2722:dbl[][])  [unwired: 1 in]
                      }
                      n1176 = Unbundle(w2698) -> (w2703:string[], w2702:bool[])
                      n1177 = Replace Array Subset(array=w2702, new element=TRUE, index=14 ("Index")) -> (w2701:bool[])
                      n1178 = Bundle(w2703, w2701) -> (w2697:cluster{string[], bool[]})  [unwired: 1 in]
                      n1179 = local read "Corrected \ndistance ch1"() -> (w2717:dbl)
                      n1180 = local read "Diff. coeff. buffer ch1"() -> (w2716:dbl)
                      n1181 = Index Array(array=w2693, index (col)=12 ("disabled index (col)")) -> (element=w2695:dbl[])  [unwired: 1 in]
                      n1182 = for {
                        shift-right: [w2754] -> w2691
                        shift-left: w2704 -> [w2753]
                        tunnel: w2716 -> [w2744]
                        tunnel: w2717 -> [w2747]
                        tunnel: w2705 -> [w2743] mode=indexing
                        tunnel: w2695 -> [w2739] mode=indexing
                        # "J(Ion) x 10^9"
                        # "J(buffer) x 10^9"
                        # "dc / dx : mol m3 / m"
                        n1183 = Index Array(array=w2743, index=1 ("Deaktivierter Index (Spalte)")) -> (element=w2750:dbl)
                        n1184 = Index Array(array=w2743, index=0 ("Deaktivierter Index (Spalte)")) -> (element=w2749:dbl)
                        n1185 = Divide(x=w2747, y=1000000.0) -> (x/y=w2745:dbl)
                        n1186 = Subtract(x=w2750, y=w2749) -> (x-y=w2748:dbl)
                        n1187 = Divide(x=w2748, y=w2745) -> (x/y=w2740:dbl)
                        n1188 = Multiply(x=w2740, y=w2744) -> (x*y=w2742:dbl)
                        n1189 = Add(x=w2742, y=w2739) -> (x+y=w2741:dbl)
                        n1190 = Insert Into Array(array=w2753, new element=w2741) -> (w2754:dbl[])  [unwired: 1 in]
                      }
                      n1191 = Replace Array Subset(array=w2693, new element=w2691, index (col)=14 ("Deaktivierter Index (Spalte)")) -> (w2692:dbl[][])  [unwired: 1 in]
                    }
                  }
                  n1192 = Multiply(x="Zoom from end (Buffer corr. modul) ch1", y=-1.0) -> (x*y=w2553:dbl)
                  n1193 = Add(x="Zoom from start (Buffer corr. modul) ch1", y=w2553) -> (x+y=w2547:dbl)
                  n1194 = feedback #6() -> (w2549:dbl)  [unwired: 1 in]
                  n1195 = Greater Or Equal?(x=w2547, y=0.0) -> (x >= y?=w2548:bool)
                  n1196 = case shown="True" w2548 {
                    tunnel: "Zoom from start (Buffer corr. modul) ch1" -> [w2586 w2589]
                    tunnel: [w2585 w2589] -> w2538
                    tunnel: w2549 -> [w2585 w2591]
                    tunnel: "Zoom from end (Buffer corr. modul) ch1" -> [_ w2588]
                    tunnel: [w2586 w2589] -> w2554
                    tunnel: [w2584 w2587] -> w2555
                    tunnel: "Zoom from end (Buffer corr. modul) ch1" -> [w2584 w2587]
                    frame False {
                    }
                    frame True {
                      n1197 = Not Equal?(x=w2591, y=w2589) -> (x != y?=w2590:bool)
                      n1198 = case shown="False" w2590 {
                        tunnel: w2589 -> [_ w2593]
                        tunnel: w2588 -> [w2592 _]
                        frame False {
                          n1199 = local write "Zoom from start (Buffer corr. modul) ch1"(w2592) -> ()
                        }
                        frame True {
                          n1200 = local write "Zoom from end (Buffer corr. modul) ch1"(w2593) -> ()
                        }
                      }
                    }
                  }
                  n1201 = feedback-in #6(w2538) -> ()
                  n1202 = Array Size(array=w2564) -> (size(s)=w2569:i32)
                  n1203 = Divide(x=w2569, y=10) -> (x/y=w2570:dbl)
                  n1204 = Multiply(x=w2570, y="Bildlaufleiste 3") -> (x*y=w2572:dbl)
                  n1205 = Array Subset(array=w2564, index=w2572) -> (w2573:cluster{dbl, string}[])  [unwired: 1 in]
                  n1206 = for {
                    shift-right: [w2603] -> w2568
                    shift-left: "" -> [w2604]
                    tunnel: w2573 -> [w2602] mode=indexing
                    n1207 = Unbundle(w2602) -> (w2600:dbl, w2597:string)
                    n1208 = Divide(x=w2600, y=60.0) -> (x/y=w2598:dbl)
                    n1209 = Number To Fractional String(number=w2598, precision (6)=i16 2 ("Genauigkeit (6)")) -> (F-format string=w2596:string)  [unwired: 2 in]
                    n1210 = Concatenate Strings(w2604, w2596, "min. ,", w2597, "\r") -> (w2603:string)
                  }
                  "?" <- w2568
                  n1211 = Subtract(x=w2555, y=w2554) -> (x-y=w2550:dbl)
                  n1212 = Index Array(array=w2536, index (col)=0 ("Deaktivierter Index (Spalte)")) -> (element=w2546:dbl[])  [unwired: 1 in]
                  n1213 = Divide(x=w2554, y=100.0) -> (x/y=w2552:dbl)
                  n1214 = Divide(x=w2550, y=100.0) -> (x/y=w2551:dbl)
                  n1215 = Array Size(array=w2546) -> (size(s)=w2556:i32)
                  n1216 = Multiply(x=w2556, y=w2552) -> (x*y=w2559:dbl)
                  n1217 = Multiply(x=w2556, y=w2551) -> (x*y=w2557:dbl)
                  n1218 = Add(x=w2557, y=2.0) -> (x+y=w2558:dbl)
                  n1219 = Subtract(x=w2559, y=2.0) -> (x-y=w2560:dbl)
                  n1220 = Array Subset(array=w2536, index (row)=w2560, length (row)=w2558) -> (w2537:dbl[][])  [unwired: 2 in]
                  n1221 = Index Array(array=w2537, index (col)=0 ("disabled index (col)")) -> (element=w2577:dbl[])  [unwired: 1 in]
                  n1222 = Index Array(array=w2537, index (col)=14 ("disabled index (col)")) -> (element=w2575:dbl[])  [unwired: 1 in]
                  n1223 = stacked-sequence {
                    tunnel: w2577 -> [w2617]
                    tunnel: w2565 -> [w2611]
                    tunnel: w2575 -> [w2616]
                    tunnel: w2532 -> [w2612]
                    frame #0 {
                      n1224 = Array Max & Min(array=w2617) -> (max value=w2626:dbl, min value=w2625:dbl)  [unwired: 2 out]
                      n1225 = Divide(x="Range limit\nS2.4 3", y=2.0) -> (x/y=w2642:dbl)
                      n1226 = Divide(x="Range limit\nS2.4 3", y=2.05) -> (x/y=w2643:dbl)
                      n1227 = Add(x="Base line \nS2.4 3", y=w2642) -> (x+y=w2618:dbl)
                      n1228 = Subtract(x="Base line \nS2.4 3", y=w2642) -> (x-y=w2619:dbl)
                      n1229 = Subtract(x="Base line \nS2.4 3", y=w2643) -> (x-y=w2624:dbl)
                      n1230 = call "EventstoGraph (SubVI).vi"("Numerisch 2"=w2625, "Array 3"=w2611, "Numerisch"=w2626, "Array (Eingang)"=dbl[][] [], "Numerisch 3"=w2624) -> ("Array (Ausgang)"=w2628:dbl[][])  [unwired: 6 in]
                      n1231 = Array Max & Min(array=w2617) -> (max value=w2638:dbl, min value=w2639:dbl)  [unwired: 2 out]
                      n1232 = call "GraphLimit01.vi"("Numeric 2"=w2619, "Numeric"=w2618, "Array in"=w2616, "Array 3"=dbl[] []) -> ("Array out"=w2633:dbl[])  [unwired: 7 in]
                      n1233 = Build Array("Base line \nS2.4 3", "Base line \nS2.4 3") -> (w2635:dbl[])
                      n1234 = Build Array(w2638, w2639) -> (w2636:dbl[])
                      n1235 = Build Array(w2618, w2619) -> (w2637:dbl[])
                      n1236 = Index Array(array=w2628, index (col)=0 ("Index (Zeile)")) -> (element=w2629:dbl[])  [unwired: 1 in]
                      n1237 = Index Array(array=w2628, index (col)=1 ("Index (Zeile)")) -> (element=w2627:dbl[])  [unwired: 1 in]
                      n1238 = Bundle(w2636, w2637) -> (w2622:cluster{dbl[], dbl[]})  [unwired: 1 in]
                      n1239 = Bundle(w2636, w2635) -> (w2623:cluster{dbl[], dbl[]})  [unwired: 1 in]
                      n1240 = Bundle(w2617, "Array out"=w2633) -> (w2621:cluster{dbl[], "Array out":dbl[]})  [unwired: 1 in]
                      n1241 = Bundle("Array (Ausgang)"=w2629, "Array (Ausgang)"=w2627) -> (w2620:T17)  [unwired: 1 in]
                      n1242 = Build Array(w2623, w2622, w2621, w2620) -> (w2613:T18)
                      n1243 = case shown="True" w2612 {
                        tunnel: w2613 -> [_ w2644]
                        frame False {
                        }
                        frame True {
                          "Ion flux (buffer corr.) SISE channel 1" <- w2644
                        }
                      }
                    }
                  }
                }
              }
              n1244 = Equal?(x=w2467, y=u16 0) -> (x = y?=w2461:bool)
              n1245 = Or(x=w2455, y=w2461) -> (x .or. y?=w2460:bool)
              n1246 = Select(t=T9."Enabled" ("Disabled"), s=w2460, f=T9."Disabled and Grayed Out") -> (s? t:f=w2476:T9)
              n1247 = property on="Buffer species ch1" class="Bool (strict)"("DisabledEnum"=w2476) -> ()  [unwired: 2 in, 2 out]
              n1248 = Equal?(x=w2467, y=u16 1) -> (x = y?=w2458:bool)
              n1249 = Or(x=w2455, y=w2458) -> (x .or. y?=w2459:bool)
              n1250 = Select(t=T9."Enabled" ("Disabled"), s=w2459, f=T9."Disabled and Grayed Out") -> (s? t:f=w2472:T9)
              n1251 = property on="Buffer conc. ch1" class="Bool (strict)"("DisabledEnum"=w2472) -> ()  [unwired: 2 in, 2 out]
              n1252 = Equal?(x=w2467, y=u16 2) -> (x = y?=w2456:bool)
              n1253 = Or(x=w2455, y=w2456) -> (x .or. y?=w2457:bool)
              n1254 = Select(t=T9."Enabled" ("Disabled"), s=w2457, f=T9."Disabled and Grayed Out") -> (s? t:f=w2449:T9)
              n1255 = property on="Update graphs (buffer corr.) ch1" class="Bool (strict)"("DisabledEnum"=w2449) -> ()  [unwired: 2 in, 2 out]
            }
          }
          n1256 = Unbundle(w2106) -> (w2099:bool[], w2098:dbl[][], w2100:dbl[], w2101:cluster{dbl, string}[])
        }
      }
    }
  }
